vi "MotorControlMina1.vi"() -> ()   [LabVIEW 2012]
uses:
  <vilib>/Utility/error.llb/DialogType.ctl
  <vilib>/DAQmx/create/channels.llb/DAQmx Create Channel (AO-Voltage-Basic).vi
  <vilib>/DAQmx/write.llb/DAQmx Write (Analog DBL 1Chan 1Samp).vi
  <vilib>/DAQmx/create/channels.llb/DAQmx Create Channel (DO-Digital Output).vi
  <vilib>/DAQmx/write.llb/DAQmx Write (Digital Bool 1Line 1Point).vi
  <vilib>/DAQmx/create/channels.llb/DAQmx Create Channel (AI-Voltage-Basic).vi
  <vilib>/DAQmx/configure/timing.llb/DAQmx Timing (Sample Clock).vi
  <vilib>/DAQmx/read.llb/DAQmx Read (Analog 2D DBL NChan NSamp).vi
  <vilib>/Analysis/baseanly.llb/Mean (DBL).vi
  <vilib>/DAQmx/read.llb/DAQmx Read (Digital Bool 1Line 1Point).vi
  <vilib>/Utility/inputDevices.llb/joystickAcquire.vi
  <vilib>/Utility/inputDevices.llb/closeJoystick.vi
  <vilib>/Analysis/NI_AALBase.lvlib
panel:
  in  "Offset (V)":dbl=5.0
  out "Oscillate Mirror? 2":bool
  out "Mirror Voltage":dbl
  in  "Oscillate Mirror?":bool
  in  "Period (s)":i32=1
  in  "Amplitude (V)":dbl=4.0
  in  "Stop":bool
  in  "ForceExtInitConst":dbl[](array[numeric])
  out "InstrumentMode":T1(ring)=enum."Shutdown"
  in  "XMotorRef":refnum<k7>(container)
  in  "YMotorRef":refnum<k7>(container)
  in  "ZMotorRef":refnum<k7>(container)
  out "JoystOffset":T2={"XOffset"=-99999, "YOffset"=-99999, "ZOffset"=-99999}
  out "RelJoyPos":T3
  in  "InterfaceSelector":T4(tab)
  in  "GoToTopDisp":bool
  in  "GoToBottDisp":bool
  in  "GoToExpLoc":bool
  in  "SaveTopDisp":bool
  in  "SaveBottDisp":bool
  in  "SaveExpLoc":bool
  out "Top Dispenser":T5={"X Pos (mm)"=0.5532008, "Y Pos (mm)"=0.030929338, "Z Pos (mm)"=0.77973413} {"Y Pos (mm)" format="%.3f"; "Z Pos (mm)" format="%.3f"; "X Pos (mm)" format="%.3f"}
  out "Bottom Dispenser":T5={"X Pos (mm)"=0.600309, "Y Pos (mm)"=-1.1540928, "Z Pos (mm)"=0.7938141} {"Y Pos (mm)" format="%.3f"; "Z Pos (mm)" format="%.3f"; "X Pos (mm)" format="%.3f"}
  out "Experiment Region":T5={"X Pos (mm)"=1.4278219, "Y Pos (mm)"=-0.74810517, "Z Pos (mm)"=0.7938141} {"Y Pos (mm)" format="%.3f"; "Z Pos (mm)" format="%.3f"; "X Pos (mm)" format="%.3f"}
  in  "PreviewPanel":T6(tab)
  out "Diagnostic Display":cluster{dbl, dbl}(graph)={100.78259213882863, 10.649843481998925}
  out "VertReading":dbl=0.0051513671875 format="%.3f"
  out "HorizReading":dbl=0.00535888671875 format="%.3f"
  out "QPD B \n(Steerable Trap)":T7={"Horizontal Voltage (V)"=-0.009930419921875, "Vertical Voltage (V)"=-0.077978515625, "Sum Voltage (V)"=-0.056793212890625, "Horizontal Signal (NormV)"=0.17485222998387961, "Vertical Signal (NormV)"=1.3730252552391187} {"Vertical Signal (NormV)" format="%.4f"; "Horizontal Signal (NormV)" format="%#.4f"; "Sum Voltage (V)" format="%.4f"; "Vertical Voltage (V)" format="%.4f"; "Horizontal Voltage (V)" format="%.4f"}
  out "QPD A \n(Fixed Trap)":T7={"Horizontal Voltage (V)"=-0.151220703125, "Vertical Voltage (V)"=-0.02420654296875, "Sum Voltage (V)"=-0.1012939453125, "Horizontal Signal (NormV)"=1.4928898529766208, "Vertical Signal (NormV)"=0.23897324656543747} {"Vertical Signal (NormV)" format="%.4f"; "Horizontal Signal (NormV)" format="%.4f"; "Sum Voltage (V)" format="%.4f"; "Vertical Voltage (V)" format="%.4f"; "Horizontal Voltage (V)" format="%.4f"}
  in  "PreviewDataAcquision":T8={"Sampling Freq (Hz)"=2500.0, "#Samples Averaged"=50}
  in  "Trap A (Steerable)  Params":T9={"X Stiff. (pN/nm)"=0.056, "X Alpha (nm/NV)"=976.0, "X Offset (NV)"=-0.02, "Y Stiff. (pN/nm)"=0.056, "Y Alpha (nm/NV)"=976.0, "Y Offset (NV)"=0.008}
  in  "Trap B (Fixed)  Params":T9={"X Stiff. (pN/nm)"=0.063, "X Alpha (nm/NV)"=1056.0, "X Offset (NV)"=-0.022, "Y Stiff. (pN/nm)"=0.063, "Y Alpha (nm/NV)"=1056.0, "Y Offset (NV)"=-0.013}
  in  "Z Motor Settings":T10={"Joyst Min Signal"=10.0, "Joyst Max Signal"=30000.0, "Vmax (mm/s)"=0.005, "Acc (mm/s/s)"=0.2, "+ JoystDirection"=2, "- JoystDirection"=1} {"Acc (mm/s/s)" format="%#.3f"; "Vmax (mm/s)" format="%#.3f"}
  in  "Y Motor Settings":T10={"Joyst Min Signal"=10.0, "Joyst Max Signal"=20000.0, "Vmax (mm/s)"=0.03, "Acc (mm/s/s)"=0.5, "+ JoystDirection"=1, "- JoystDirection"=2} {"Acc (mm/s/s)" format="%#.3f"; "Vmax (mm/s)" format="%#.3f"}
  in  "X Motor Settings":T10={"Joyst Min Signal"=10.0, "Joyst Max Signal"=20000.0, "Vmax (mm/s)"=0.03, "Acc (mm/s/s)"=0.5, "+ JoystDirection"=2, "- JoystDirection"=1} {"Acc (mm/s/s)" format="%#.3f"; "Vmax (mm/s)" format="%#.3f"}
  in  "Motor Cruise Param":T11={"X Acc (mm/s^2)"=0.3, "X Vmax (mm/s)"=0.3, "Y Acc (mm/s^2)"=0.3, "Y Vmax (mm/s)"=0.3, "Z Acc (mm/s^2)"=0.1, "Z Vmax (mm/s)"=0.1}
  in  "Motor Limits":T12={"XMin"=-0.8, "XMax"=3.0, "YMin"=-2.0, "YMax"=2.0, "ZMin"=0.0, "ZMax"=2.0}
  in  "Steerable Mirror Calibration":T13={"Hor. Scaling (nm/V)"=760.0, "Vert. Scaling (nm/V)"=760.0, "Hor. Mirr. Offset (V)"=0.0, "Vert. Mirr. Offset (V)"=0.0}
  in  "SampRate/Ch":dbl=25000.0
  in  "AveragingWindow":i32=10
  in  "Steerable \nTrap\n(F12)":bool
  in  "Fixed\nTrap\n(F11)":bool
  in  "BMHorizSlider(V)":dbl(slide)=0.0059356689453125 scale=0.0..10.0
  in  "BMSliderVert(V)":dbl(slide)=0.005126953125 scale=0.0..10.0 scale format="%#_3f"
  in  "Align Traps Vertically":bool
  in  "MaxHorizontalTrapSeparation":bool
  out "X Motor State":T14={"Direction"=0, "Vel (mm/s)"=0.0, "IsActive?"=FALSE, "Pos (mm)"=-0.2957381} {"Pos (mm)" format="%#.3f"; "Vel (mm/s)" format="%#.4f"}
  out "Y Motor State":T14={"Direction"=0, "Vel (mm/s)"=0.0, "IsActive?"=FALSE, "Pos (mm)"=0.016441232} {"Pos (mm)" format="%#.3f"; "Vel (mm/s)" format="%#.4f"}
  out "Z Motor State":T14={"Direction"=0, "Vel (mm/s)"=0.0, "IsActive?"=FALSE, "Pos (mm)"=-0.26253498} {"Pos (mm)" format="%#.3f"; "Vel (mm/s)" format="%#.4f"}
  out "Move Z":bool
  out "Move XY":bool
  in  "MotorLoopDelay":u32=100
  out "Waveform Chart":T15(graph)={"[0]"=0.0023651123, "[1]"=0.0025787354, "[2]"=0.0019226074, "[3]"=0.0018310547, "[4]"=0.006378174, "[5]"=0.004486084, "[6]"=0.0008239746, "[7]"=0.0034179688}
  in  "StopPassiveMode":bool caption="stop"
  out "LowFreqFilePath":string="C:\\Data\\091813\\091813N02.psv"
  in  "PMVertSlider(V)":dbl(slide)=0.005145263671875 scale=0.0..10.0 scale format="%#_3f"
  in  "PMHorizSlider(V)":dbl(slide)=0.0045623779296875 scale=2.0..10.0
  out "IsPassiveModeActive?":bool caption="stop"
  out "Force TrapA":cluster{dbl, dbl}[](graph)=[{nan, nan}, {nan, nan}, {nan, nan}, {nan, nan}, {nan, nan}, {nan, nan}, {nan, nan}, {nan, nan}, {nan, nan}, {nan, nan}, {nan, nan}, {nan, nan}, {nan, nan}, {nan, nan}, {nan, nan}, {nan, nan}, {nan, nan}, {nan, nan}, {nan, nan}, {nan, nan}, {nan, nan}, {nan, nan}, {nan, nan}, {nan, nan}, {nan, nan}, {nan, nan}, {nan, nan}, {nan, nan}, {nan, nan}, {nan, nan}, {nan, nan}, {nan, nan}, {nan, nan}, {nan, nan}, {nan, nan}, {nan, nan}, {nan, nan}, {nan, nan}, {nan, nan}, {nan, nan}, {nan, nan}, {nan, nan}, {nan, nan}, {nan, nan}, {nan, nan}, {nan, nan}, {nan, nan}, {nan, nan}, {nan, nan}, {nan, nan}, {nan, nan}, {nan, nan}, {nan, nan}, {nan, nan}, {nan, nan}, {nan, nan}, {nan, nan}, {nan, nan}, {nan, nan}, {nan, nan}, {nan, nan}, {nan, nan}, {nan, nan}, {nan, nan}, {nan, nan}, {nan, nan}, {nan, nan}, {nan, nan}, {nan, nan}, {nan, nan}, {nan, nan}, {nan, nan}, {nan, nan}, {nan, nan}, {nan, nan}, {nan, nan}, {nan, nan}, {nan, nan}, {nan, nan}, {nan, nan}, {nan, nan}, {nan, nan}, {nan, nan}, {nan, nan}, {nan, nan}, {nan, nan}, {nan, nan}, {nan, nan}, {nan, nan}, {nan, nan}, {nan, nan}, {nan, nan}, {nan, nan}, {nan, nan}, {nan, nan}, {nan, nan}, {nan, nan}, {nan, nan}, {nan, nan}, {nan, nan}, {nan, nan}, {nan, nan}, {nan, nan}, {nan, nan}, {nan, nan}, {nan, nan}, {nan, nan}, {nan, nan}, {nan, nan}, {nan, nan}, {nan, nan}, {nan, nan}, {nan, nan}, {nan, nan}, {nan, nan}, {nan, nan}, {nan, nan}, {nan, nan}, {nan, nan}, {nan, nan}, {nan, nan}, {nan, nan}, {nan, nan}, {nan, nan}, {nan, nan}, {nan, nan}, {nan, nan}, {nan, nan}, {nan, nan}, {nan, nan}, {nan, nan}, {nan, nan}, {nan, nan}, {nan, nan}, {nan, nan}, {nan, nan}, {nan, nan}, {nan, nan}, {nan, nan}, {nan, nan}, {nan, nan}, {nan, nan}, {nan, nan}, {nan, nan}, {nan, nan}, {nan, nan}, {nan, nan}, {nan, nan}, {nan, nan}, {nan, nan}, {nan, nan}, {nan, nan}, {nan, nan}, {nan, nan}, {nan, nan}, {nan, nan}, {nan, nan}, {nan, nan}, {nan, nan}, {nan, nan}, {nan, nan}, {nan, nan}, {nan, nan}, {nan, nan}, {nan, nan}, {nan, nan}, {nan, nan}, {nan, nan}, {nan, nan}, {nan, nan}, {nan, nan}, {nan, nan}, {nan, nan}, {nan, nan}, {nan, nan}, {nan, nan}, {nan, nan}, {nan, nan}, {nan, nan}, {nan, nan}, {nan, nan}, {nan, nan}, {nan, nan}, {nan, nan}, {nan, nan}, {nan, nan}, {nan, nan}, {nan, nan}, {nan, nan}, {nan, nan}, {nan, nan}, {nan, nan}, {nan, nan}, {nan, nan}, {nan, nan}, {nan, nan}, {nan, nan}, {nan, nan}, {nan, nan}, {nan, nan}, {nan, nan}, {nan, nan}, {nan, nan}, {nan, nan}, {nan, nan}, {nan, nan}, {nan, nan}, {nan, nan}, {nan, nan}, {nan, nan}, {nan, nan}, {nan, nan}, {nan, nan}, {nan, nan}, {nan, nan}, {nan, nan}, {nan, nan}, {nan, nan}, {nan, nan}, {nan, nan}, {nan, nan}, {nan, nan}, {nan, nan}, {nan, nan}, {nan, nan}, {nan, nan}, {nan, nan}, {nan, nan}, {nan, nan}, {nan, nan}, {nan, nan}, {nan, nan}, {nan, nan}, {nan, nan}, {nan, nan}, {nan, nan}, {nan, nan}, {nan, nan}, {nan, nan}, {nan, nan}, {nan, nan}, {nan, nan}, {nan, nan}, {nan, nan}, {nan, nan}, {nan, nan}, {nan, nan}, {nan, nan}, {nan, nan}, {nan, nan}, {nan, nan}, {nan, nan}, {nan, nan}, {nan, nan}, {nan, nan}, {nan, nan}, {nan, nan}, {nan, nan}, {nan, nan}, {nan, nan}, {nan, nan}, {nan, nan}, {nan, nan}, {nan, nan}, {nan, nan}, {nan, nan}, {nan, nan}, {nan, nan}, {nan, nan}, {nan, nan}, {nan, nan}, {nan, nan}, {nan, nan}, {nan, nan}, {nan, nan}, {nan, nan}, {nan, nan}, {nan, nan}, {nan, nan}, {nan, nan}, {nan, nan}, {nan, nan}, {nan, nan}, {nan, nan}, {nan, nan}, {nan, nan}, {nan, nan}, {nan, nan}, {nan, nan}, {nan, nan}, {nan, nan}, {nan, nan}, {nan, nan}, {nan, nan}, {nan, nan}, {nan, nan}, {nan, nan}, {nan, nan}, {nan, nan}, {nan, nan}, {nan, nan}, {nan, nan}, {nan, nan}, {nan, nan}, {nan, nan}, {nan, nan}, {nan, nan}, {nan, nan}, {nan, nan}, {nan, nan}, {nan, nan}, {nan, nan}, {nan, nan}, {nan, nan}, {nan, nan}, {nan, nan}, {nan, nan}, {nan, nan}, {nan, nan}, {nan, nan}, {nan, nan}, {nan, nan}, {nan, nan}, {nan, nan}, {nan, nan}, {nan, nan}, {nan, nan}, {nan, nan}, {nan, nan}, {nan, nan}, {nan, nan}, {nan, nan}, {nan, nan}, {nan, nan}, {nan, nan}, {nan, nan}, {nan, nan}, {nan, nan}, {nan, nan}, {nan, nan}, {nan, nan}, {nan, nan}, {nan, nan}, {nan, nan}, {nan, nan}, {nan, nan}, {nan, nan}, {nan, nan}, {nan, nan}, {nan, nan}, {nan, nan}, {nan, nan}, {nan, nan}, {nan, nan}, {nan, nan}, {nan, nan}, {nan, nan}, {nan, nan}, {nan, nan}, {nan, nan}, {nan, nan}, {nan, nan}, {nan, nan}, {nan, nan}, {nan, nan}, {nan, nan}, {nan, nan}, {nan, nan}, {nan, nan}, {nan, nan}, {nan, nan}, {nan, nan}, {nan, nan}, {nan, nan}, {nan, nan}, {nan, nan}, {nan, nan}, {nan, nan}, {nan, nan}, {nan, nan}, {nan, nan}, {nan, nan}, {nan, nan}, {nan, nan}, {nan, nan}, {nan, nan}, {nan, nan}, {nan, nan}, {nan, nan}, {nan, nan}, {nan, nan}, {nan, nan}, {nan, nan}, {nan, nan}, {nan, nan}, {nan, nan}, {nan, nan}, {nan, nan}, {nan, nan}, {nan, nan}, {nan, nan}, {nan, nan}, {nan, nan}, {nan, nan}, {nan, nan}, {nan, nan}, {nan, nan}, {nan, nan}, {nan, nan}, {nan, nan}, {nan, nan}, {nan, nan}, {nan, nan}, {nan, nan}, {nan, nan}, {nan, nan}, {nan, nan}, {nan, nan}, {nan, nan}, {nan, nan}, {nan, nan}, {nan, nan}, {nan, nan}, {nan, nan}, {nan, nan}, {nan, nan}, {nan, nan}, {nan, nan}, {nan, nan}, {nan, nan}, {nan, nan}, {nan, nan}, {nan, nan}, {nan, nan}, {nan, nan}, {nan, nan}, {nan, nan}, {nan, nan}, {nan, nan}, {nan, nan}, {nan, nan}, {nan, nan}, {nan, nan}, {nan, nan}, {nan, nan}, {nan, nan}, {nan, nan}, {nan, nan}, {nan, nan}, {nan, nan}, {nan, nan}, {nan, nan}, {nan, nan}, {nan, nan}, {nan, nan}, {nan, nan}, {nan, nan}, {nan, nan}, {nan, nan}, {nan, nan}, {nan, nan}, {nan, nan}, {nan, nan}, {nan, nan}, {nan, nan}, {nan, nan}, {nan, nan}, {nan, nan}, {nan, nan}, {nan, nan}, {nan, nan}, {nan, nan}, {nan, nan}, {nan, nan}, {nan, nan}, {nan, nan}, {nan, nan}, {nan, nan}, {nan, nan}, {nan, nan}, {nan, nan}, {nan, nan}, {nan, nan}, {nan, nan}, {nan, nan}, {nan, nan}, {nan, nan}, {nan, nan}, {nan, nan}, {nan, nan}, {nan, nan}, {nan, nan}, {nan, nan}, {nan, nan}, {nan, nan}, {nan, nan}, {nan, nan}, {nan, nan}, {nan, nan}, {nan, nan}, {nan, nan}, {nan, nan}, {nan, nan}, {nan, nan}, {nan, nan}, {nan, nan}, {nan, nan}, {nan, nan}, {nan, nan}, {nan, nan}, {nan, nan}, {nan, nan}, {nan, nan}, {nan, nan}, {nan, nan}, {nan, nan}, {nan, nan}, {nan, nan}, {nan, nan}, {nan, nan}, {nan, nan}, {nan, nan}, {nan, nan}, {nan, nan}, {nan, nan}, {nan, nan}, {nan, nan}, {nan, nan}, {nan, nan}, {nan, nan}, {nan, nan}, {nan, nan}, {nan, nan}, {nan, nan}, {nan, nan}, {nan, nan}, {nan, nan}, {nan, nan}, {nan, nan}, {nan, nan}, {nan, nan}, {nan, nan}, {nan, nan}, {nan, nan}, {nan, nan}, {nan, nan}, {nan, nan}, {nan, nan}, {nan, nan}, {nan, nan}, {nan, nan}, {nan, nan}, {nan, nan}, {nan, nan}, {nan, nan}, {nan, nan}, {nan, nan}, {nan, nan}, {nan, nan}, {nan, nan}, {nan, nan}, {nan, nan}, {nan, nan}, {nan, nan}, {nan, nan}, {nan, nan}, {nan, nan}, {nan, nan}, {nan, nan}, {nan, nan}, {nan, nan}, {nan, nan}, {nan, nan}, {nan, nan}, {nan, nan}, {nan, nan}, {nan, nan}, {nan, nan}, {nan, nan}, {nan, nan}, {nan, nan}, {nan, nan}, {nan, nan}, {nan, nan}, {nan, nan}, {nan, nan}, {nan, nan}, {nan, nan}, {nan, nan}, {nan, nan}, {nan, nan}, {nan, nan}, {nan, nan}, {nan, nan}, {nan, nan}, {nan, nan}, {nan, nan}, {nan, nan}, {nan, nan}, {nan, nan}, {nan, nan}, {nan, nan}, {nan, nan}, {nan, nan}, {nan, nan}, {nan, nan}, {nan, nan}, {nan, nan}, {nan, nan}, {nan, nan}, {nan, nan}, {nan, nan}, {nan, nan}, {nan, nan}, {nan, nan}, {nan, nan}, {nan, nan}, {nan, nan}, {nan, nan}, {nan, nan}, {nan, nan}, {nan, nan}, {nan, nan}, {nan, nan}, {nan, nan}, {nan, nan}, {nan, nan}, {nan, nan}, {nan, nan}, {nan, nan}, {nan, nan}, {nan, nan}, {nan, nan}, {nan, nan}, {nan, nan}, {nan, nan}, {nan, nan}, {nan, nan}, {nan, nan}, {nan, nan}, {nan, nan}, {nan, nan}, {nan, nan}, {nan, nan}, {nan, nan}, {nan, nan}, {nan, nan}, {nan, nan}, {nan, nan}, {nan, nan}, {nan, nan}, {nan, nan}, {nan, nan}, {nan, nan}, {nan, nan}, {nan, nan}, {nan, nan}, {nan, nan}, {nan, nan}, {nan, nan}, {nan, nan}, {nan, nan}, {nan, nan}, {nan, nan}, {nan, nan}, {nan, nan}, {nan, nan}, {nan, nan}, {nan, nan}, {nan, nan}, {nan, nan}, {nan, nan}, {nan, nan}, {nan, nan}, {nan, nan}, {nan, nan}, {nan, nan}, {nan, nan}, {nan, nan}, {nan, nan}, {nan, nan}, {nan, nan}, {nan, nan}, {nan, nan}, {nan, nan}, {nan, nan}, {nan, nan}, {nan, nan}, {nan, nan}, {nan, nan}, {nan, nan}, {nan, nan}, {nan, nan}, {nan, nan}, {nan, nan}, {nan, nan}, {nan, nan}, {nan, nan}, {nan, nan}, {nan, nan}, {nan, nan}, {nan, nan}, {nan, nan}, {nan, nan}, {nan, nan}, {nan, nan}, {nan, nan}, {nan, nan}, {nan, nan}, {nan, nan}, {nan, nan}, {nan, nan}, {nan, nan}, {nan, nan}, {nan, nan}, {nan, nan}, {nan, nan}, {nan, nan}, {nan, nan}, {nan, nan}, {nan, nan}, {nan, nan}, {nan, nan}, {nan, nan}, {nan, nan}, {nan, nan}, {nan, nan}, {nan, nan}, {nan, nan}, {nan, nan}, {nan, nan}, {nan, nan}, {nan, nan}, {nan, nan}, {nan, nan}, {nan, nan}, {nan, nan}, {nan, nan}, {nan, nan}, {nan, nan}, {nan, nan}, {nan, nan}, {nan, nan}, {nan, nan}, {nan, nan}, {nan, nan}, {nan, nan}, {nan, nan}, {nan, nan}, {nan, nan}, {nan, nan}, {nan, nan}, {nan, nan}, {nan, nan}, {nan, nan}, {nan, nan}, {nan, nan}, {nan, nan}, {nan, nan}, {nan, nan}, {nan, nan}, {nan, nan}, {nan, nan}, {nan, nan}, {nan, nan}, {nan, nan}, {nan, nan}, {nan, nan}, {nan, nan}, {nan, nan}, {nan, nan}, {nan, nan}, {nan, nan}, {nan, nan}, {nan, nan}, {nan, nan}, {nan, nan}, {nan, nan}, {nan, nan}, {nan, nan}, {nan, nan}, {nan, nan}, {nan, nan}, {nan, nan}, {nan, nan}, {nan, nan}, {nan, nan}, {nan, nan}, {nan, nan}, {nan, nan}, {nan, nan}, {nan, nan}, {nan, nan}, {nan, nan}, {nan, nan}, {nan, nan}, {nan, nan}, {nan, nan}, {nan, nan}, {nan, nan}, {nan, nan}, {nan, nan}, {nan, nan}, {nan, nan}, {nan, nan}, {nan, nan}, {nan, nan}, {nan, nan}, {nan, nan}, {nan, nan}, {nan, nan}, {nan, nan}, {nan, nan}, {nan, nan}, {nan, nan}, {nan, nan}, {nan, nan}, {nan, nan}, {nan, nan}, {nan, nan}, {nan, nan}, {nan, nan}, {nan, nan}, {nan, nan}, {nan, nan}, {nan, nan}, {nan, nan}, {nan, nan}, {nan, nan}, {nan, nan}, {nan, nan}, {nan, nan}, {nan, nan}, {nan, nan}, {nan, nan}, {nan, nan}, {nan, nan}, {nan, nan}, {nan, nan}, {nan, nan}, {nan, nan}, {nan, nan}, {nan, nan}, {nan, nan}, {nan, nan}, {nan, nan}, {nan, nan}, {nan, nan}, {nan, nan}, {nan, nan}, {nan, nan}, {nan, nan}, {nan, nan}, {nan, nan}, {nan, nan}, {nan, nan}, {nan, nan}, {nan, nan}, {nan, nan}, {nan, nan}, {nan, nan}, {nan, nan}, {nan, nan}, {nan, nan}, {nan, nan}, {nan, nan}, {nan, nan}, {nan, nan}, {nan, nan}, {nan, nan}, {nan, nan}, {nan, nan}, {nan, nan}, {nan, nan}, {nan, nan}, {nan, nan}, {nan, nan}, {nan, nan}, {nan, nan}, {nan, nan}, {nan, nan}, {nan, nan}, {nan, nan}, {nan, nan}, {nan, nan}, {nan, nan}, {nan, nan}, {nan, nan}, {nan, nan}, {nan, nan}, {nan, nan}, {nan, nan}, {nan, nan}, {nan, nan}, {nan, nan}, {nan, nan}, {nan, nan}, {nan, nan}, {nan, nan}, {nan, nan}, {nan, nan}, {nan, nan}, {nan, nan}, {nan, nan}, {nan, nan}, {nan, nan}, {nan, nan}, {nan, nan}, {nan, nan}, {nan, nan}, {nan, nan}, {nan, nan}, {nan, nan}, {nan, nan}, {nan, nan}, {nan, nan}, {nan, nan}, {nan, nan}, {nan, nan}, {nan, nan}, {nan, nan}, {nan, nan}, {nan, nan}, {nan, nan}, {nan, nan}, {nan, nan}, {nan, nan}, {nan, nan}, {nan, nan}, {nan, nan}, {nan, nan}, {nan, nan}, {nan, nan}, {nan, nan}, {nan, nan}, {nan, nan}, {nan, nan}, {nan, nan}, {nan, nan}, {nan, nan}, {nan, nan}, {nan, nan}, {nan, nan}, {nan, nan}, {nan, nan}, {nan, nan}, {nan, nan}, {nan, nan}, {nan, nan}, {nan, nan}, {nan, nan}, {nan, nan}, {nan, nan}, {nan, nan}, {nan, nan}, {nan, nan}, {nan, nan}, {nan, nan}, {nan, nan}, {nan, nan}, {nan, nan}, {nan, nan}, {nan, nan}, {nan, nan}, {nan, nan}, {nan, nan}, {nan, nan}, {nan, nan}, {nan, nan}, {nan, nan}, {nan, nan}, {nan, nan}, {nan, nan}, {nan, nan}, {nan, nan}, {nan, nan}, {nan, nan}, {nan, nan}, {nan, nan}, {nan, nan}, {nan, nan}, {nan, nan}, {nan, nan}, {nan, nan}, {nan, nan}, {nan, nan}, {nan, nan}, {nan, nan}, {nan, nan}, {nan, nan}, {nan, nan}, {nan, nan}, {nan, nan}, {nan, nan}, {nan, nan}, {nan, nan}, {nan, nan}, {nan, nan}, {nan, nan}, {nan, nan}]
  out "Noise-Ext":cluster{dbl, dbl}[](graph)=[{nan, -0.0}, {nan, -0.0}, {nan, -0.0}, {nan, -0.0}, {nan, -0.0}, {nan, -0.0}, {nan, -0.0}, {nan, -0.0}, {nan, -0.0}, {nan, -0.0}, {nan, -0.0}, {nan, -0.0}, {nan, -0.0}, {nan, -0.0}, {nan, -0.0}, {nan, -0.0}, {nan, -0.0}, {nan, -0.0}, {nan, -0.0}, {nan, -0.0}, {nan, -0.0}, {nan, -0.0}, {nan, -0.0}, {nan, -0.0}, {nan, -0.0}, {nan, -0.0}, {nan, -0.0}, {nan, -0.0}, {nan, -0.0}, {nan, -0.0}, {nan, -0.0}, {nan, -0.0}, {nan, -0.0}, {nan, -0.0}, {nan, -0.0}, {nan, -0.0}, {nan, -0.0}, {nan, -0.0}, {nan, -0.0}, {nan, -0.0}, {nan, -0.0}, {nan, -0.0}, {nan, -0.0}, {nan, -0.0}, {nan, -0.0}, {nan, -0.0}, {nan, -0.0}, {nan, -0.0}, {nan, -0.0}, {nan, -0.0}, {nan, -0.0}, {nan, -0.0}, {nan, -0.0}, {nan, -0.0}, {nan, -0.0}, {nan, -0.0}, {nan, -0.0}, {nan, -0.0}, {nan, -0.0}, {nan, -0.0}, {nan, -0.0}, {nan, -0.0}, {nan, -0.0}, {nan, -0.0}, {nan, -0.0}, {nan, -0.0}, {nan, -0.0}, {nan, -0.0}, {nan, -0.0}, {nan, -0.0}, {nan, -0.0}, {nan, -0.0}, {nan, -0.0}, {nan, -0.0}, {nan, -0.0}, {nan, -0.0}, {nan, -0.0}, {nan, -0.0}, {nan, -0.0}, {nan, -0.0}, {nan, -0.0}, {nan, -0.0}, {nan, -0.0}, {nan, -0.0}, {nan, -0.0}, {nan, -0.0}, {nan, -0.0}, {nan, -0.0}, {nan, -0.0}, {nan, -0.0}, {nan, -0.0}, {nan, -0.0}, {nan, -0.0}, {nan, -0.0}, {nan, -0.0}, {nan, -0.0}, {nan, -0.0}, {nan, -0.0}, {nan, -0.0}, {nan, -0.0}, {nan, -0.0}, {nan, -0.0}, {nan, -0.0}, {nan, -0.0}, {nan, -0.0}, {nan, -0.0}, {nan, -0.0}, {nan, -0.0}, {nan, -0.0}, {nan, -0.0}, {nan, -0.0}, {nan, -0.0}, {nan, -0.0}, {nan, -0.0}, {nan, -0.0}, {nan, -0.0}, {nan, -0.0}, {nan, -0.0}, {nan, -0.0}, {nan, -0.0}, {nan, -0.0}, {nan, -0.0}, {nan, -0.0}, {nan, -0.0}, {nan, -0.0}, {nan, -0.0}, {nan, -0.0}, {nan, -0.0}, {nan, -0.0}, {nan, -0.0}, {nan, -0.0}, {nan, -0.0}, {nan, -0.0}, {nan, -0.0}, {nan, -0.0}, {nan, -0.0}, {nan, -0.0}, {nan, -0.0}, {nan, -0.0}, {nan, -0.0}, {nan, -0.0}, {nan, -0.0}, {nan, -0.0}, {nan, -0.0}, {nan, -0.0}, {nan, -0.0}, {nan, -0.0}, {nan, -0.0}, {nan, -0.0}, {nan, -0.0}, {nan, -0.0}, {nan, -0.0}, {nan, -0.0}, {nan, -0.0}, {nan, -0.0}, {nan, -0.0}, {nan, -0.0}, {nan, -0.0}, {nan, -0.0}, {nan, -0.0}, {nan, -0.0}, {nan, -0.0}, {nan, -0.0}, {nan, -0.0}, {nan, -0.0}, {nan, -0.0}, {nan, -0.0}, {nan, -0.0}, {nan, -0.0}, {nan, -0.0}, {nan, -0.0}, {nan, -0.0}, {nan, -0.0}, {nan, -0.0}, {nan, -0.0}, {nan, -0.0}, {nan, -0.0}, {nan, -0.0}, {nan, -0.0}, {nan, -0.0}, {nan, -0.0}, {nan, -0.0}, {nan, -0.0}, {nan, -0.0}, {nan, -0.0}, {nan, -0.0}, {nan, -0.0}, {nan, -0.0}, {nan, -0.0}, {nan, -0.0}, {nan, -0.0}, {nan, -0.0}, {nan, -0.0}, {nan, -0.0}, {nan, -0.0}, {nan, -0.0}, {nan, -0.0}, {nan, -0.0}, {nan, -0.0}, {nan, -0.0}, {nan, -0.0}, {nan, -0.0}, {nan, -0.0}, {nan, -0.0}, {nan, -0.0}, {nan, -0.0}, {nan, -0.0}, {nan, -0.0}, {nan, -0.0}, {nan, -0.0}, {nan, -0.0}, {nan, -0.0}, {nan, -0.0}, {nan, -0.0}, {nan, -0.0}, {nan, -0.0}, {nan, -0.0}, {nan, -0.0}, {nan, -0.0}, {nan, -0.0}, {nan, -0.0}, {nan, -0.0}, {nan, -0.0}, {nan, -0.0}, {nan, -0.0}, {nan, -0.0}, {nan, -0.0}, {nan, -0.0}, {nan, -0.0}, {nan, -0.0}, {nan, -0.0}, {nan, -0.0}, {nan, -0.0}, {nan, -0.0}, {nan, -0.0}, {nan, -0.0}, {nan, -0.0}, {nan, -0.0}, {nan, -0.0}, {nan, -0.0}, {nan, -0.0}, {nan, -0.0}, {nan, -0.0}, {nan, -0.0}, {nan, -0.0}, {nan, -0.0}, {nan, -0.0}, {nan, -0.0}, {nan, -0.0}, {nan, -0.0}, {nan, -0.0}, {nan, -0.0}, {nan, -0.0}, {nan, -0.0}, {nan, -0.0}, {nan, -0.0}, {nan, -0.0}, {nan, -0.0}, {nan, -0.0}, {nan, -0.0}, {nan, -0.0}, {nan, -0.0}, {nan, -0.0}, {nan, -0.0}, {nan, -0.0}, {nan, -0.0}, {nan, -0.0}, {nan, -0.0}, {nan, -0.0}, {nan, -0.0}, {nan, -0.0}, {nan, -0.0}, {nan, -0.0}, {nan, -0.0}, {nan, -0.0}, {nan, -0.0}, {nan, -0.0}, {nan, -0.0}, {nan, -0.0}, {nan, -0.0}, {nan, -0.0}, {nan, -0.0}, {nan, -0.0}, {nan, -0.0}, {nan, -0.0}, {nan, -0.0}, {nan, -0.0}, {nan, -0.0}, {nan, -0.0}, {nan, -0.0}, {nan, -0.0}, {nan, -0.0}, {nan, -0.0}, {nan, -0.0}, {nan, -0.0}, {nan, -0.0}, {nan, -0.0}, {nan, -0.0}, {nan, -0.0}, {nan, -0.0}, {nan, -0.0}, {nan, -0.0}, {nan, -0.0}, {nan, -0.0}, {nan, -0.0}, {nan, -0.0}, {nan, -0.0}, {nan, -0.0}, {nan, -0.0}, {nan, -0.0}, {nan, -0.0}, {nan, -0.0}, {nan, -0.0}, {nan, -0.0}, {nan, -0.0}, {nan, -0.0}, {nan, -0.0}, {nan, -0.0}, {nan, -0.0}, {nan, -0.0}, {nan, -0.0}, {nan, -0.0}, {nan, -0.0}, {nan, -0.0}, {nan, -0.0}, {nan, -0.0}, {nan, -0.0}, {nan, -0.0}, {nan, -0.0}, {nan, -0.0}, {nan, -0.0}, {nan, -0.0}, {nan, -0.0}, {nan, -0.0}, {nan, -0.0}, {nan, -0.0}, {nan, -0.0}, {nan, -0.0}, {nan, -0.0}, {nan, -0.0}, {nan, -0.0}, {nan, -0.0}, {nan, -0.0}, {nan, -0.0}, {nan, -0.0}, {nan, -0.0}, {nan, -0.0}, {nan, -0.0}, {nan, -0.0}, {nan, -0.0}, {nan, -0.0}, {nan, -0.0}, {nan, -0.0}, {nan, -0.0}, {nan, -0.0}, {nan, -0.0}, {nan, -0.0}, {nan, -0.0}, {nan, -0.0}, {nan, -0.0}, {nan, -0.0}, {nan, -0.0}, {nan, -0.0}, {nan, -0.0}, {nan, -0.0}, {nan, -0.0}, {nan, -0.0}, {nan, -0.0}, {nan, -0.0}, {nan, -0.0}, {nan, -0.0}, {nan, -0.0}, {nan, -0.0}, {nan, -0.0}, {nan, -0.0}, {nan, -0.0}, {nan, -0.0}, {nan, -0.0}, {nan, -0.0}, {nan, -0.0}, {nan, -0.0}, {nan, -0.0}, {nan, -0.0}, {nan, -0.0}, {nan, -0.0}, {nan, -0.0}, {nan, -0.0}, {nan, -0.0}, {nan, -0.0}, {nan, -0.0}, {nan, -0.0}, {nan, -0.0}, {nan, -0.0}, {nan, -0.0}, {nan, -0.0}, {nan, -0.0}, {nan, -0.0}, {nan, -0.0}, {nan, -0.0}, {nan, -0.0}, {nan, -0.0}, {nan, -0.0}, {nan, -0.0}, {nan, -0.0}, {nan, -0.0}, {nan, -0.0}, {nan, -0.0}, {nan, -0.0}, {nan, -0.0}, {nan, -0.0}, {nan, -0.0}, {nan, -0.0}, {nan, -0.0}, {nan, -0.0}, {nan, -0.0}, {nan, -0.0}, {nan, -0.0}, {nan, -0.0}, {nan, -0.0}, {nan, -0.0}, {nan, -0.0}, {nan, -0.0}, {nan, -0.0}, {nan, -0.0}, {nan, -0.0}, {nan, -0.0}, {nan, -0.0}, {nan, -0.0}, {nan, -0.0}, {nan, -0.0}, {nan, -0.0}, {nan, -0.0}, {nan, -0.0}, {nan, -0.0}, {nan, -0.0}, {nan, -0.0}, {nan, -0.0}, {nan, -0.0}, {nan, -0.0}, {nan, -0.0}, {nan, -0.0}, {nan, -0.0}, {nan, -0.0}, {nan, -0.0}, {nan, -0.0}, {nan, -0.0}, {nan, -0.0}, {nan, -0.0}, {nan, -0.0}, {nan, -0.0}, {nan, -0.0}, {nan, -0.0}, {nan, -0.0}, {nan, -0.0}, {nan, -0.0}, {nan, -0.0}, {nan, -0.0}, {nan, -0.0}, {nan, -0.0}, {nan, -0.0}, {nan, -0.0}, {nan, -0.0}, {nan, -0.0}, {nan, -0.0}, {nan, -0.0}, {nan, -0.0}, {nan, -0.0}, {nan, -0.0}, {nan, -0.0}, {nan, -0.0}, {nan, -0.0}, {nan, -0.0}, {nan, -0.0}, {nan, -0.0}, {nan, -0.0}, {nan, -0.0}, {nan, -0.0}, {nan, -0.0}, {nan, -0.0}, {nan, -0.0}, {nan, -0.0}, {nan, -0.0}, {nan, -0.0}, {nan, -0.0}, {nan, -0.0}, {nan, -0.0}, {nan, -0.0}, {nan, -0.0}, {nan, -0.0}, {nan, -0.0}, {nan, -0.0}, {nan, -0.0}, {nan, -0.0}, {nan, -0.0}, {nan, -0.0}, {nan, -0.0}, {nan, -0.0}, {nan, -0.0}, {nan, -0.0}, {nan, -0.0}, {nan, -0.0}, {nan, -0.0}, {nan, -0.0}, {nan, -0.0}, {nan, -0.0}, {nan, -0.0}, {nan, -0.0}, {nan, -0.0}, {nan, -0.0}, {nan, -0.0}, {nan, -0.0}, {nan, -0.0}, {nan, -0.0}, {nan, -0.0}, {nan, -0.0}, {nan, -0.0}, {nan, -0.0}, {nan, -0.0}, {nan, -0.0}, {nan, -0.0}, {nan, -0.0}, {nan, -0.0}, {nan, -0.0}, {nan, -0.0}, {nan, -0.0}, {nan, -0.0}, {nan, -0.0}, {nan, -0.0}, {nan, -0.0}, {nan, -0.0}, {nan, -0.0}, {nan, -0.0}, {nan, -0.0}, {nan, -0.0}, {nan, -0.0}, {nan, -0.0}, {nan, -0.0}, {nan, -0.0}, {nan, -0.0}, {nan, -0.0}, {nan, -0.0}, {nan, -0.0}, {nan, -0.0}, {nan, -0.0}, {nan, -0.0}, {nan, -0.0}, {nan, -0.0}, {nan, -0.0}, {nan, -0.0}, {nan, -0.0}, {nan, -0.0}, {nan, -0.0}, {nan, -0.0}, {nan, -0.0}, {nan, -0.0}, {nan, -0.0}, {nan, -0.0}, {nan, -0.0}, {nan, -0.0}, {nan, -0.0}, {nan, -0.0}, {nan, -0.0}, {nan, -0.0}, {nan, -0.0}, {nan, -0.0}, {nan, -0.0}, {nan, -0.0}, {nan, -0.0}, {nan, -0.0}, {nan, -0.0}, {nan, -0.0}, {nan, -0.0}, {nan, -0.0}, {nan, -0.0}, {nan, -0.0}, {nan, -0.0}, {nan, -0.0}, {nan, -0.0}, {nan, -0.0}, {nan, -0.0}, {nan, -0.0}, {nan, -0.0}, {nan, -0.0}, {nan, -0.0}, {nan, -0.0}, {nan, -0.0}, {nan, -0.0}, {nan, -0.0}, {nan, -0.0}, {nan, -0.0}, {nan, -0.0}, {nan, -0.0}, {nan, -0.0}, {nan, -0.0}, {nan, -0.0}, {nan, -0.0}, {nan, -0.0}, {nan, -0.0}, {nan, -0.0}, {nan, -0.0}, {nan, -0.0}, {nan, -0.0}, {nan, -0.0}, {nan, -0.0}, {nan, -0.0}, {nan, -0.0}, {nan, -0.0}, {nan, -0.0}, {nan, -0.0}, {nan, -0.0}, {nan, -0.0}, {nan, -0.0}, {nan, -0.0}, {nan, -0.0}, {nan, -0.0}, {nan, -0.0}, {nan, -0.0}, {nan, -0.0}, {nan, -0.0}, {nan, -0.0}, {nan, -0.0}, {nan, -0.0}, {nan, -0.0}, {nan, -0.0}, {nan, -0.0}, {nan, -0.0}, {nan, -0.0}, {nan, -0.0}, {nan, -0.0}, {nan, -0.0}, {nan, -0.0}, {nan, -0.0}, {nan, -0.0}, {nan, -0.0}, {nan, -0.0}, {nan, -0.0}, {nan, -0.0}, {nan, -0.0}, {nan, -0.0}, {nan, -0.0}, {nan, -0.0}, {nan, -0.0}, {nan, -0.0}, {nan, -0.0}, {nan, -0.0}, {nan, -0.0}, {nan, -0.0}, {nan, -0.0}, {nan, -0.0}, {nan, -0.0}, {nan, -0.0}, {nan, -0.0}, {nan, -0.0}, {nan, -0.0}, {nan, -0.0}, {nan, -0.0}, {nan, -0.0}, {nan, -0.0}, {nan, -0.0}, {nan, -0.0}, {nan, -0.0}, {nan, -0.0}, {nan, -0.0}, {nan, -0.0}, {nan, -0.0}, {nan, -0.0}, {nan, -0.0}, {nan, -0.0}, {nan, -0.0}, {nan, -0.0}, {nan, -0.0}, {nan, -0.0}, {nan, -0.0}, {nan, -0.0}, {nan, -0.0}, {nan, -0.0}, {nan, -0.0}, {nan, -0.0}, {nan, -0.0}, {nan, -0.0}, {nan, -0.0}, {nan, -0.0}, {nan, -0.0}, {nan, -0.0}, {nan, -0.0}, {nan, -0.0}, {nan, -0.0}, {nan, -0.0}, {nan, -0.0}, {nan, -0.0}, {nan, -0.0}, {nan, -0.0}, {nan, -0.0}, {nan, -0.0}, {nan, -0.0}, {nan, -0.0}, {nan, -0.0}, {nan, -0.0}, {nan, -0.0}, {nan, -0.0}, {nan, -0.0}, {nan, -0.0}, {nan, -0.0}, {nan, -0.0}, {nan, -0.0}, {nan, -0.0}, {nan, -0.0}, {nan, -0.0}, {nan, -0.0}, {nan, -0.0}, {nan, -0.0}, {nan, -0.0}, {nan, -0.0}, {nan, -0.0}, {nan, -0.0}, {nan, -0.0}, {nan, -0.0}, {nan, -0.0}, {nan, -0.0}, {nan, -0.0}, {nan, -0.0}, {nan, -0.0}, {nan, -0.0}, {nan, -0.0}, {nan, -0.0}, {nan, -0.0}, {nan, -0.0}, {nan, -0.0}, {nan, -0.0}, {nan, -0.0}, {nan, -0.0}, {nan, -0.0}, {nan, -0.0}, {nan, -0.0}, {nan, -0.0}, {nan, -0.0}, {nan, -0.0}, {nan, -0.0}, {nan, -0.0}, {nan, -0.0}, {nan, -0.0}, {nan, -0.0}, {nan, -0.0}, {nan, -0.0}, {nan, -0.0}, {nan, -0.0}, {nan, -0.0}, {nan, -0.0}, {nan, -0.0}, {nan, -0.0}, {nan, -0.0}, {nan, -0.0}, {nan, -0.0}, {nan, -0.0}, {nan, -0.0}, {nan, -0.0}, {nan, -0.0}, {nan, -0.0}, {nan, -0.0}, {nan, -0.0}, {nan, -0.0}, {nan, -0.0}, {nan, -0.0}, {nan, -0.0}, {nan, -0.0}, {nan, -0.0}, {nan, -0.0}, {nan, -0.0}, {nan, -0.0}, {nan, -0.0}, {nan, -0.0}, {nan, -0.0}, {nan, -0.0}, {nan, -0.0}, {nan, -0.0}, {nan, -0.0}, {nan, -0.0}, {nan, -0.0}, {nan, -0.0}, {nan, -0.0}, {nan, -0.0}, {nan, -0.0}, {nan, -0.0}, {nan, -0.0}, {nan, -0.0}, {nan, -0.0}, {nan, -0.0}, {nan, -0.0}, {nan, -0.0}, {nan, -0.0}, {nan, -0.0}, {nan, -0.0}, {nan, -0.0}, {nan, -0.0}, {nan, -0.0}, {nan, -0.0}, {nan, -0.0}, {nan, -0.0}, {nan, -0.0}, {nan, -0.0}, {nan, -0.0}, {nan, -0.0}, {nan, -0.0}, {nan, -0.0}, {nan, -0.0}, {nan, -0.0}, {nan, -0.0}, {nan, -0.0}, {nan, -0.0}, {nan, -0.0}, {nan, -0.0}, {nan, -0.0}, {nan, -0.0}, {nan, -0.0}, {nan, -0.0}, {nan, -0.0}, {nan, -0.0}, {nan, -0.0}, {nan, -0.0}, {nan, -0.0}, {nan, -0.0}, {nan, -0.0}, {nan, -0.0}, {nan, -0.0}, {nan, -0.0}, {nan, -0.0}, {nan, -0.0}, {nan, -0.0}, {nan, -0.0}, {nan, -0.0}, {nan, -0.0}, {nan, -0.0}, {nan, -0.0}, {nan, -0.0}, {nan, -0.0}, {nan, -0.0}, {nan, -0.0}, {nan, -0.0}, {nan, -0.0}, {nan, -0.0}, {nan, -0.0}, {nan, -0.0}, {nan, -0.0}, {nan, -0.0}, {nan, -0.0}, {nan, -0.0}, {nan, -0.0}, {nan, -0.0}, {nan, -0.0}, {nan, -0.0}, {nan, -0.0}, {nan, -0.0}, {nan, -0.0}, {nan, -0.0}, {nan, -0.0}, {nan, -0.0}, {nan, -0.0}, {nan, -0.0}, {nan, -0.0}, {nan, -0.0}, {nan, -0.0}, {nan, -0.0}, {nan, -0.0}, {nan, -0.0}, {nan, -0.0}, {nan, -0.0}, {nan, -0.0}, {nan, -0.0}, {nan, -0.0}, {nan, -0.0}, {nan, -0.0}, {nan, -0.0}, {nan, -0.0}, {nan, -0.0}, {nan, -0.0}, {nan, -0.0}, {nan, -0.0}, {nan, -0.0}, {nan, -0.0}, {nan, -0.0}, {nan, -0.0}, {nan, -0.0}, {nan, -0.0}, {nan, -0.0}, {nan, -0.0}, {nan, -0.0}, {nan, -0.0}, {nan, -0.0}, {nan, -0.0}, {nan, -0.0}, {nan, -0.0}, {nan, -0.0}, {nan, -0.0}, {nan, -0.0}, {nan, -0.0}, {nan, -0.0}, {nan, -0.0}, {nan, -0.0}, {nan, -0.0}, {nan, -0.0}, {nan, -0.0}, {nan, -0.0}, {nan, -0.0}, {nan, -0.0}, {nan, -0.0}, {nan, -0.0}, {nan, -0.0}, {nan, -0.0}, {nan, -0.0}, {nan, -0.0}, {nan, -0.0}, {nan, -0.0}, {nan, -0.0}, {nan, -0.0}, {nan, -0.0}, {nan, -0.0}, {nan, -0.0}, {nan, -0.0}, {nan, -0.0}, {nan, -0.0}, {nan, -0.0}, {nan, -0.0}, {nan, -0.0}, {nan, -0.0}, {nan, -0.0}, {nan, -0.0}, {nan, -0.0}, {nan, -0.0}, {nan, -0.0}, {nan, -0.0}, {nan, -0.0}, {nan, -0.0}, {nan, -0.0}, {nan, -0.0}, {nan, -0.0}, {nan, -0.0}, {nan, -0.0}, {nan, -0.0}, {nan, -0.0}, {nan, -0.0}, {nan, -0.0}, {nan, -0.0}, {nan, -0.0}, {nan, -0.0}, {nan, -0.0}, {nan, -0.0}, {nan, -0.0}, {nan, -0.0}, {nan, -0.0}, {nan, -0.0}, {nan, -0.0}, {nan, -0.0}, {nan, -0.0}, {nan, -0.0}, {nan, -0.0}, {nan, -0.0}, {nan, -0.0}, {nan, -0.0}, {nan, -0.0}, {nan, -0.0}, {nan, -0.0}, {nan, -0.0}, {nan, -0.0}, {nan, -0.0}, {nan, -0.0}, {nan, -0.0}, {nan, -0.0}, {nan, -0.0}, {nan, -0.0}, {nan, -0.0}, {nan, -0.0}, {nan, -0.0}, {nan, -0.0}, {nan, -0.0}, {nan, -0.0}, {nan, -0.0}, {nan, -0.0}, {nan, -0.0}, {nan, -0.0}, {nan, -0.0}, {nan, -0.0}, {nan, -0.0}, {nan, -0.0}, {nan, -0.0}, {nan, -0.0}, {nan, -0.0}, {nan, -0.0}, {nan, -0.0}, {nan, -0.0}, {nan, -0.0}, {nan, -0.0}, {nan, -0.0}, {nan, -0.0}, {nan, -0.0}, {nan, -0.0}, {nan, -0.0}, {nan, -0.0}, {nan, -0.0}, {nan, -0.0}, {nan, -0.0}]
  out "Force TrapB":cluster{dbl, dbl}[](graph)=[{nan, nan}, {nan, nan}, {nan, nan}, {nan, nan}, {nan, nan}, {nan, nan}, {nan, nan}, {nan, nan}, {nan, nan}, {nan, nan}, {nan, nan}, {nan, nan}, {nan, nan}, {nan, nan}, {nan, nan}, {nan, nan}, {nan, nan}, {nan, nan}, {nan, nan}, {nan, nan}, {nan, nan}, {nan, nan}, {nan, nan}, {nan, nan}, {nan, nan}, {nan, nan}, {nan, nan}, {nan, nan}, {nan, nan}, {nan, nan}, {nan, nan}, {nan, nan}, {nan, nan}, {nan, nan}, {nan, nan}, {nan, nan}, {nan, nan}, {nan, nan}, {nan, nan}, {nan, nan}, {nan, nan}, {nan, nan}, {nan, nan}, {nan, nan}, {nan, nan}, {nan, nan}, {nan, nan}, {nan, nan}, {nan, nan}, {nan, nan}, {nan, nan}, {nan, nan}, {nan, nan}, {nan, nan}, {nan, nan}, {nan, nan}, {nan, nan}, {nan, nan}, {nan, nan}, {nan, nan}, {nan, nan}, {nan, nan}, {nan, nan}, {nan, nan}, {nan, nan}, {nan, nan}, {nan, nan}, {nan, nan}, {nan, nan}, {nan, nan}, {nan, nan}, {nan, nan}, {nan, nan}, {nan, nan}, {nan, nan}, {nan, nan}, {nan, nan}, {nan, nan}, {nan, nan}, {nan, nan}, {nan, nan}, {nan, nan}, {nan, nan}, {nan, nan}, {nan, nan}, {nan, nan}, {nan, nan}, {nan, nan}, {nan, nan}, {nan, nan}, {nan, nan}, {nan, nan}, {nan, nan}, {nan, nan}, {nan, nan}, {nan, nan}, {nan, nan}, {nan, nan}, {nan, nan}, {nan, nan}, {nan, nan}, {nan, nan}, {nan, nan}, {nan, nan}, {nan, nan}, {nan, nan}, {nan, nan}, {nan, nan}, {nan, nan}, {nan, nan}, {nan, nan}, {nan, nan}, {nan, nan}, {nan, nan}, {nan, nan}, {nan, nan}, {nan, nan}, {nan, nan}, {nan, nan}, {nan, nan}, {nan, nan}, {nan, nan}, {nan, nan}, {nan, nan}, {nan, nan}, {nan, nan}, {nan, nan}, {nan, nan}, {nan, nan}, {nan, nan}, {nan, nan}, {nan, nan}, {nan, nan}, {nan, nan}, {nan, nan}, {nan, nan}, {nan, nan}, {nan, nan}, {nan, nan}, {nan, nan}, {nan, nan}, {nan, nan}, {nan, nan}, {nan, nan}, {nan, nan}, {nan, nan}, {nan, nan}, {nan, nan}, {nan, nan}, {nan, nan}, {nan, nan}, {nan, nan}, {nan, nan}, {nan, nan}, {nan, nan}, {nan, nan}, {nan, nan}, {nan, nan}, {nan, nan}, {nan, nan}, {nan, nan}, {nan, nan}, {nan, nan}, {nan, nan}, {nan, nan}, {nan, nan}, {nan, nan}, {nan, nan}, {nan, nan}, {nan, nan}, {nan, nan}, {nan, nan}, {nan, nan}, {nan, nan}, {nan, nan}, {nan, nan}, {nan, nan}, {nan, nan}, {nan, nan}, {nan, nan}, {nan, nan}, {nan, nan}, {nan, nan}, {nan, nan}, {nan, nan}, {nan, nan}, {nan, nan}, {nan, nan}, {nan, nan}, {nan, nan}, {nan, nan}, {nan, nan}, {nan, nan}, {nan, nan}, {nan, nan}, {nan, nan}, {nan, nan}, {nan, nan}, {nan, nan}, {nan, nan}, {nan, nan}, {nan, nan}, {nan, nan}, {nan, nan}, {nan, nan}, {nan, nan}, {nan, nan}, {nan, nan}, {nan, nan}, {nan, nan}, {nan, nan}, {nan, nan}, {nan, nan}, {nan, nan}, {nan, nan}, {nan, nan}, {nan, nan}, {nan, nan}, {nan, nan}, {nan, nan}, {nan, nan}, {nan, nan}, {nan, nan}, {nan, nan}, {nan, nan}, {nan, nan}, {nan, nan}, {nan, nan}, {nan, nan}, {nan, nan}, {nan, nan}, {nan, nan}, {nan, nan}, {nan, nan}, {nan, nan}, {nan, nan}, {nan, nan}, {nan, nan}, {nan, nan}, {nan, nan}, {nan, nan}, {nan, nan}, {nan, nan}, {nan, nan}, {nan, nan}, {nan, nan}, {nan, nan}, {nan, nan}, {nan, nan}, {nan, nan}, {nan, nan}, {nan, nan}, {nan, nan}, {nan, nan}, {nan, nan}, {nan, nan}, {nan, nan}, {nan, nan}, {nan, nan}, {nan, nan}, {nan, nan}, {nan, nan}, {nan, nan}, {nan, nan}, {nan, nan}, {nan, nan}, {nan, nan}, {nan, nan}, {nan, nan}, {nan, nan}, {nan, nan}, {nan, nan}, {nan, nan}, {nan, nan}, {nan, nan}, {nan, nan}, {nan, nan}, {nan, nan}, {nan, nan}, {nan, nan}, {nan, nan}, {nan, nan}, {nan, nan}, {nan, nan}, {nan, nan}, {nan, nan}, {nan, nan}, {nan, nan}, {nan, nan}, {nan, nan}, {nan, nan}, {nan, nan}, {nan, nan}, {nan, nan}, {nan, nan}, {nan, nan}, {nan, nan}, {nan, nan}, {nan, nan}, {nan, nan}, {nan, nan}, {nan, nan}, {nan, nan}, {nan, nan}, {nan, nan}, {nan, nan}, {nan, nan}, {nan, nan}, {nan, nan}, {nan, nan}, {nan, nan}, {nan, nan}, {nan, nan}, {nan, nan}, {nan, nan}, {nan, nan}, {nan, nan}, {nan, nan}, {nan, nan}, {nan, nan}, {nan, nan}, {nan, nan}, {nan, nan}, {nan, nan}, {nan, nan}, {nan, nan}, {nan, nan}, {nan, nan}, {nan, nan}, {nan, nan}, {nan, nan}, {nan, nan}, {nan, nan}, {nan, nan}, {nan, nan}, {nan, nan}, {nan, nan}, {nan, nan}, {nan, nan}, {nan, nan}, {nan, nan}, {nan, nan}, {nan, nan}, {nan, nan}, {nan, nan}, {nan, nan}, {nan, nan}, {nan, nan}, {nan, nan}, {nan, nan}, {nan, nan}, {nan, nan}, {nan, nan}, {nan, nan}, {nan, nan}, {nan, nan}, {nan, nan}, {nan, nan}, {nan, nan}, {nan, nan}, {nan, nan}, {nan, nan}, {nan, nan}, {nan, nan}, {nan, nan}, {nan, nan}, {nan, nan}, {nan, nan}, {nan, nan}, {nan, nan}, {nan, nan}, {nan, nan}, {nan, nan}, {nan, nan}, {nan, nan}, {nan, nan}, {nan, nan}, {nan, nan}, {nan, nan}, {nan, nan}, {nan, nan}, {nan, nan}, {nan, nan}, {nan, nan}, {nan, nan}, {nan, nan}, {nan, nan}, {nan, nan}, {nan, nan}, {nan, nan}, {nan, nan}, {nan, nan}, {nan, nan}, {nan, nan}, {nan, nan}, {nan, nan}, {nan, nan}, {nan, nan}, {nan, nan}, {nan, nan}, {nan, nan}, {nan, nan}, {nan, nan}, {nan, nan}, {nan, nan}, {nan, nan}, {nan, nan}, {nan, nan}, {nan, nan}, {nan, nan}, {nan, nan}, {nan, nan}, {nan, nan}, {nan, nan}, {nan, nan}, {nan, nan}, {nan, nan}, {nan, nan}, {nan, nan}, {nan, nan}, {nan, nan}, {nan, nan}, {nan, nan}, {nan, nan}, {nan, nan}, {nan, nan}, {nan, nan}, {nan, nan}, {nan, nan}, {nan, nan}, {nan, nan}, {nan, nan}, {nan, nan}, {nan, nan}, {nan, nan}, {nan, nan}, {nan, nan}, {nan, nan}, {nan, nan}, {nan, nan}, {nan, nan}, {nan, nan}, {nan, nan}, {nan, nan}, {nan, nan}, {nan, nan}, {nan, nan}, {nan, nan}, {nan, nan}, {nan, nan}, {nan, nan}, {nan, nan}, {nan, nan}, {nan, nan}, {nan, nan}, {nan, nan}, {nan, nan}, {nan, nan}, {nan, nan}, {nan, nan}, {nan, nan}, {nan, nan}, {nan, nan}, {nan, nan}, {nan, nan}, {nan, nan}, {nan, nan}, {nan, nan}, {nan, nan}, {nan, nan}, {nan, nan}, {nan, nan}, {nan, nan}, {nan, nan}, {nan, nan}, {nan, nan}, {nan, nan}, {nan, nan}, {nan, nan}, {nan, nan}, {nan, nan}, {nan, nan}, {nan, nan}, {nan, nan}, {nan, nan}, {nan, nan}, {nan, nan}, {nan, nan}, {nan, nan}, {nan, nan}, {nan, nan}, {nan, nan}, {nan, nan}, {nan, nan}, {nan, nan}, {nan, nan}, {nan, nan}, {nan, nan}, {nan, nan}, {nan, nan}, {nan, nan}, {nan, nan}, {nan, nan}, {nan, nan}, {nan, nan}, {nan, nan}, {nan, nan}, {nan, nan}, {nan, nan}, {nan, nan}, {nan, nan}, {nan, nan}, {nan, nan}, {nan, nan}, {nan, nan}, {nan, nan}, {nan, nan}, {nan, nan}, {nan, nan}, {nan, nan}, {nan, nan}, {nan, nan}, {nan, nan}, {nan, nan}, {nan, nan}, {nan, nan}, {nan, nan}, {nan, nan}, {nan, nan}, {nan, nan}, {nan, nan}, {nan, nan}, {nan, nan}, {nan, nan}, {nan, nan}, {nan, nan}, {nan, nan}, {nan, nan}, {nan, nan}, {nan, nan}, {nan, nan}, {nan, nan}, {nan, nan}, {nan, nan}, {nan, nan}, {nan, nan}, {nan, nan}, {nan, nan}, {nan, nan}, {nan, nan}, {nan, nan}, {nan, nan}, {nan, nan}, {nan, nan}, {nan, nan}, {nan, nan}, {nan, nan}, {nan, nan}, {nan, nan}, {nan, nan}, {nan, nan}, {nan, nan}, {nan, nan}, {nan, nan}, {nan, nan}, {nan, nan}, {nan, nan}, {nan, nan}, {nan, nan}, {nan, nan}, {nan, nan}, {nan, nan}, {nan, nan}, {nan, nan}, {nan, nan}, {nan, nan}, {nan, nan}, {nan, nan}, {nan, nan}, {nan, nan}, {nan, nan}, {nan, nan}, {nan, nan}, {nan, nan}, {nan, nan}, {nan, nan}, {nan, nan}, {nan, nan}, {nan, nan}, {nan, nan}, {nan, nan}, {nan, nan}, {nan, nan}, {nan, nan}, {nan, nan}, {nan, nan}, {nan, nan}, {nan, nan}, {nan, nan}, {nan, nan}, {nan, nan}, {nan, nan}, {nan, nan}, {nan, nan}, {nan, nan}, {nan, nan}, {nan, nan}, {nan, nan}, {nan, nan}, {nan, nan}, {nan, nan}, {nan, nan}, {nan, nan}, {nan, nan}, {nan, nan}, {nan, nan}, {nan, nan}, {nan, nan}, {nan, nan}, {nan, nan}, {nan, nan}, {nan, nan}, {nan, nan}, {nan, nan}, {nan, nan}, {nan, nan}, {nan, nan}, {nan, nan}, {nan, nan}, {nan, nan}, {nan, nan}, {nan, nan}, {nan, nan}, {nan, nan}, {nan, nan}, {nan, nan}, {nan, nan}, {nan, nan}, {nan, nan}, {nan, nan}, {nan, nan}, {nan, nan}, {nan, nan}, {nan, nan}, {nan, nan}, {nan, nan}, {nan, nan}, {nan, nan}, {nan, nan}, {nan, nan}, {nan, nan}, {nan, nan}, {nan, nan}, {nan, nan}, {nan, nan}, {nan, nan}, {nan, nan}, {nan, nan}, {nan, nan}, {nan, nan}, {nan, nan}, {nan, nan}, {nan, nan}, {nan, nan}, {nan, nan}, {nan, nan}, {nan, nan}, {nan, nan}, {nan, nan}, {nan, nan}, {nan, nan}, {nan, nan}, {nan, nan}, {nan, nan}, {nan, nan}, {nan, nan}, {nan, nan}, {nan, nan}, {nan, nan}, {nan, nan}, {nan, nan}, {nan, nan}, {nan, nan}, {nan, nan}, {nan, nan}, {nan, nan}, {nan, nan}, {nan, nan}, {nan, nan}, {nan, nan}, {nan, nan}, {nan, nan}, {nan, nan}, {nan, nan}, {nan, nan}, {nan, nan}, {nan, nan}, {nan, nan}, {nan, nan}, {nan, nan}, {nan, nan}, {nan, nan}, {nan, nan}, {nan, nan}, {nan, nan}, {nan, nan}, {nan, nan}, {nan, nan}, {nan, nan}, {nan, nan}, {nan, nan}, {nan, nan}, {nan, nan}, {nan, nan}, {nan, nan}, {nan, nan}, {nan, nan}, {nan, nan}, {nan, nan}, {nan, nan}, {nan, nan}, {nan, nan}, {nan, nan}, {nan, nan}, {nan, nan}, {nan, nan}, {nan, nan}, {nan, nan}, {nan, nan}, {nan, nan}, {nan, nan}, {nan, nan}, {nan, nan}, {nan, nan}, {nan, nan}, {nan, nan}, {nan, nan}, {nan, nan}, {nan, nan}, {nan, nan}, {nan, nan}, {nan, nan}, {nan, nan}, {nan, nan}, {nan, nan}, {nan, nan}, {nan, nan}, {nan, nan}, {nan, nan}, {nan, nan}, {nan, nan}, {nan, nan}, {nan, nan}, {nan, nan}, {nan, nan}, {nan, nan}, {nan, nan}, {nan, nan}, {nan, nan}, {nan, nan}, {nan, nan}, {nan, nan}, {nan, nan}, {nan, nan}, {nan, nan}, {nan, nan}, {nan, nan}, {nan, nan}, {nan, nan}, {nan, nan}, {nan, nan}, {nan, nan}, {nan, nan}, {nan, nan}, {nan, nan}, {nan, nan}, {nan, nan}, {nan, nan}, {nan, nan}, {nan, nan}, {nan, nan}, {nan, nan}, {nan, nan}, {nan, nan}, {nan, nan}, {nan, nan}, {nan, nan}, {nan, nan}, {nan, nan}, {nan, nan}, {nan, nan}, {nan, nan}, {nan, nan}, {nan, nan}, {nan, nan}, {nan, nan}, {nan, nan}, {nan, nan}, {nan, nan}, {nan, nan}, {nan, nan}, {nan, nan}, {nan, nan}, {nan, nan}, {nan, nan}, {nan, nan}, {nan, nan}, {nan, nan}, {nan, nan}, {nan, nan}, {nan, nan}, {nan, nan}, {nan, nan}, {nan, nan}, {nan, nan}, {nan, nan}, {nan, nan}, {nan, nan}, {nan, nan}, {nan, nan}, {nan, nan}, {nan, nan}, {nan, nan}, {nan, nan}, {nan, nan}, {nan, nan}, {nan, nan}, {nan, nan}, {nan, nan}, {nan, nan}, {nan, nan}, {nan, nan}, {nan, nan}, {nan, nan}, {nan, nan}, {nan, nan}, {nan, nan}, {nan, nan}, {nan, nan}, {nan, nan}, {nan, nan}, {nan, nan}, {nan, nan}, {nan, nan}, {nan, nan}, {nan, nan}, {nan, nan}, {nan, nan}, {nan, nan}, {nan, nan}, {nan, nan}, {nan, nan}, {nan, nan}, {nan, nan}, {nan, nan}, {nan, nan}, {nan, nan}, {nan, nan}, {nan, nan}, {nan, nan}, {nan, nan}, {nan, nan}, {nan, nan}, {nan, nan}, {nan, nan}, {nan, nan}, {nan, nan}, {nan, nan}, {nan, nan}, {nan, nan}, {nan, nan}, {nan, nan}, {nan, nan}, {nan, nan}, {nan, nan}, {nan, nan}, {nan, nan}, {nan, nan}, {nan, nan}, {nan, nan}, {nan, nan}, {nan, nan}, {nan, nan}, {nan, nan}, {nan, nan}, {nan, nan}, {nan, nan}, {nan, nan}, {nan, nan}, {nan, nan}, {nan, nan}, {nan, nan}, {nan, nan}, {nan, nan}, {nan, nan}, {nan, nan}, {nan, nan}, {nan, nan}, {nan, nan}, {nan, nan}, {nan, nan}, {nan, nan}, {nan, nan}, {nan, nan}, {nan, nan}, {nan, nan}, {nan, nan}, {nan, nan}, {nan, nan}, {nan, nan}, {nan, nan}, {nan, nan}, {nan, nan}, {nan, nan}, {nan, nan}, {nan, nan}, {nan, nan}, {nan, nan}, {nan, nan}, {nan, nan}, {nan, nan}, {nan, nan}, {nan, nan}, {nan, nan}, {nan, nan}, {nan, nan}, {nan, nan}, {nan, nan}, {nan, nan}, {nan, nan}, {nan, nan}, {nan, nan}, {nan, nan}, {nan, nan}, {nan, nan}, {nan, nan}, {nan, nan}, {nan, nan}, {nan, nan}, {nan, nan}, {nan, nan}, {nan, nan}, {nan, nan}, {nan, nan}, {nan, nan}, {nan, nan}, {nan, nan}, {nan, nan}, {nan, nan}, {nan, nan}, {nan, nan}, {nan, nan}, {nan, nan}, {nan, nan}, {nan, nan}, {nan, nan}, {nan, nan}, {nan, nan}, {nan, nan}, {nan, nan}, {nan, nan}, {nan, nan}, {nan, nan}, {nan, nan}, {nan, nan}, {nan, nan}, {nan, nan}, {nan, nan}, {nan, nan}, {nan, nan}, {nan, nan}, {nan, nan}, {nan, nan}, {nan, nan}, {nan, nan}, {nan, nan}, {nan, nan}, {nan, nan}, {nan, nan}, {nan, nan}, {nan, nan}, {nan, nan}, {nan, nan}, {nan, nan}, {nan, nan}, {nan, nan}, {nan, nan}, {nan, nan}, {nan, nan}, {nan, nan}, {nan, nan}, {nan, nan}, {nan, nan}, {nan, nan}, {nan, nan}, {nan, nan}, {nan, nan}, {nan, nan}, {nan, nan}, {nan, nan}]
  out "OffsetFilePath":string="C:\\Data\\091813\\091813N08.ofs"
  in  "InitialConst":dbl[](array[numeric])
  in  "Stop Voltage (V)":dbl=4.0
  out "OM Vert MTA Voltage":dbl=0.0042724609375 format="%#.3f"
  out "OM Horiz MTA Voltage":dbl format="%#.3f"
  in  "HorizMirrCalib(nm/V)":dbl=752.0
  in  "HorizMirrOffs(V)":dbl
  in  "ClearChart":bool
  in  "Step (V)":dbl=0.01
  in  "#PtsToWait":i32=100
  in  "VertMirrOffs(V)":dbl
  in  "VertMirrCalib(nm/V)":dbl=752.0
  out "IsOffsetModeActive?":bool caption="stop"
  in  "StopOffset":bool caption="stop"
  out "ProgressBar":i32(slide)=200 min=0 max=512 step=1 scale=0.0..200.0
  in  "WindowSample#":i32=2048
  out "HiFreqDiagnostic":T16(graph)={"[0]"=0.002342537045478821, "[1]"=0.0025282055139541626, "[2]"=0.0019662082195281982, "[3]"=0.0019291043281555176, "[4]"=0.005142837762832642, "[5]"=0.0045330822467803955, "[6]"=0.0008034706115722656, "[7]"=0.0034596025943756104}
  in  "HiFSamplingRate/Ch":dbl=25000.0
  out "File Name and Path":string="C:\\Data\\091813\\091813N01.brw"
  in  "Total#OfWindows":dbl=200.0
  out "IsForceExtActive?":bool=TRUE
  in  "FEX Axis":bool=TRUE
  out "ForceExtensionFilePath":string="C:\\Data\\091813\\091813N00.pul"
  in  "StopForceExtension":bool caption="stop"
  in  "#FEXPtsToWait":i32=500
  in  "Mirror Step (V)":dbl=0.0020000000949949026
  out "FEX Force TrapA":cluster{dbl, dbl}[](graph)=[{nan, nan}, {nan, nan}, {nan, nan}, {nan, nan}, {nan, nan}, {nan, nan}, {nan, nan}, {nan, nan}, {nan, nan}, {nan, nan}, {nan, nan}, {nan, nan}, {nan, nan}, {nan, nan}, {nan, nan}, {nan, nan}, {nan, nan}, {nan, nan}, {nan, nan}, {nan, nan}, {nan, nan}, {nan, nan}, {nan, nan}, {nan, nan}, {nan, nan}, {nan, nan}, {nan, nan}, {nan, nan}, {nan, nan}, {nan, nan}, {nan, nan}, {nan, nan}, {nan, nan}, {nan, nan}, {nan, nan}, {nan, nan}, {nan, nan}, {nan, nan}, {nan, nan}, {nan, nan}, {nan, nan}, {nan, nan}, {nan, nan}, {nan, nan}, {nan, nan}, {nan, nan}, {nan, nan}, {nan, nan}, {nan, nan}, {nan, nan}, {nan, nan}, {nan, nan}, {nan, nan}, {nan, nan}, {nan, nan}, {nan, nan}, {nan, nan}, {nan, nan}, {nan, nan}, {nan, nan}, {nan, nan}, {nan, nan}, {nan, nan}, {nan, nan}, {nan, nan}, {nan, nan}, {nan, nan}, {nan, nan}, {nan, nan}, {nan, nan}, {nan, nan}, {nan, nan}, {nan, nan}, {nan, nan}, {nan, nan}, {nan, nan}, {nan, nan}, {nan, nan}, {nan, nan}, {nan, nan}, {nan, nan}, {nan, nan}, {nan, nan}, {nan, nan}, {nan, nan}, {nan, nan}, {nan, nan}, {nan, nan}, {nan, nan}, {nan, nan}, {nan, nan}, {nan, nan}, {nan, nan}, {nan, nan}, {nan, nan}, {nan, nan}, {nan, nan}, {nan, nan}, {nan, nan}, {nan, nan}, {nan, nan}, {nan, nan}, {nan, nan}, {nan, nan}, {nan, nan}, {nan, nan}, {nan, nan}, {nan, nan}, {nan, nan}, {nan, nan}, {nan, nan}, {nan, nan}, {nan, nan}, {nan, nan}, {nan, nan}, {nan, nan}, {nan, nan}, {nan, nan}, {nan, nan}, {nan, nan}, {nan, nan}, {nan, nan}, {nan, nan}, {nan, nan}, {nan, nan}, {nan, nan}, {nan, nan}, {nan, nan}, {nan, nan}, {nan, nan}, {nan, nan}, {nan, nan}, {nan, nan}, {nan, nan}, {nan, nan}, {nan, nan}, {nan, nan}, {nan, nan}, {nan, nan}, {nan, nan}, {nan, nan}, {nan, nan}, {nan, nan}, {nan, nan}, {nan, nan}, {nan, nan}, {nan, nan}, {nan, nan}, {nan, nan}, {nan, nan}, {nan, nan}, {nan, nan}, {nan, nan}, {nan, nan}, {nan, nan}, {nan, nan}, {nan, nan}, {nan, nan}, {nan, nan}, {nan, nan}, {nan, nan}, {nan, nan}, {nan, nan}, {nan, nan}, {nan, nan}, {nan, nan}, {nan, nan}, {nan, nan}, {nan, nan}, {nan, nan}, {nan, nan}, {nan, nan}, {nan, nan}, {nan, nan}, {nan, nan}, {nan, nan}, {nan, nan}, {nan, nan}, {nan, nan}, {nan, nan}, {nan, nan}, {nan, nan}, {nan, nan}, {nan, nan}, {nan, nan}, {nan, nan}, {nan, nan}, {nan, nan}, {nan, nan}, {nan, nan}, {nan, nan}, {nan, nan}, {nan, nan}, {nan, nan}, {nan, nan}, {nan, nan}, {nan, nan}, {nan, nan}, {nan, nan}, {nan, nan}, {nan, nan}, {nan, nan}, {nan, nan}, {nan, nan}, {nan, nan}, {nan, nan}, {nan, nan}, {nan, nan}, {nan, nan}, {nan, nan}, {nan, nan}, {nan, nan}, {nan, nan}, {nan, nan}, {nan, nan}, {nan, nan}, {nan, nan}, {nan, nan}, {nan, nan}, {nan, nan}, {nan, nan}, {nan, nan}, {nan, nan}, {nan, nan}, {nan, nan}, {nan, nan}, {nan, nan}, {nan, nan}, {nan, nan}, {nan, nan}, {nan, nan}, {nan, nan}, {nan, nan}, {nan, nan}, {nan, nan}, {nan, nan}, {nan, nan}, {nan, nan}, {nan, nan}, {nan, nan}, {nan, nan}, {nan, nan}, {nan, nan}, {nan, nan}, {nan, nan}, {nan, nan}, {nan, nan}, {nan, nan}, {nan, nan}, {nan, nan}, {nan, nan}, {nan, nan}, {nan, nan}, {nan, nan}, {nan, nan}, {nan, nan}, {nan, nan}, {nan, nan}, {nan, nan}, {nan, nan}, {nan, nan}, {nan, nan}, {nan, nan}, {nan, nan}, {nan, nan}, {nan, nan}, {nan, nan}, {nan, nan}, {nan, nan}, {nan, nan}, {nan, nan}, {nan, nan}, {nan, nan}, {nan, nan}, {nan, nan}, {nan, nan}, {nan, nan}, {nan, nan}, {nan, nan}, {nan, nan}, {nan, nan}, {nan, nan}, {nan, nan}, {nan, nan}, {nan, nan}, {nan, nan}, {nan, nan}, {nan, nan}, {nan, nan}, {nan, nan}, {nan, nan}, {nan, nan}, {nan, nan}, {nan, nan}, {nan, nan}, {nan, nan}, {nan, nan}, {nan, nan}, {nan, nan}, {nan, nan}, {nan, nan}, {nan, nan}, {nan, nan}, {nan, nan}, {nan, nan}, {nan, nan}, {nan, nan}, {nan, nan}, {nan, nan}, {nan, nan}, {nan, nan}, {nan, nan}, {nan, nan}, {nan, nan}, {nan, nan}, {nan, nan}, {nan, nan}, {nan, nan}, {nan, nan}, {nan, nan}, {nan, nan}, {nan, nan}, {nan, nan}, {nan, nan}, {nan, nan}, {nan, nan}, {nan, nan}, {nan, nan}, {nan, nan}, {nan, nan}, {nan, nan}, {nan, nan}, {nan, nan}, {nan, nan}, {nan, nan}, {nan, nan}, {nan, nan}, {nan, nan}, {nan, nan}, {nan, nan}, {nan, nan}, {nan, nan}, {nan, nan}, {nan, nan}, {nan, nan}, {nan, nan}, {nan, nan}, {nan, nan}, {nan, nan}, {nan, nan}, {nan, nan}, {nan, nan}, {nan, nan}, {nan, nan}, {nan, nan}, {nan, nan}, {nan, nan}, {nan, nan}, {nan, nan}, {nan, nan}, {nan, nan}, {nan, nan}, {nan, nan}, {nan, nan}, {nan, nan}, {nan, nan}, {nan, nan}, {nan, nan}, {nan, nan}, {nan, nan}, {nan, nan}, {nan, nan}, {nan, nan}, {nan, nan}, {nan, nan}, {nan, nan}, {nan, nan}, {nan, nan}, {nan, nan}, {nan, nan}, {nan, nan}, {nan, nan}, {nan, nan}, {nan, nan}, {nan, nan}, {nan, nan}, {nan, nan}, {nan, nan}, {nan, nan}, {nan, nan}, {nan, nan}, {nan, nan}, {nan, nan}, {nan, nan}, {nan, nan}, {nan, nan}, {nan, nan}, {nan, nan}, {nan, nan}, {nan, nan}, {nan, nan}, {nan, nan}, {nan, nan}, {nan, nan}, {nan, nan}, {nan, nan}, {nan, nan}, {nan, nan}, {nan, nan}, {nan, nan}, {nan, nan}, {nan, nan}, {nan, nan}, {nan, nan}, {nan, nan}, {nan, nan}, {nan, nan}, {nan, nan}, {nan, nan}, {nan, nan}, {nan, nan}, {nan, nan}, {nan, nan}, {nan, nan}, {nan, nan}, {nan, nan}, {nan, nan}, {nan, nan}, {nan, nan}, {nan, nan}, {nan, nan}, {nan, nan}, {nan, nan}, {nan, nan}, {nan, nan}, {nan, nan}, {nan, nan}, {nan, nan}, {nan, nan}, {nan, nan}, {nan, nan}, {nan, nan}, {nan, nan}, {nan, nan}, {nan, nan}, {nan, nan}, {nan, nan}, {nan, nan}, {nan, nan}, {nan, nan}, {nan, nan}, {nan, nan}, {nan, nan}, {nan, nan}, {nan, nan}, {nan, nan}, {nan, nan}, {nan, nan}, {nan, nan}, {nan, nan}, {nan, nan}, {nan, nan}, {nan, nan}, {nan, nan}, {nan, nan}, {nan, nan}, {nan, nan}, {nan, nan}, {nan, nan}, {nan, nan}, {nan, nan}, {nan, nan}, {nan, nan}, {nan, nan}, {nan, nan}, {nan, nan}, {nan, nan}, {nan, nan}, {nan, nan}, {nan, nan}, {nan, nan}, {nan, nan}, {nan, nan}, {nan, nan}, {nan, nan}, {nan, nan}, {nan, nan}, {nan, nan}, {nan, nan}, {nan, nan}, {nan, nan}, {nan, nan}, {nan, nan}, {nan, nan}, {nan, nan}, {nan, nan}, {nan, nan}, {nan, nan}, {nan, nan}, {nan, nan}, {nan, nan}, {nan, nan}, {nan, nan}, {nan, nan}, {nan, nan}, {nan, nan}, {nan, nan}, {nan, nan}, {nan, nan}, {nan, nan}, {nan, nan}, {nan, nan}, {nan, nan}, {nan, nan}, {nan, nan}, {nan, nan}, {nan, nan}, {nan, nan}, {nan, nan}, {nan, nan}, {nan, nan}, {nan, nan}, {nan, nan}, {nan, nan}, {nan, nan}, {nan, nan}, {nan, nan}, {nan, nan}, {nan, nan}, {nan, nan}, {nan, nan}, {nan, nan}, {nan, nan}, {nan, nan}, {nan, nan}, {nan, nan}, {nan, nan}, {nan, nan}, {nan, nan}, {nan, nan}, {nan, nan}, {nan, nan}, {nan, nan}, {nan, nan}, {nan, nan}, {nan, nan}, {nan, nan}, {nan, nan}, {nan, nan}, {nan, nan}, {nan, nan}, {nan, nan}, {nan, nan}, {nan, nan}, {nan, nan}, {nan, nan}, {nan, nan}, {nan, nan}, {nan, nan}, {nan, nan}, {nan, nan}, {nan, nan}, {nan, nan}, {nan, nan}, {nan, nan}, {nan, nan}, {nan, nan}, {nan, nan}, {nan, nan}, {nan, nan}, {nan, nan}, {nan, nan}, {nan, nan}, {nan, nan}, {nan, nan}, {nan, nan}, {nan, nan}, {nan, nan}, {nan, nan}, {nan, nan}, {nan, nan}, {nan, nan}, {nan, nan}, {nan, nan}, {nan, nan}, {nan, nan}, {nan, nan}, {nan, nan}, {nan, nan}, {nan, nan}, {nan, nan}, {nan, nan}, {nan, nan}, {nan, nan}, {nan, nan}, {nan, nan}, {nan, nan}, {nan, nan}, {nan, nan}, {nan, nan}, {nan, nan}, {nan, nan}, {nan, nan}, {nan, nan}, {nan, nan}, {nan, nan}, {nan, nan}, {nan, nan}, {nan, nan}, {nan, nan}, {nan, nan}, {nan, nan}, {nan, nan}, {nan, nan}, {nan, nan}, {nan, nan}, {nan, nan}, {nan, nan}, {nan, nan}, {nan, nan}, {nan, nan}, {nan, nan}, {nan, nan}, {nan, nan}, {nan, nan}, {nan, nan}, {nan, nan}, {nan, nan}, {nan, nan}, {nan, nan}, {nan, nan}, {nan, nan}, {nan, nan}, {nan, nan}, {nan, nan}, {nan, nan}, {nan, nan}, {nan, nan}, {nan, nan}, {nan, nan}, {nan, nan}, {nan, nan}, {nan, nan}, {nan, nan}, {nan, nan}, {nan, nan}, {nan, nan}, {nan, nan}, {nan, nan}, {nan, nan}, {nan, nan}, {nan, nan}, {nan, nan}, {nan, nan}, {nan, nan}, {nan, nan}, {nan, nan}, {nan, nan}, {nan, nan}, {nan, nan}, {nan, nan}, {nan, nan}, {nan, nan}, {nan, nan}, {nan, nan}, {nan, nan}, {nan, nan}, {nan, nan}, {nan, nan}, {nan, nan}, {nan, nan}, {nan, nan}, {nan, nan}, {nan, nan}, {nan, nan}, {nan, nan}, {nan, nan}, {nan, nan}, {nan, nan}, {nan, nan}, {nan, nan}, {nan, nan}, {nan, nan}, {nan, nan}, {nan, nan}, {nan, nan}, {nan, nan}, {nan, nan}, {nan, nan}, {nan, nan}, {nan, nan}, {nan, nan}, {nan, nan}, {nan, nan}, {nan, nan}, {nan, nan}, {nan, nan}, {nan, nan}, {nan, nan}, {nan, nan}, {nan, nan}, {nan, nan}, {nan, nan}, {nan, nan}, {nan, nan}, {nan, nan}, {nan, nan}, {nan, nan}, {nan, nan}, {nan, nan}, {nan, nan}, {nan, nan}, {nan, nan}, {nan, nan}, {nan, nan}, {nan, nan}, {nan, nan}, {nan, nan}, {nan, nan}, {nan, nan}, {nan, nan}, {nan, nan}, {nan, nan}, {nan, nan}, {nan, nan}, {nan, nan}, {nan, nan}, {nan, nan}, {nan, nan}, {nan, nan}, {nan, nan}, {nan, nan}, {nan, nan}, {nan, nan}, {nan, nan}, {nan, nan}, {nan, nan}, {nan, nan}, {nan, nan}, {nan, nan}, {nan, nan}, {nan, nan}, {nan, nan}, {nan, nan}, {nan, nan}, {nan, nan}, {nan, nan}, {nan, nan}, {nan, nan}, {nan, nan}, {nan, nan}, {nan, nan}, {nan, nan}, {nan, nan}, {nan, nan}, {nan, nan}, {nan, nan}, {nan, nan}, {nan, nan}, {nan, nan}, {nan, nan}, {nan, nan}, {nan, nan}, {nan, nan}, {nan, nan}, {nan, nan}, {nan, nan}, {nan, nan}, {nan, nan}, {nan, nan}, {nan, nan}, {nan, nan}, {nan, nan}, {nan, nan}, {nan, nan}, {nan, nan}, {nan, nan}, {nan, nan}, {nan, nan}, {nan, nan}, {nan, nan}, {nan, nan}, {nan, nan}, {nan, nan}, {nan, nan}, {nan, nan}, {nan, nan}, {nan, nan}, {nan, nan}, {nan, nan}, {nan, nan}, {nan, nan}, {nan, nan}, {nan, nan}, {nan, nan}, {nan, nan}, {nan, nan}, {nan, nan}, {nan, nan}, {nan, nan}, {nan, nan}, {nan, nan}, {nan, nan}, {nan, nan}, {nan, nan}, {nan, nan}, {nan, nan}, {nan, nan}, {nan, nan}, {nan, nan}, {nan, nan}, {nan, nan}, {nan, nan}, {nan, nan}, {nan, nan}, {nan, nan}, {nan, nan}, {nan, nan}, {nan, nan}, {nan, nan}, {nan, nan}, {nan, nan}, {nan, nan}, {nan, nan}, {nan, nan}, {nan, nan}, {nan, nan}, {nan, nan}, {nan, nan}, {nan, nan}, {nan, nan}, {nan, nan}, {nan, nan}, {nan, nan}, {nan, nan}, {nan, nan}, {nan, nan}, {nan, nan}, {nan, nan}, {nan, nan}, {nan, nan}, {nan, nan}, {nan, nan}, {nan, nan}, {nan, nan}, {nan, nan}, {nan, nan}, {nan, nan}, {nan, nan}, {nan, nan}, {nan, nan}, {nan, nan}, {nan, nan}, {nan, nan}, {nan, nan}, {nan, nan}, {nan, nan}, {nan, nan}, {nan, nan}, {nan, nan}, {nan, nan}, {nan, nan}, {nan, nan}, {nan, nan}, {nan, nan}, {nan, nan}, {nan, nan}, {nan, nan}, {nan, nan}, {nan, nan}, {nan, nan}, {nan, nan}, {nan, nan}, {nan, nan}, {nan, nan}, {nan, nan}, {nan, nan}, {nan, nan}, {nan, nan}, {nan, nan}, {nan, nan}, {nan, nan}, {nan, nan}, {nan, nan}, {nan, nan}, {nan, nan}, {nan, nan}, {nan, nan}, {nan, nan}, {nan, nan}, {nan, nan}, {nan, nan}, {nan, nan}, {nan, nan}, {nan, nan}, {nan, nan}, {nan, nan}, {nan, nan}, {nan, nan}, {nan, nan}, {nan, nan}, {nan, nan}, {nan, nan}, {nan, nan}, {nan, nan}, {nan, nan}, {nan, nan}, {nan, nan}, {nan, nan}, {nan, nan}, {nan, nan}, {nan, nan}, {nan, nan}, {nan, nan}, {nan, nan}, {nan, nan}, {nan, nan}, {nan, nan}, {nan, nan}, {nan, nan}, {nan, nan}, {nan, nan}, {nan, nan}, {nan, nan}, {nan, nan}, {nan, nan}, {nan, nan}, {nan, nan}, {nan, nan}, {nan, nan}, {nan, nan}, {nan, nan}, {nan, nan}, {nan, nan}, {nan, nan}, {nan, nan}, {nan, nan}, {nan, nan}, {nan, nan}, {nan, nan}, {nan, nan}, {nan, nan}, {nan, nan}, {nan, nan}, {nan, nan}, {nan, nan}, {nan, nan}, {nan, nan}, {nan, nan}, {nan, nan}, {nan, nan}, {nan, nan}, {nan, nan}, {nan, nan}, {nan, nan}, {nan, nan}, {nan, nan}, {nan, nan}, {nan, nan}, {7.638962495303106, 2.456849346640493}, {7.84670121492986, 2.456180715056149}, {7.942545246743487, 2.427469325692295}, {7.900969908567134, 2.4098354947322864}, {7.865465305611222, 2.4495638510702538}, {7.966782197206914, 2.4496951071687545}, {7.87006434744489, 2.4490746455516}, {7.8437578281563125, 2.45506709388253}, {7.911915628131262, 2.4425679963649523}, {7.901751745678857, 2.4404390355076924}, {7.878296632327154, 2.4306340867881993}, {7.863901631387775, 2.4648225046672785}, {7.918262305861724, 2.4575404686155946}, {7.864867430172846, 2.463818476380022}, {7.959331749436373, 2.4372888251352878}, {7.861234187124248, 2.4390292519711547}, {7.891403901553106, 2.4337530028631815}, {7.908466346756012, 2.451178545183674}, {7.8473910712049095, 2.430505249229798}, {7.884597319639279, 2.417524377874045}, {7.856543164453908, 2.4550126445337797}, {7.876594986848698, 2.4463404091548315}, {7.878250641908818, 2.4296030107026403}, {7.936796444451403, 2.4391183372916156}, {7.883263597507515, 2.4300972184127314}, {7.9049710749624245, 2.454844207830699}, {7.840538498872745, 2.4269627273809995}, {7.8741574946768536, 2.455451506050127}, {7.862935832602705, 2.442907047277978}, {7.929116044589178, 2.4194841577810426}, {7.815749663389279, 2.3985679248140253}, {7.880228229897295, 2.447961704588897}, {7.8477589945516035, 2.4208019123274913}, {7.914491091558117, 2.4398445687182324}, {7.89535907753006, 2.4237016421698336}, {7.933945038514529, 2.451442492194818}, {7.8621080050726455, 2.464890983956254}, {7.848310879571644, 2.4305929769253565}, {7.891541872808117, 2.4451493905929733}, {7.843803818574649, 2.440983690848668}, {7.833777907377255, 2.432451028667969}]
  out "FEX Noise-Ext":cluster{dbl, dbl}[](graph)=[{nan, -0.0}, {nan, -0.0}, {nan, -0.0}, {nan, -0.0}, {nan, -0.0}, {nan, -0.0}, {nan, -0.0}, {nan, -0.0}, {nan, -0.0}, {nan, -0.0}, {nan, -0.0}, {nan, -0.0}, {nan, -0.0}, {nan, -0.0}, {nan, -0.0}, {nan, -0.0}, {nan, -0.0}, {nan, -0.0}, {nan, -0.0}, {nan, -0.0}, {nan, -0.0}, {nan, -0.0}, {nan, -0.0}, {nan, -0.0}, {nan, -0.0}, {nan, -0.0}, {nan, -0.0}, {nan, -0.0}, {nan, -0.0}, {nan, -0.0}, {nan, -0.0}, {nan, -0.0}, {nan, -0.0}, {nan, -0.0}, {nan, -0.0}, {nan, -0.0}, {nan, -0.0}, {nan, -0.0}, {nan, -0.0}, {nan, -0.0}, {nan, -0.0}, {nan, -0.0}, {nan, -0.0}, {nan, -0.0}, {nan, -0.0}, {nan, -0.0}, {nan, -0.0}, {nan, -0.0}, {nan, -0.0}, {nan, -0.0}, {nan, -0.0}, {nan, -0.0}, {nan, -0.0}, {nan, -0.0}, {nan, -0.0}, {nan, -0.0}, {nan, -0.0}, {nan, -0.0}, {nan, -0.0}, {nan, -0.0}, {nan, -0.0}, {nan, -0.0}, {nan, -0.0}, {nan, -0.0}, {nan, -0.0}, {nan, -0.0}, {nan, -0.0}, {nan, -0.0}, {nan, -0.0}, {nan, -0.0}, {nan, -0.0}, {nan, -0.0}, {nan, -0.0}, {nan, -0.0}, {nan, -0.0}, {nan, -0.0}, {nan, -0.0}, {nan, -0.0}, {nan, -0.0}, {nan, -0.0}, {nan, -0.0}, {nan, -0.0}, {nan, -0.0}, {nan, -0.0}, {nan, -0.0}, {nan, -0.0}, {nan, -0.0}, {nan, -0.0}, {nan, -0.0}, {nan, -0.0}, {nan, -0.0}, {nan, -0.0}, {nan, -0.0}, {nan, -0.0}, {nan, -0.0}, {nan, -0.0}, {nan, -0.0}, {nan, -0.0}, {nan, -0.0}, {nan, -0.0}, {nan, -0.0}, {nan, -0.0}, {nan, -0.0}, {nan, -0.0}, {nan, -0.0}, {nan, -0.0}, {nan, -0.0}, {nan, -0.0}, {nan, -0.0}, {nan, -0.0}, {nan, -0.0}, {nan, -0.0}, {nan, -0.0}, {nan, -0.0}, {nan, -0.0}, {nan, -0.0}, {nan, -0.0}, {nan, -0.0}, {nan, -0.0}, {nan, -0.0}, {nan, -0.0}, {nan, -0.0}, {nan, -0.0}, {nan, -0.0}, {nan, -0.0}, {nan, -0.0}, {nan, -0.0}, {nan, -0.0}, {nan, -0.0}, {nan, -0.0}, {nan, -0.0}, {nan, -0.0}, {nan, -0.0}, {nan, -0.0}, {nan, -0.0}, {nan, -0.0}, {nan, -0.0}, {nan, -0.0}, {nan, -0.0}, {nan, -0.0}, {nan, -0.0}, {nan, -0.0}, {nan, -0.0}, {nan, -0.0}, {nan, -0.0}, {nan, -0.0}, {nan, -0.0}, {nan, -0.0}, {nan, -0.0}, {nan, -0.0}, {nan, -0.0}, {nan, -0.0}, {nan, -0.0}, {nan, -0.0}, {nan, -0.0}, {nan, -0.0}, {nan, -0.0}, {nan, -0.0}, {nan, -0.0}, {nan, -0.0}, {nan, -0.0}, {nan, -0.0}, {nan, -0.0}, {nan, -0.0}, {nan, -0.0}, {nan, -0.0}, {nan, -0.0}, {nan, -0.0}, {nan, -0.0}, {nan, -0.0}, {nan, -0.0}, {nan, -0.0}, {nan, -0.0}, {nan, -0.0}, {nan, -0.0}, {nan, -0.0}, {nan, -0.0}, {nan, -0.0}, {nan, -0.0}, {nan, -0.0}, {nan, -0.0}, {nan, -0.0}, {nan, -0.0}, {nan, -0.0}, {nan, -0.0}, {nan, -0.0}, {nan, -0.0}, {nan, -0.0}, {nan, -0.0}, {nan, -0.0}, {nan, -0.0}, {nan, -0.0}, {nan, -0.0}, {nan, -0.0}, {nan, -0.0}, {nan, -0.0}, {nan, -0.0}, {nan, -0.0}, {nan, -0.0}, {nan, -0.0}, {nan, -0.0}, {nan, -0.0}, {nan, -0.0}, {nan, -0.0}, {nan, -0.0}, {nan, -0.0}, {nan, -0.0}, {nan, -0.0}, {nan, -0.0}, {nan, -0.0}, {nan, -0.0}, {nan, -0.0}, {nan, -0.0}, {nan, -0.0}, {nan, -0.0}, {nan, -0.0}, {nan, -0.0}, {nan, -0.0}, {nan, -0.0}, {nan, -0.0}, {nan, -0.0}, {nan, -0.0}, {nan, -0.0}, {nan, -0.0}, {nan, -0.0}, {nan, -0.0}, {nan, -0.0}, {nan, -0.0}, {nan, -0.0}, {nan, -0.0}, {nan, -0.0}, {nan, -0.0}, {nan, -0.0}, {nan, -0.0}, {nan, -0.0}, {nan, -0.0}, {nan, -0.0}, {nan, -0.0}, {nan, -0.0}, {nan, -0.0}, {nan, -0.0}, {nan, -0.0}, {nan, -0.0}, {nan, -0.0}, {nan, -0.0}, {nan, -0.0}, {nan, -0.0}, {nan, -0.0}, {nan, -0.0}, {nan, -0.0}, {nan, -0.0}, {nan, -0.0}, {nan, -0.0}, {nan, -0.0}, {nan, -0.0}, {nan, -0.0}, {nan, -0.0}, {nan, -0.0}, {nan, -0.0}, {nan, -0.0}, {nan, -0.0}, {nan, -0.0}, {nan, -0.0}, {nan, -0.0}, {nan, -0.0}, {nan, -0.0}, {nan, -0.0}, {nan, -0.0}, {nan, -0.0}, {nan, -0.0}, {nan, -0.0}, {nan, -0.0}, {nan, -0.0}, {nan, -0.0}, {nan, -0.0}, {nan, -0.0}, {nan, -0.0}, {nan, -0.0}, {nan, -0.0}, {nan, -0.0}, {nan, -0.0}, {nan, -0.0}, {nan, -0.0}, {nan, -0.0}, {nan, -0.0}, {nan, -0.0}, {nan, -0.0}, {nan, -0.0}, {nan, -0.0}, {nan, -0.0}, {nan, -0.0}, {nan, -0.0}, {nan, -0.0}, {nan, -0.0}, {nan, -0.0}, {nan, -0.0}, {nan, -0.0}, {nan, -0.0}, {nan, -0.0}, {nan, -0.0}, {nan, -0.0}, {nan, -0.0}, {nan, -0.0}, {nan, -0.0}, {nan, -0.0}, {nan, -0.0}, {nan, -0.0}, {nan, -0.0}, {nan, -0.0}, {nan, -0.0}, {nan, -0.0}, {nan, -0.0}, {nan, -0.0}, {nan, -0.0}, {nan, -0.0}, {nan, -0.0}, {nan, -0.0}, {nan, -0.0}, {nan, -0.0}, {nan, -0.0}, {nan, -0.0}, {nan, -0.0}, {nan, -0.0}, {nan, -0.0}, {nan, -0.0}, {nan, -0.0}, {nan, -0.0}, {nan, -0.0}, {nan, -0.0}, {nan, -0.0}, {nan, -0.0}, {nan, -0.0}, {nan, -0.0}, {nan, -0.0}, {nan, -0.0}, {nan, -0.0}, {nan, -0.0}, {nan, -0.0}, {nan, -0.0}, {nan, -0.0}, {nan, -0.0}, {nan, -0.0}, {nan, -0.0}, {nan, -0.0}, {nan, -0.0}, {nan, -0.0}, {nan, -0.0}, {nan, -0.0}, {nan, -0.0}, {nan, -0.0}, {nan, -0.0}, {nan, -0.0}, {nan, -0.0}, {nan, -0.0}, {nan, -0.0}, {nan, -0.0}, {nan, -0.0}, {nan, -0.0}, {nan, -0.0}, {nan, -0.0}, {nan, -0.0}, {nan, -0.0}, {nan, -0.0}, {nan, -0.0}, {nan, -0.0}, {nan, -0.0}, {nan, -0.0}, {nan, -0.0}, {nan, -0.0}, {nan, -0.0}, {nan, -0.0}, {nan, -0.0}, {nan, -0.0}, {nan, -0.0}, {nan, -0.0}, {nan, -0.0}, {nan, -0.0}, {nan, -0.0}, {nan, -0.0}, {nan, -0.0}, {nan, -0.0}, {nan, -0.0}, {nan, -0.0}, {nan, -0.0}, {nan, -0.0}, {nan, -0.0}, {nan, -0.0}, {nan, -0.0}, {nan, -0.0}, {nan, -0.0}, {nan, -0.0}, {nan, -0.0}, {nan, -0.0}, {nan, -0.0}, {nan, -0.0}, {nan, -0.0}, {nan, -0.0}, {nan, -0.0}, {nan, -0.0}, {nan, -0.0}, {nan, -0.0}, {nan, -0.0}, {nan, -0.0}, {nan, -0.0}, {nan, -0.0}, {nan, -0.0}, {nan, -0.0}, {nan, -0.0}, {nan, -0.0}, {nan, -0.0}, {nan, -0.0}, {nan, -0.0}, {nan, -0.0}, {nan, -0.0}, {nan, -0.0}, {nan, -0.0}, {nan, -0.0}, {nan, -0.0}, {nan, -0.0}, {nan, -0.0}, {nan, -0.0}, {nan, -0.0}, {nan, -0.0}, {nan, -0.0}, {nan, -0.0}, {nan, -0.0}, {nan, -0.0}, {nan, -0.0}, {nan, -0.0}, {nan, -0.0}, {nan, -0.0}, {nan, -0.0}, {nan, -0.0}, {nan, -0.0}, {nan, -0.0}, {nan, -0.0}, {nan, -0.0}, {nan, -0.0}, {nan, -0.0}, {nan, -0.0}, {nan, -0.0}, {nan, -0.0}, {nan, -0.0}, {nan, -0.0}, {nan, -0.0}, {nan, -0.0}, {nan, -0.0}, {nan, -0.0}, {nan, -0.0}, {nan, -0.0}, {nan, -0.0}, {nan, -0.0}, {nan, -0.0}, {nan, -0.0}, {nan, -0.0}, {nan, -0.0}, {nan, -0.0}, {nan, -0.0}, {nan, -0.0}, {nan, -0.0}, {nan, -0.0}, {nan, -0.0}, {nan, -0.0}, {nan, -0.0}, {nan, -0.0}, {nan, -0.0}, {nan, -0.0}, {nan, -0.0}, {nan, -0.0}, {nan, -0.0}, {nan, -0.0}, {nan, -0.0}, {nan, -0.0}, {nan, -0.0}, {nan, -0.0}, {nan, -0.0}, {nan, -0.0}, {nan, -0.0}, {nan, -0.0}, {nan, -0.0}, {nan, -0.0}, {nan, -0.0}, {nan, -0.0}, {nan, -0.0}, {nan, -0.0}, {nan, -0.0}, {nan, -0.0}, {nan, -0.0}, {nan, -0.0}, {nan, -0.0}, {nan, -0.0}, {nan, -0.0}, {nan, -0.0}, {nan, -0.0}, {nan, -0.0}, {nan, -0.0}, {nan, -0.0}, {nan, -0.0}, {nan, -0.0}, {nan, -0.0}, {nan, -0.0}, {nan, -0.0}, {nan, -0.0}, {nan, -0.0}, {nan, -0.0}, {nan, -0.0}, {nan, -0.0}, {nan, -0.0}, {nan, -0.0}, {nan, -0.0}, {nan, -0.0}, {nan, -0.0}, {nan, -0.0}, {nan, -0.0}, {nan, -0.0}, {nan, -0.0}, {nan, -0.0}, {nan, -0.0}, {nan, -0.0}, {nan, -0.0}, {nan, -0.0}, {nan, -0.0}, {nan, -0.0}, {nan, -0.0}, {nan, -0.0}, {nan, -0.0}, {nan, -0.0}, {nan, -0.0}, {nan, -0.0}, {nan, -0.0}, {nan, -0.0}, {nan, -0.0}, {nan, -0.0}, {nan, -0.0}, {nan, -0.0}, {nan, -0.0}, {nan, -0.0}, {nan, -0.0}, {nan, -0.0}, {nan, -0.0}, {nan, -0.0}, {nan, -0.0}, {nan, -0.0}, {nan, -0.0}, {nan, -0.0}, {nan, -0.0}, {nan, -0.0}, {nan, -0.0}, {nan, -0.0}, {nan, -0.0}, {nan, -0.0}, {nan, -0.0}, {nan, -0.0}, {nan, -0.0}, {nan, -0.0}, {nan, -0.0}, {nan, -0.0}, {nan, -0.0}, {nan, -0.0}, {nan, -0.0}, {nan, -0.0}, {nan, -0.0}, {nan, -0.0}, {nan, -0.0}, {nan, -0.0}, {nan, -0.0}, {nan, -0.0}, {nan, -0.0}, {nan, -0.0}, {nan, -0.0}, {nan, -0.0}, {nan, -0.0}, {nan, -0.0}, {nan, -0.0}, {nan, -0.0}, {nan, -0.0}, {nan, -0.0}, {nan, -0.0}, {nan, -0.0}, {nan, -0.0}, {nan, -0.0}, {nan, -0.0}, {nan, -0.0}, {nan, -0.0}, {nan, -0.0}, {nan, -0.0}, {nan, -0.0}, {nan, -0.0}, {nan, -0.0}, {nan, -0.0}, {nan, -0.0}, {nan, -0.0}, {nan, -0.0}, {nan, -0.0}, {nan, -0.0}, {nan, -0.0}, {nan, -0.0}, {nan, -0.0}, {nan, -0.0}, {nan, -0.0}, {nan, -0.0}, {nan, -0.0}, {nan, -0.0}, {nan, -0.0}, {nan, -0.0}, {nan, -0.0}, {nan, -0.0}, {nan, -0.0}, {nan, -0.0}, {nan, -0.0}, {nan, -0.0}, {nan, -0.0}, {nan, -0.0}, {nan, -0.0}, {nan, -0.0}, {nan, -0.0}, {nan, -0.0}, {nan, -0.0}, {nan, -0.0}, {nan, -0.0}, {nan, -0.0}, {nan, -0.0}, {nan, -0.0}, {nan, -0.0}, {nan, -0.0}, {nan, -0.0}, {nan, -0.0}, {nan, -0.0}, {nan, -0.0}, {nan, -0.0}, {nan, -0.0}, {nan, -0.0}, {nan, -0.0}, {nan, -0.0}, {nan, -0.0}, {nan, -0.0}, {nan, -0.0}, {nan, -0.0}, {nan, -0.0}, {nan, -0.0}, {nan, -0.0}, {nan, -0.0}, {nan, -0.0}, {nan, -0.0}, {nan, -0.0}, {nan, -0.0}, {nan, -0.0}, {nan, -0.0}, {nan, -0.0}, {nan, -0.0}, {nan, -0.0}, {nan, -0.0}, {nan, -0.0}, {nan, -0.0}, {nan, -0.0}, {nan, -0.0}, {nan, -0.0}, {nan, -0.0}, {nan, -0.0}, {nan, -0.0}, {nan, -0.0}, {nan, -0.0}, {nan, -0.0}, {nan, -0.0}, {nan, -0.0}, {nan, -0.0}, {nan, -0.0}, {nan, -0.0}, {nan, -0.0}, {nan, -0.0}, {nan, -0.0}, {nan, -0.0}, {nan, -0.0}, {nan, -0.0}, {nan, -0.0}, {nan, -0.0}, {nan, -0.0}, {nan, -0.0}, {nan, -0.0}, {nan, -0.0}, {nan, -0.0}, {nan, -0.0}, {nan, -0.0}, {nan, -0.0}, {nan, -0.0}, {nan, -0.0}, {nan, -0.0}, {nan, -0.0}, {nan, -0.0}, {nan, -0.0}, {nan, -0.0}, {nan, -0.0}, {nan, -0.0}, {nan, -0.0}, {nan, -0.0}, {nan, -0.0}, {nan, -0.0}, {nan, -0.0}, {nan, -0.0}, {nan, -0.0}, {nan, -0.0}, {nan, -0.0}, {nan, -0.0}, {nan, -0.0}, {nan, -0.0}, {nan, -0.0}, {nan, -0.0}, {nan, -0.0}, {nan, -0.0}, {nan, -0.0}, {nan, -0.0}, {nan, -0.0}, {nan, -0.0}, {nan, -0.0}, {nan, -0.0}, {nan, -0.0}, {nan, -0.0}, {nan, -0.0}, {nan, -0.0}, {nan, -0.0}, {nan, -0.0}, {nan, -0.0}, {nan, -0.0}, {nan, -0.0}, {nan, -0.0}, {nan, -0.0}, {nan, -0.0}, {nan, -0.0}, {nan, -0.0}, {nan, -0.0}, {nan, -0.0}, {nan, -0.0}, {nan, -0.0}, {nan, -0.0}, {nan, -0.0}, {nan, -0.0}, {nan, -0.0}, {nan, -0.0}, {nan, -0.0}, {nan, -0.0}, {nan, -0.0}, {nan, -0.0}, {nan, -0.0}, {nan, -0.0}, {nan, -0.0}, {nan, -0.0}, {nan, -0.0}, {nan, -0.0}, {nan, -0.0}, {nan, -0.0}, {nan, -0.0}, {nan, -0.0}, {nan, -0.0}, {nan, -0.0}, {nan, -0.0}, {nan, -0.0}, {nan, -0.0}, {nan, -0.0}, {nan, -0.0}, {nan, -0.0}, {nan, -0.0}, {nan, -0.0}, {nan, -0.0}, {nan, -0.0}, {nan, -0.0}, {nan, -0.0}, {nan, -0.0}, {nan, -0.0}, {nan, -0.0}, {nan, -0.0}, {nan, -0.0}, {nan, -0.0}, {nan, -0.0}, {nan, -0.0}, {nan, -0.0}, {nan, -0.0}, {nan, -0.0}, {nan, -0.0}, {nan, -0.0}, {nan, -0.0}, {nan, -0.0}, {nan, -0.0}, {nan, -0.0}, {nan, -0.0}, {nan, -0.0}, {nan, -0.0}, {nan, -0.0}, {nan, -0.0}, {nan, -0.0}, {nan, -0.0}, {nan, -0.0}, {nan, -0.0}, {nan, -0.0}, {nan, -0.0}, {nan, -0.0}, {nan, -0.0}, {nan, -0.0}, {nan, -0.0}, {nan, -0.0}, {nan, -0.0}, {nan, -0.0}, {nan, -0.0}, {nan, -0.0}, {nan, -0.0}, {nan, -0.0}, {nan, -0.0}, {nan, -0.0}, {nan, -0.0}, {nan, -0.0}, {nan, -0.0}, {nan, -0.0}, {nan, -0.0}, {nan, -0.0}, {nan, -0.0}, {nan, -0.0}, {nan, -0.0}, {nan, -0.0}, {nan, -0.0}, {nan, -0.0}, {nan, -0.0}, {nan, -0.0}, {nan, -0.0}, {nan, -0.0}, {nan, -0.0}, {nan, -0.0}, {nan, -0.0}, {nan, -0.0}, {nan, -0.0}, {nan, -0.0}, {nan, -0.0}, {nan, -0.0}, {nan, -0.0}, {nan, -0.0}, {nan, -0.0}, {nan, -0.0}, {nan, -0.0}, {nan, -0.0}, {nan, -0.0}, {nan, -0.0}, {nan, -0.0}, {nan, -0.0}, {nan, -0.0}, {nan, -0.0}, {nan, -0.0}, {nan, -0.0}, {nan, -0.0}, {nan, -0.0}, {nan, -0.0}, {nan, -0.0}, {nan, -0.0}, {nan, -0.0}, {nan, -0.0}, {nan, -0.0}, {nan, -0.0}, {nan, -0.0}, {nan, -0.0}, {nan, -0.0}, {nan, -0.0}, {nan, -0.0}, {nan, -0.0}, {nan, -0.0}, {nan, -0.0}, {nan, -0.0}, {nan, -0.0}, {nan, -0.0}, {nan, -0.0}, {nan, -0.0}, {nan, -0.0}, {nan, -0.0}, {nan, -0.0}, {nan, -0.0}, {nan, -0.0}, {nan, -0.0}, {nan, -0.0}, {nan, -0.0}, {nan, -0.0}, {nan, -0.0}, {nan, -0.0}, {nan, -0.0}, {nan, -0.0}, {nan, -0.0}, {nan, -0.0}, {nan, -0.0}, {nan, -0.0}, {nan, -0.0}, {nan, -0.0}, {nan, -0.0}, {nan, -0.0}, {nan, -0.0}, {nan, -0.0}, {nan, -0.0}, {nan, -0.0}, {nan, -0.0}, {nan, -0.0}, {nan, -0.0}, {nan, -0.0}, {nan, -0.0}, {nan, -0.0}, {nan, -0.0}, {nan, -0.0}, {nan, -0.0}, {nan, -0.0}, {nan, -0.0}, {nan, -0.0}, {nan, -0.0}, {nan, -0.0}, {nan, -0.0}, {nan, -0.0}, {nan, -0.0}, {nan, -0.0}, {nan, -0.0}, {nan, -0.0}, {nan, -0.0}, {nan, -0.0}, {nan, -0.0}, {nan, -0.0}, {nan, -0.0}, {nan, -0.0}, {nan, -0.0}, {nan, -0.0}, {nan, -0.0}, {nan, -0.0}, {nan, -0.0}, {nan, -0.0}, {nan, -0.0}, {nan, -0.0}, {nan, -0.0}, {nan, -0.0}, {nan, -0.0}, {nan, -0.0}, {nan, -0.0}, {nan, -0.0}, {nan, -0.0}, {nan, -0.0}, {nan, -0.0}, {nan, -0.0}, {nan, -0.0}, {nan, -0.0}, {nan, -0.0}, {nan, -0.0}, {nan, -0.0}, {nan, -0.0}, {nan, -0.0}, {nan, -0.0}, {nan, -0.0}, {nan, -0.0}, {nan, -0.0}, {nan, -0.0}, {nan, -0.0}, {nan, -0.0}, {nan, -0.0}, {nan, -0.0}, {nan, -0.0}, {nan, -0.0}, {nan, -0.0}, {nan, -0.0}, {nan, -0.0}, {nan, -0.0}, {nan, -0.0}, {7.638962495303106, 0.9424895025303812}, {7.84670121492986, 0.5282070367470151}, {7.942545246743487, 0.5159960674800174}, {7.900969908567134, 0.4907154316691091}, {7.865465305611222, 0.5191385043313906}, {7.966782197206914, 0.41829504179999155}, {7.87006434744489, 0.6516490364346552}, {7.8437578281563125, 0.4932356122250669}, {7.911915628131262, 0.4821745456477965}, {7.901751745678857, 0.5423211503831956}, {7.878296632327154, 0.47943346326329545}, {7.863901631387775, 0.5166610797022774}, {7.918262305861724, 0.5282630505733534}, {7.864867430172846, 0.40363490227811527}, {7.959331749436373, 0.49292139427239506}, {7.861234187124248, 0.5240573257959174}, {7.891403901553106, 0.48927152745934555}, {7.908466346756012, 0.5340555987810467}, {7.8473910712049095, 0.643118990608639}, {7.884597319639279, 0.5885190763353795}, {7.856543164453908, 0.5073054712202651}, {7.876594986848698, 0.49943787866942396}, {7.878250641908818, 0.499898938801153}, {7.936796444451403, 0.5498592962935136}, {7.883263597507515, 0.4997781722532626}, {7.9049710749624245, 0.5051966386097685}, {7.840538498872745, 0.4450089009781842}, {7.8741574946768536, 0.5609350386555202}, {7.862935832602705, 0.6307906368989648}, {7.929116044589178, 0.5923612817797143}, {7.815749663389279, 0.565545387522218}, {7.880228229897295, 0.5270993781198449}, {7.8477589945516035, 0.5306976897528386}, {7.914491091558117, 0.6210086014010772}, {7.89535907753006, 0.4445374232285632}, {7.933945038514529, 0.5519236459453175}, {7.8621080050726455, 0.549317095654789}, {7.848310879571644, 0.52564045522024}, {7.891541872808117, 0.5519690324295364}, {7.843803818574649, 0.4284688173038872}, {7.833777907377255, 0.5131353218761074}]
  in  "Direction":bool=TRUE
  in  "IsPullActive?":bool
  in  "Clear FEX Chart":bool
  in  "FEX HorizMirrOffs(V)":dbl
  in  "FEX HorizMirrCalib(nm/V)":dbl=752.0
  out "FEX Mirror Y Volt":dbl=0.00537109375 format="%#.3f"
  out "FEX Mirror X Volt":dbl=0.004638671875 format="%#.3f"
  # "ClpXP Optical Tweezers"
  # "Chamber Locations"
  # "Need a Button Here that would read the \nNormalized Offset and save it"
  # "Off"
  # "On"
  # "Off"
  # "On"
  # "Thorlabs Motor Status"
  # "Passive Mode"
  # "when I switch tabs from the passive mode to basic mode, the recording doesn't stop"
  # "The sliders don't do anything in passive mode, fix it"
  # "Whenever I click on Ackquire Offset, it goes back to the basic operation, then I have to ckick again"
  # "Trap Motion Control"
  # "Steerable Mirror Info"
  # "Zero-Force Offset Mode"
  # "High Frequency Data Acquisition"
  # "Adjust the length of acquisition time"
  # "Force-Extension Mode"
  # "Y"
  # "+"
  # "X"
  # "-"
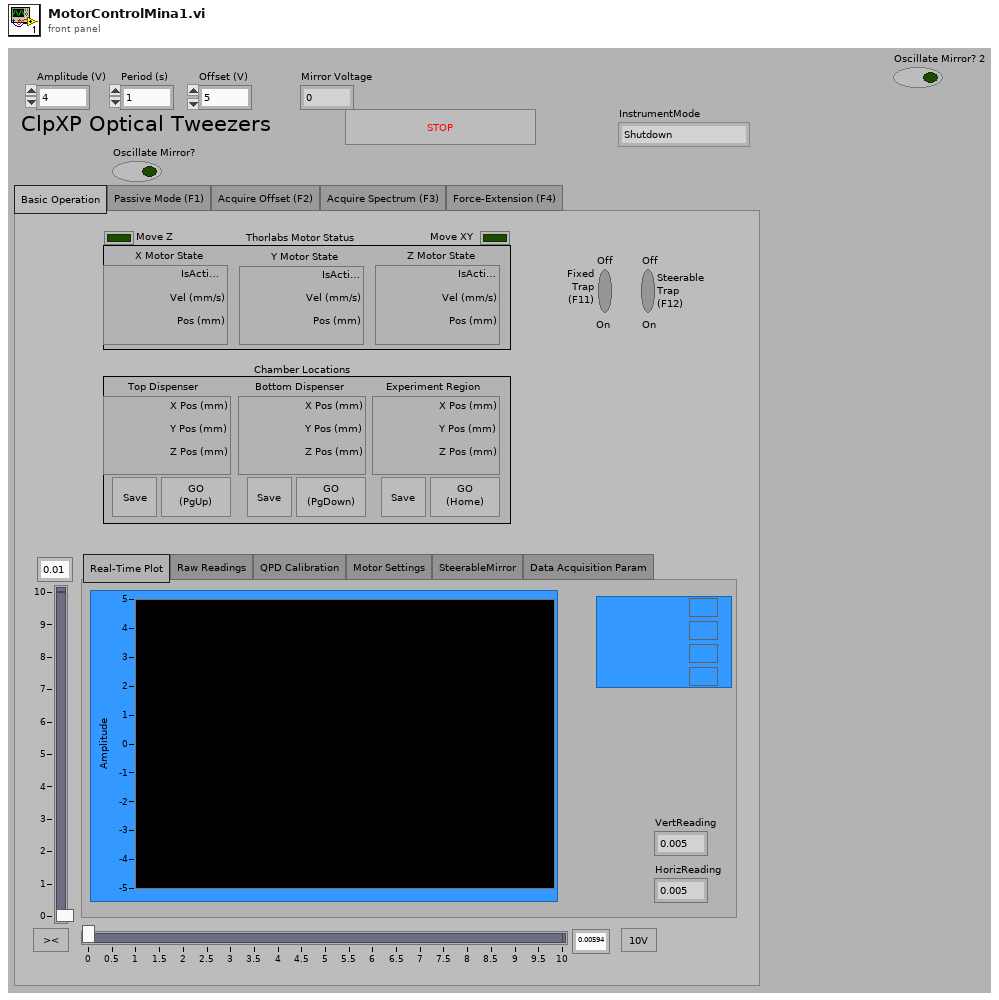
[diagram p1: front panel]
types:
  T1 = enum16{"InitializeJoystick", "InitializeMotors", "BasicMode", "PassiveMode", "AcquireOffsetMode", "AcquireSpectrumMode", "Force-ExtensionMode", "Shutdown"}
  T2 = cluster{"XOffset":i32, "YOffset":i32, "ZOffset":i32}
  T3 = cluster{"XRelPos":i32, "YRelPos":i32, "ZRelPos":i32}
  T4 = enum32{"Basic Operation", "Passive Mode (F1)", "Acquire Offset (F2)", "Acquire Spectrum (F3)", "Force-Extension (F4)"}
  T5 = cluster{"X Pos (mm)":sgl, "Y Pos (mm)":sgl, "Z Pos (mm)":sgl}
  T6 = enum32{"Real-Time Plot", "Raw Readings", "QPD Calibration", "Motor Settings", "SteerableMirror", "Data Acquisition Param"}
  T7 = cluster{"Horizontal Voltage (V)":dbl, "Vertical Voltage (V)":dbl, "Sum Voltage (V)":dbl, "Horizontal Signal (NormV)":dbl, "Vertical Signal (NormV)":dbl}
  T8 = cluster{"Sampling Freq (Hz)":dbl, "#Samples Averaged":i32}
  T9 = cluster{"X Stiff. (pN/nm)":dbl, "X Alpha (nm/NV)":dbl, "X Offset (NV)":dbl, "Y Stiff. (pN/nm)":dbl, "Y Alpha (nm/NV)":dbl, "Y Offset (NV)":dbl}
  T10 = cluster{"Joyst Min Signal":dbl, "Joyst Max Signal":dbl, "Vmax (mm/s)":sgl, "Acc (mm/s/s)":sgl, "+ JoystDirection":i32, "- JoystDirection":i32}
  T11 = cluster{"X Acc (mm/s^2)":sgl, "X Vmax (mm/s)":sgl, "Y Acc (mm/s^2)":sgl, "Y Vmax (mm/s)":sgl, "Z Acc (mm/s^2)":sgl, "Z Vmax (mm/s)":sgl}
  T12 = cluster{"XMin":sgl, "XMax":sgl, "YMin":sgl, "YMax":sgl, "ZMin":sgl, "ZMax":sgl}
  T13 = cluster{"Hor. Scaling (nm/V)":dbl, "Vert. Scaling (nm/V)":dbl, "Hor. Mirr. Offset (V)":dbl, "Vert. Mirr. Offset (V)":dbl}
  T14 = cluster{"Direction":i32, "Vel (mm/s)":sgl, "IsActive?":bool, "Pos (mm)":sgl}
  T15 = cluster{"[0]":sgl, "[1]":sgl, "[2]":sgl, "[3]":sgl, "[4]":sgl, "[5]":sgl, "[6]":sgl, "[7]":sgl}
  T16 = cluster{"[0]":dbl, "[1]":dbl, "[2]":dbl, "[3]":dbl, "[4]":dbl, "[5]":dbl, "[6]":dbl, "[7]":dbl}
  T17 = typedef "DialogType.ctl" = u16
  T18 = cluster{"XMotorRef":refnum<k7>, "YMotorRef":refnum<k7>, "ZMotorRef":refnum<k7>}
  T19 = enum16{"open", "open or create", "create or replace", "create", "open (read only)"}
  T20 = cluster{"[0]":dbl, "[1]":dbl, "[2]":dbl, "[3]":dbl, "[4]":dbl, "[5]":dbl, "[6]":dbl, "[7]":dbl}[]
  T21 = cluster{"AI0: Vy Steer Trap":dbl, "AI1: Vy Fixed Trap":dbl, "AI2: Vx Steer Trap":dbl, "AI3: Vx Fixed Trap":dbl, "AI4: MTA Yaxis":dbl, "AI5: MTA Xaxis":dbl, "AI6: Vsum Steer Trap":dbl, "AI7: Vsum Fixed Trap":dbl}
  T22 = cluster{"Fx Fixed Trap":dbl, "Fy Fixed Trap":dbl, "Fx Steerable Trap":dbl, "Fy Steerable Trap":dbl}
  T23 = cluster{"Fx Fixed Trap":dbl, "Fx Steerable Trap":dbl}
  T24 = cluster{"Steerable \nTrap\n(F12)":refnum<vi>, "Fixed\nTrap\n(F11)":refnum<vi>}
  T25 = cluster{"Motor Reference":refnum<k7>, "Motor Reference":refnum<k7>, "Motor Reference":refnum<k7>}
  T26 = cluster{"X axis":i32, "Y axis":i32, "Z axis":i32, "X axis rotation":i32, "Y axis rotation":i32, "Z axis rotation":i32, "U axis":i32, "V axis":i32}
  T27 = cluster{"button 1":bool, "button 2":bool, "button 3":bool, "button 4":bool, "button 5":bool, "button 6":bool, "button 7":bool, "button 8":bool, "button 9":bool, "button 10":bool, "button 11":bool, "button 12":bool, "button 13":bool, "button 14":bool, "button 15":bool, "button 16":bool, "button 17":bool, "button 18":bool, "button 19":bool, "button 20":bool, "button 21":bool, "button 22":bool, "button 23":bool, "button 24":bool, "button 25":bool, "button 26":bool, "button 27":bool, "button 28":bool, "button 29":bool, "button 30":bool, "button 31":bool, "button 32":bool}
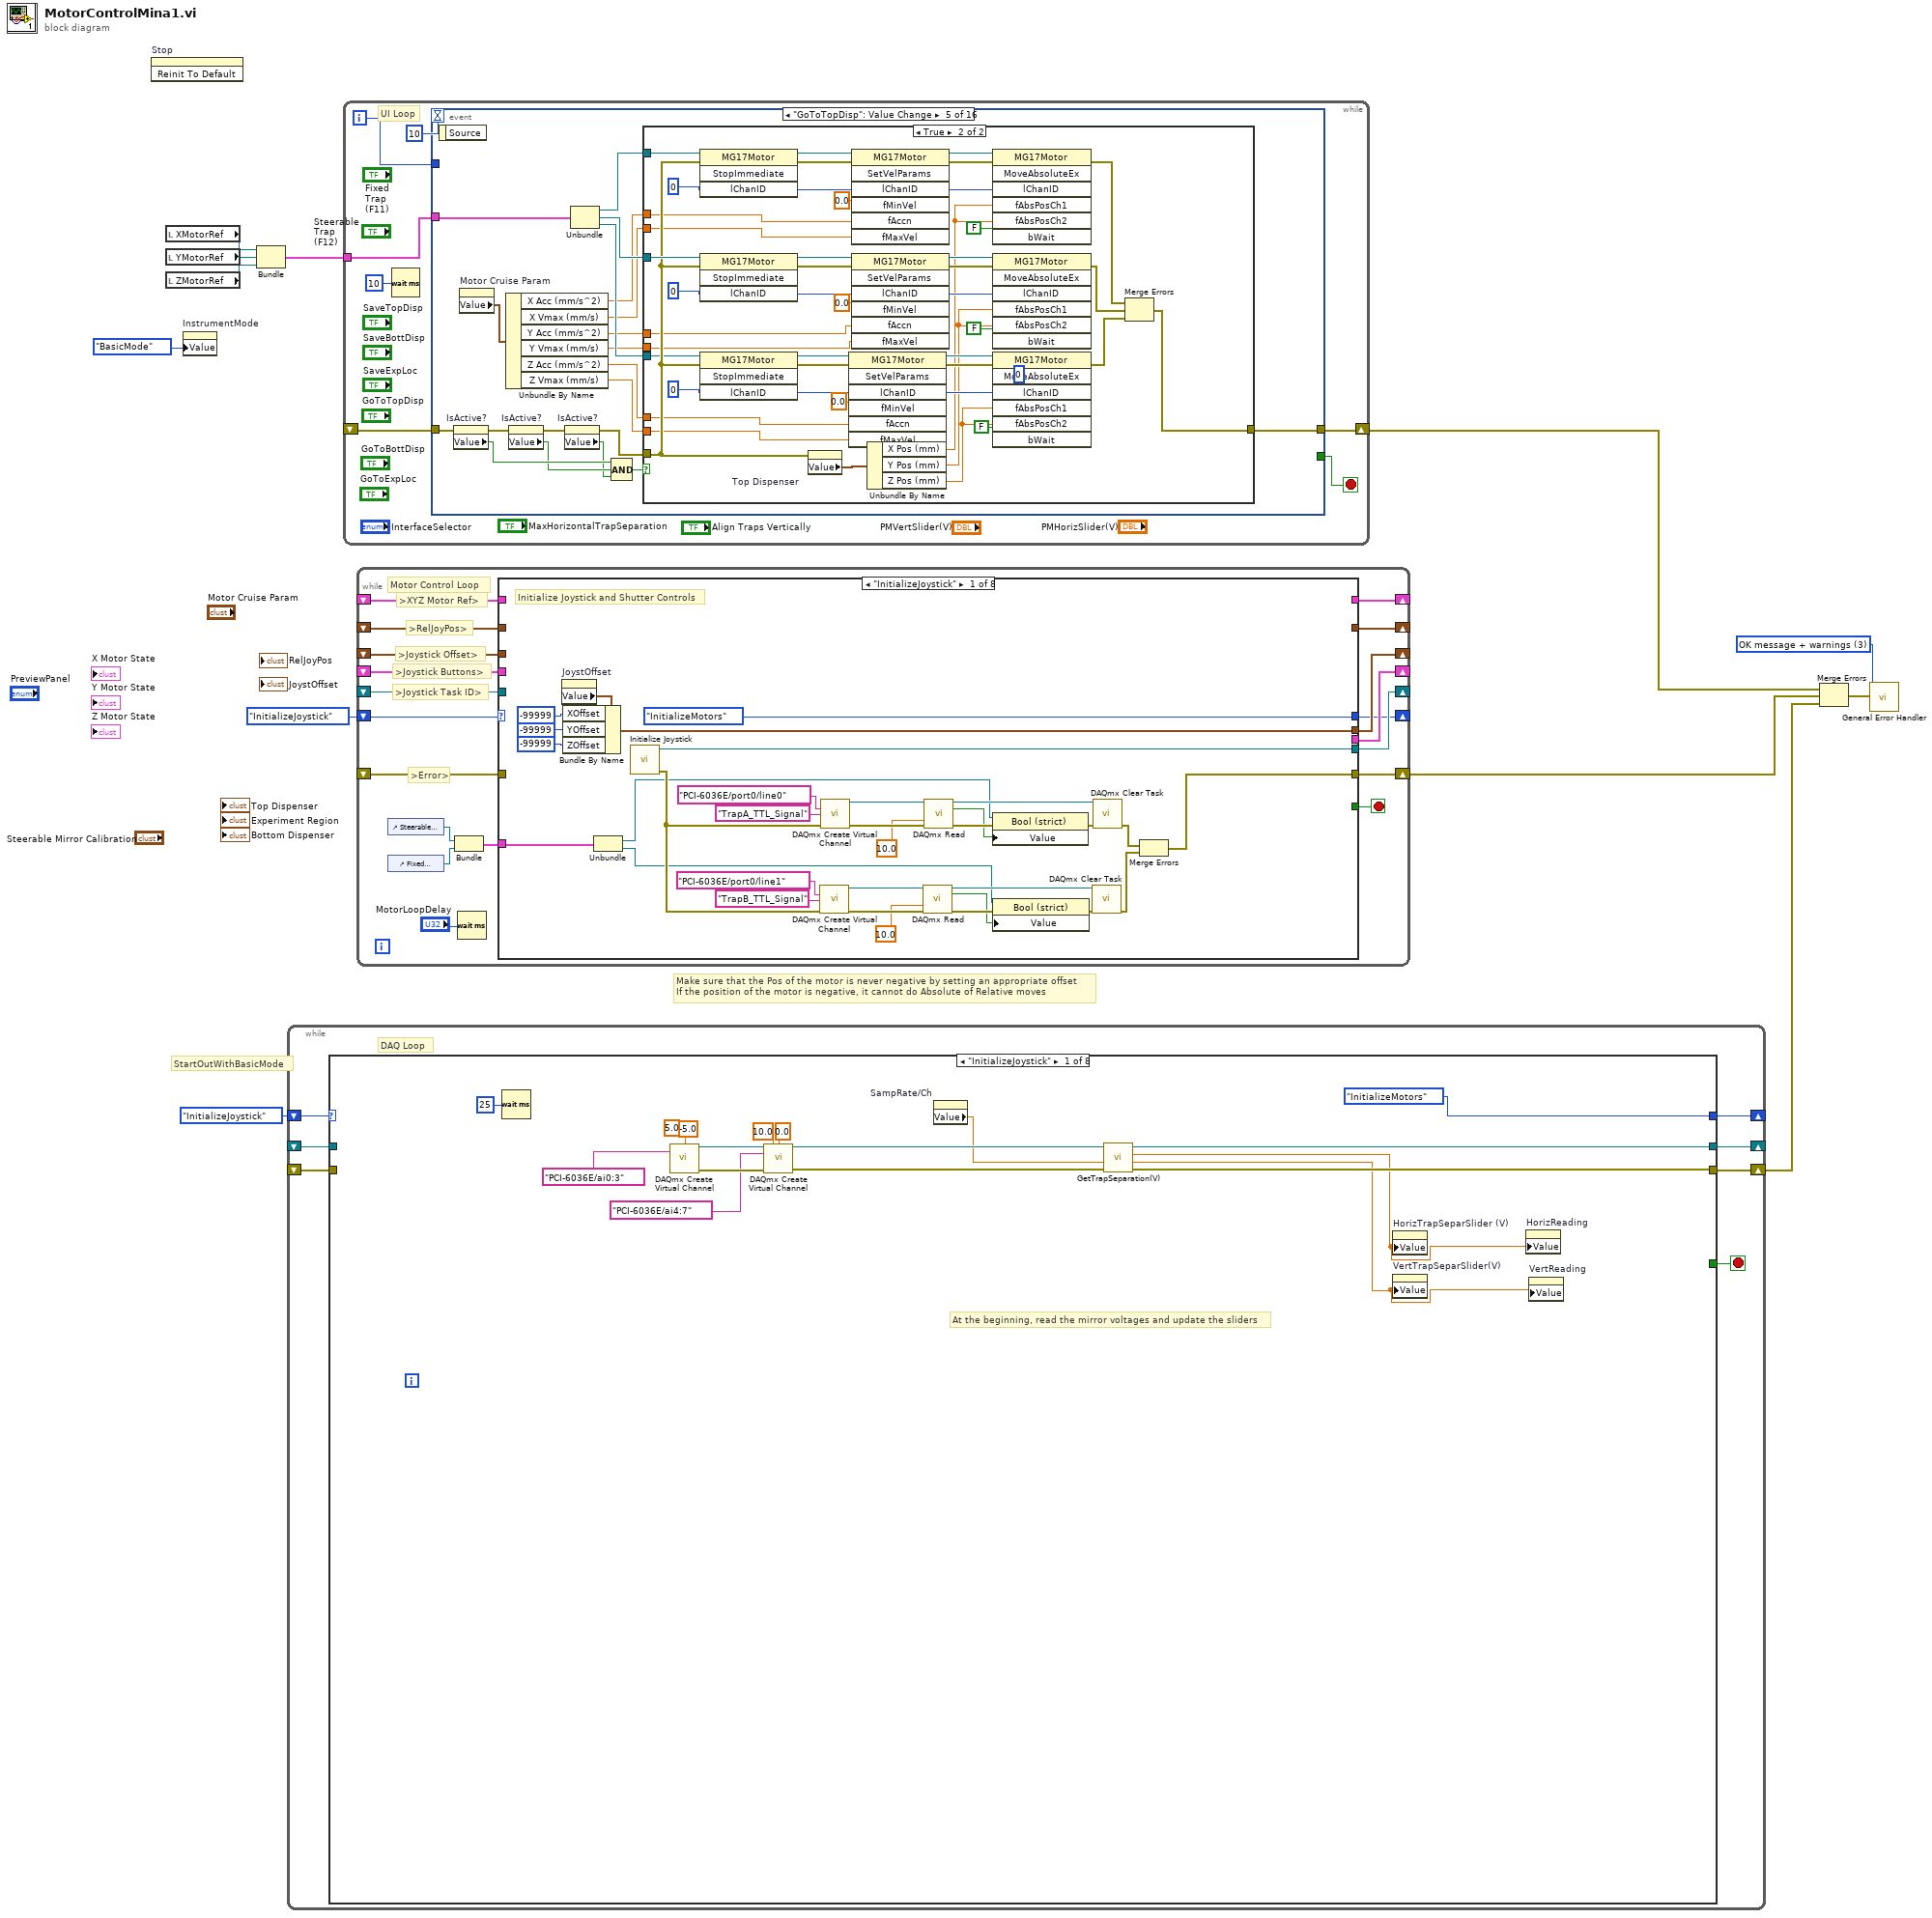
[diagram p0: block diagram]
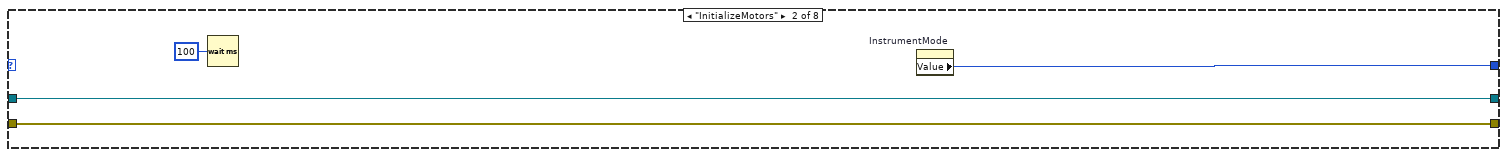
[diagram p2: hidden frame]
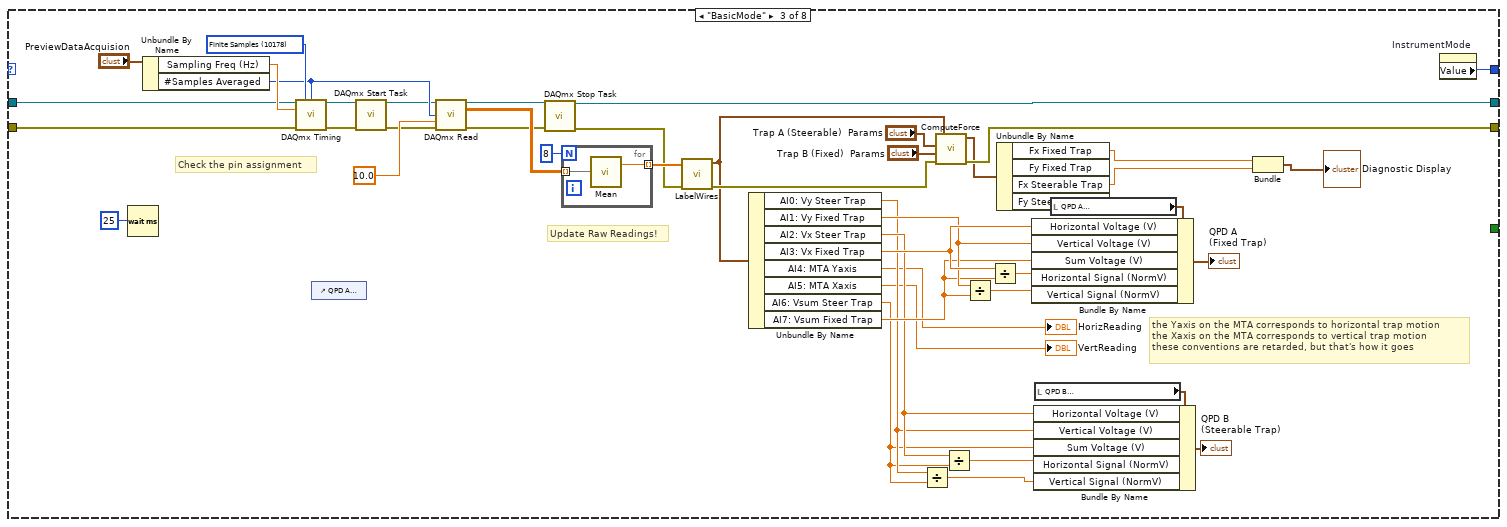
[diagram p3: hidden frame]
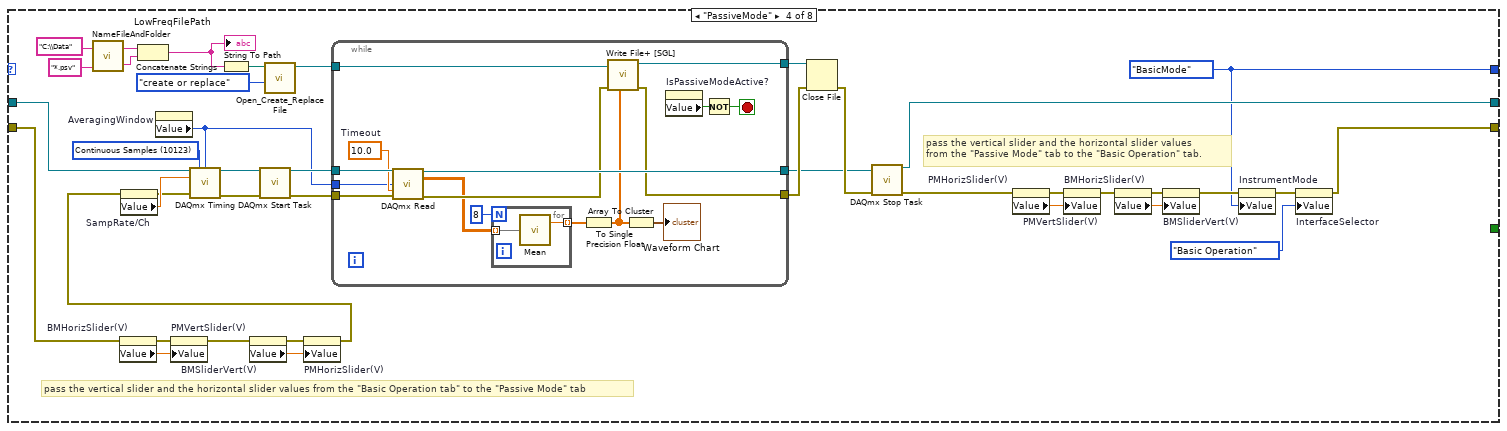
[diagram p4: hidden frame]
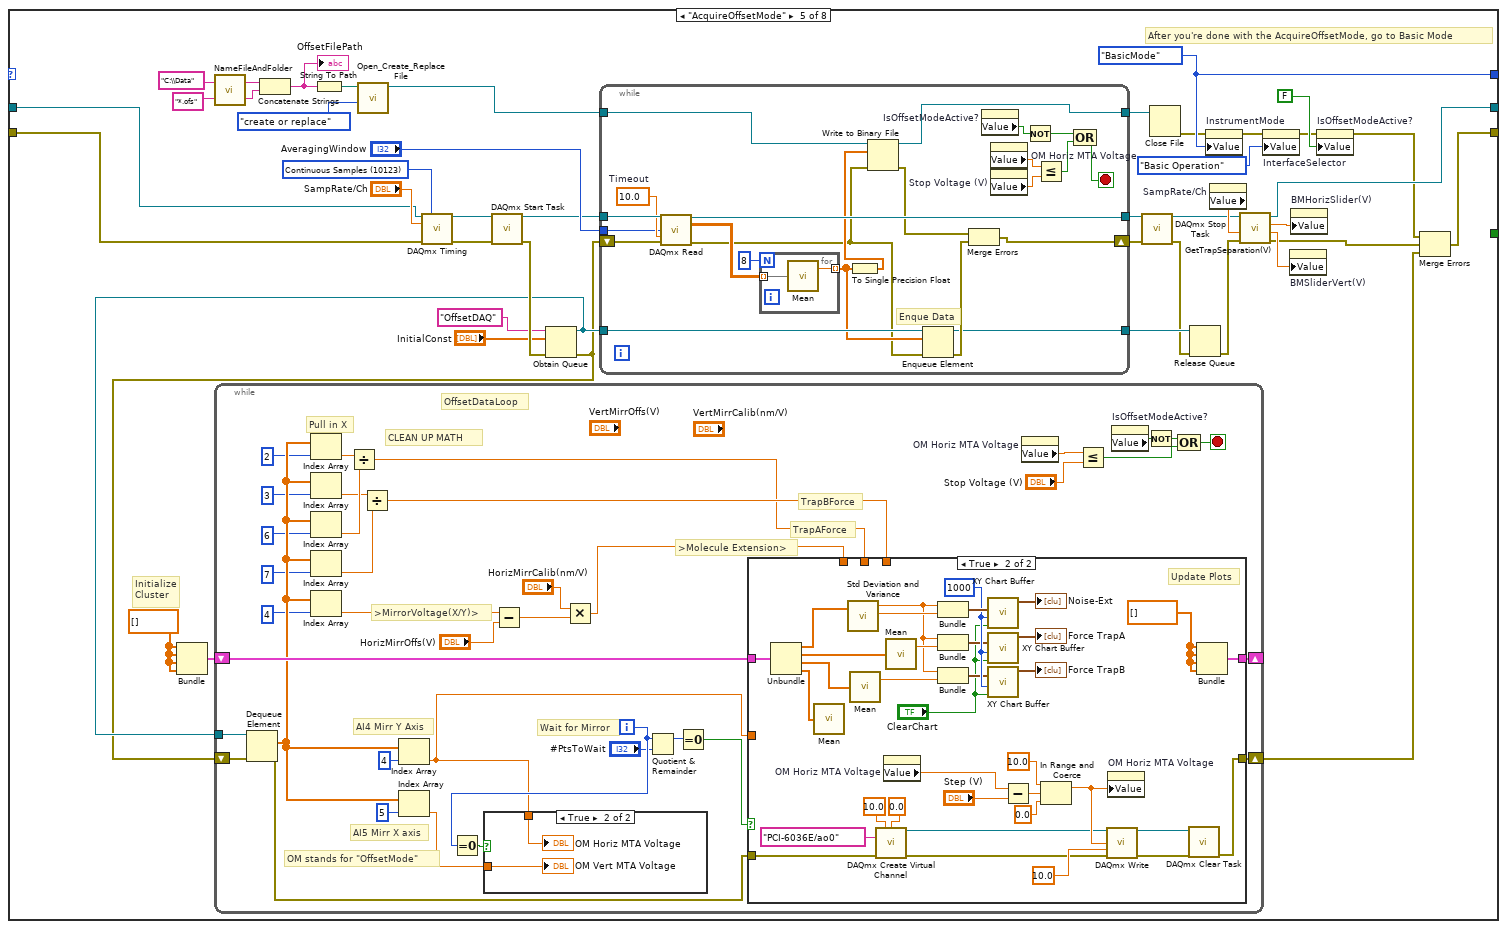
[diagram p5: hidden frame]
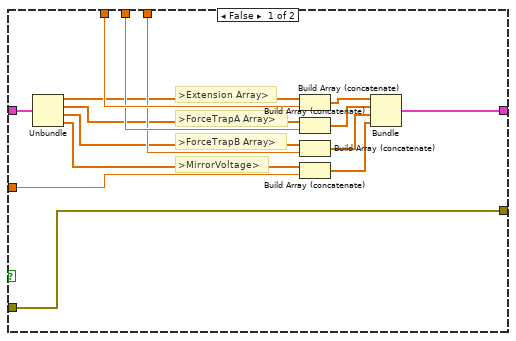
[diagram p7: hidden frame]
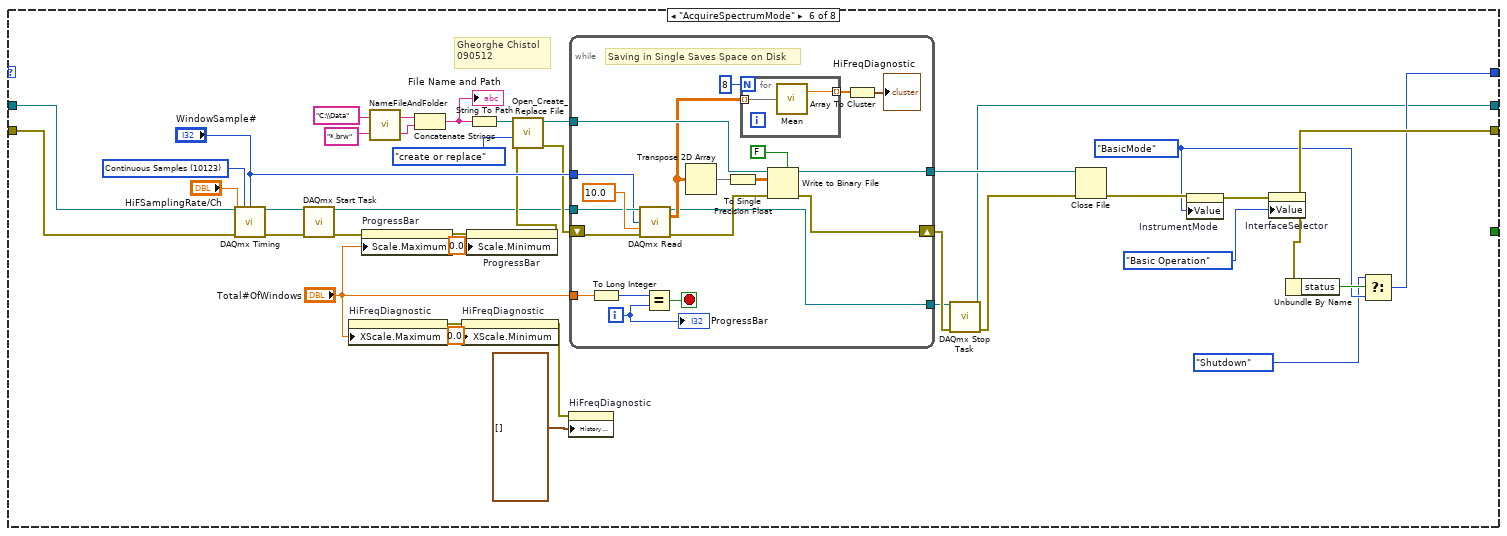
[diagram p8: hidden frame]
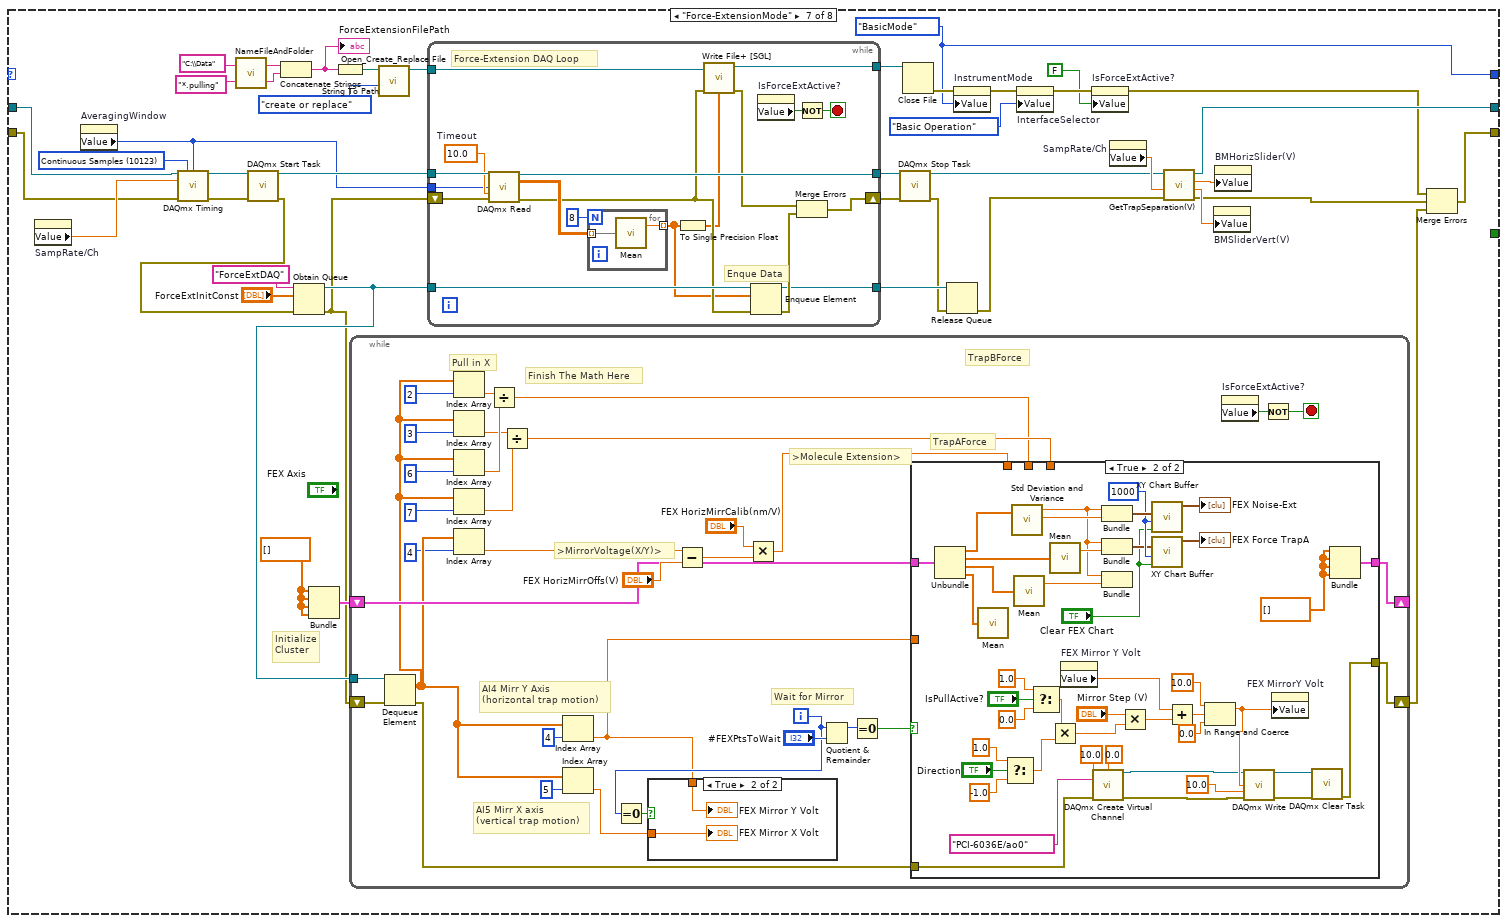
[diagram p9: hidden frame]
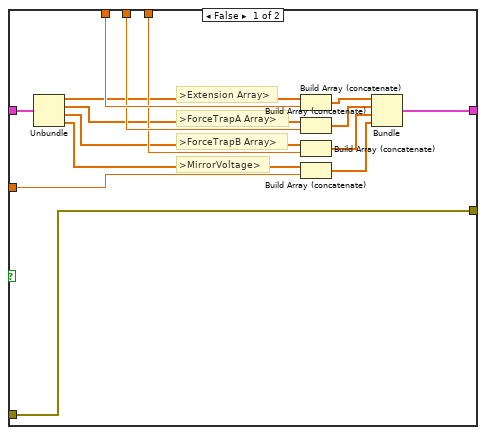
[diagram p11: hidden frame]
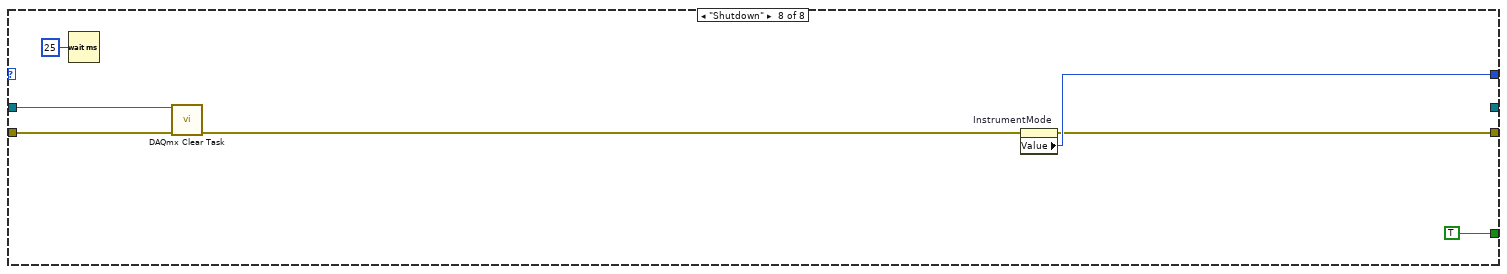
[diagram p12: hidden frame]
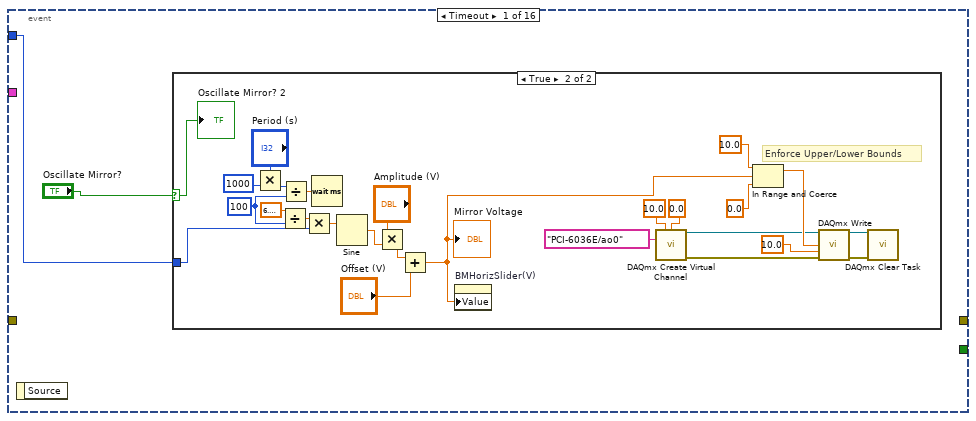
[diagram p13: hidden frame]
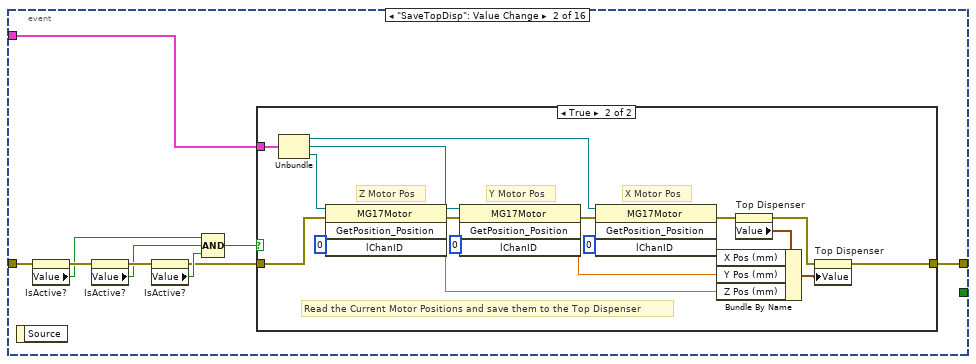
[diagram p15: hidden frame]
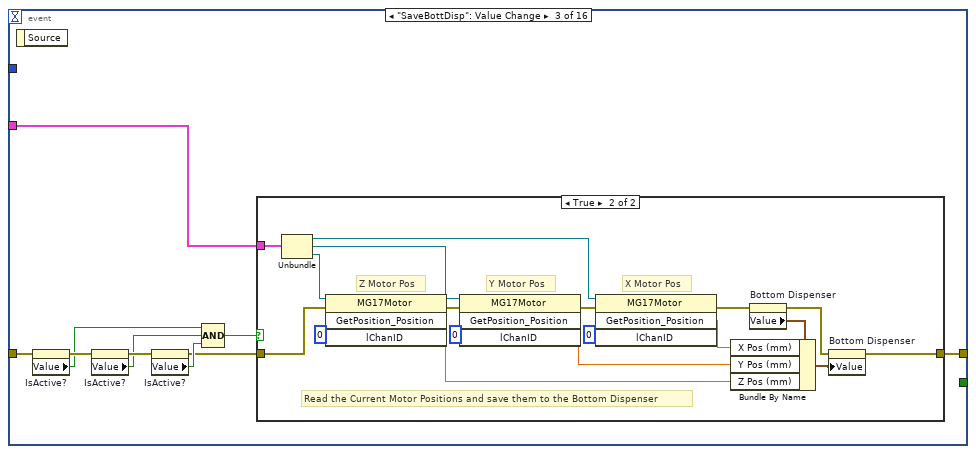
[diagram p17: hidden frame]
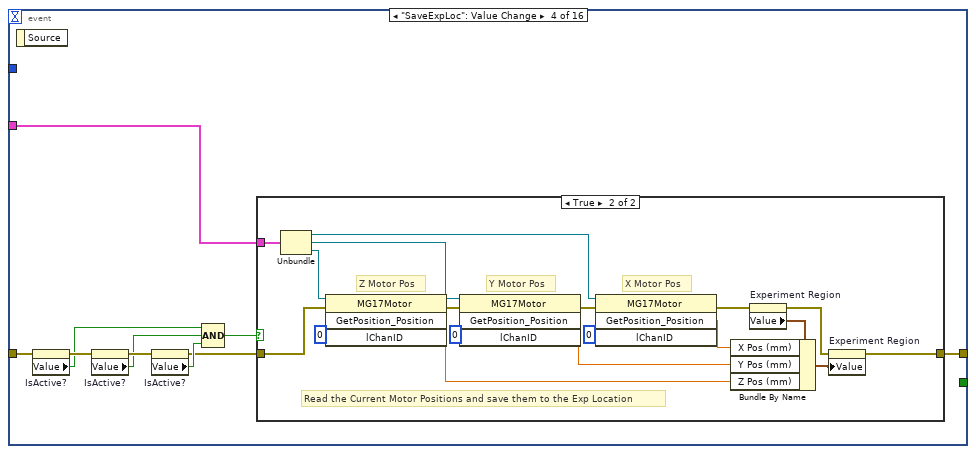
[diagram p19: hidden frame]
diagram:
  w2 = T17 3 items=["no dialog", "OK message", "continue or stop message", "OK message + warnings", "continue/stop + warnings"] ("type of dialog (OK msg:1)")
  # "StartOutWithBasicMode"
  # "Make sure that the Pos of the motor is never negative by setting an appropriate offset\nIf the position of the motor is negative, it cannot do Absolute of Relative moves"
  n1 = invoke on="Stop" class="Bool" method="Reinit To Default"() -> ()  [unwired: 3 in, 3 out]
  n2 = local read "XMotorRef"() -> (w12:refnum<k7>)
  n3 = local read "YMotorRef"() -> (w11:refnum<k7>)
  n4 = local read "ZMotorRef"() -> (w10:refnum<k7>)
  n5 = property on="InstrumentMode" class="Enum (strict)"("Value"=T1."BasicMode") -> ()  [unwired: 2 in, 2 out]
  n6 = Bundle("XMotorRef"=w12, "YMotorRef"=w11, "ZMotorRef"=w10) -> (w9:T18)  [unwired: 1 in]
  n7 = while {
    shift-right: [w14] -> _
    shift-left: T1."InitializeJoystick" ("Value") -> [w15]
    shift-right: [w17] -> w7
    shift-left: _ -> [w18]
    shift-right: [w13] -> _
    shift-left: _ -> [w19]
    stop <- w16 stop-if-true
    # "DAQ Loop"
    n8 = case shown="\"InitializeJoystick\"" w15 {
      tunnel: w19 -> [_ w37 w67 w109 w157 w305 w379 w524]
      tunnel: w18 -> [_ w36 w79 w100 w170 w324 w387 w527]
      tunnel: [w23 w36 w49 w87 w145 w319 w366 w525] -> w17
      tunnel: [_ _ _ _ _ _ _ TRUE] -> w16
      tunnel: [T1."InitializeMotors" ("Value") w38 w77 w88 w162 w315 w376 w529] -> w14
      tunnel: [w24 w37 w66 w106 w150 w304 w370 _] -> w13
      frame "InitializeJoystick" {
        (unwired) 5.0 ("Maximum Value")
        # "At the beginning, read the mirror voltages and update the sliders"
        n9 = Wait (ms)(milliseconds to wait=u32 25) -> ()  [unwired: 1 out]
        n10 = call-poly <vilib>:"DAQmx Create Virtual Channel.vi"("minimum value"=-5.0 ("Minimum Value"), "physical channels"=tag "PCI-6036E/ai0:3" ("Physical Channel")) -> ("task out"=w32:refnum<k21>, "error out"=w31:errorcluster)  [unwired: 12 in]
        n11 = call-poly <vilib>:"DAQmx Create Virtual Channel.vi"("task in"=w32, "maximum value"=10.0, "minimum value"=0.0, "physical channels"=tag "PCI-6036E/ai4:7", "error in"=w31) -> ("task out"=w27:refnum<k21>, "error out"=w26:errorcluster)  [unwired: 9 in]
        n12 = property on="SampRate/Ch" class="DigNum (strict)"() -> ("Value"=w25:dbl)  [unwired: 2 in, 2 out]
        n13 = call "GetTrapSeparation(V).vi"("ErrorIn"=w26, "AcquisitionRatePerChannel"=w25, "DAQ Task"=w27) -> ("ErrorOut"=w23:errorcluster, "VertTrapSeparation(V)"=w21:dbl, "HorTrapSeparation(V)"=w22:dbl, "DAQ Task"=w24:refnum<k21>)  [unwired: 1 in]
        n14 = property on="HorizTrapSeparSlider (V)" class="Slide (strict)"("Value"=w22) -> ()  [unwired: 2 in, 2 out]
        n15 = property on="VertTrapSeparSlider(V)" class="Slide (strict)"("Value"=w21) -> ()  [unwired: 2 in, 2 out]
        n16 = property on="HorizReading" class="DigNum (strict)"("Value"=w22) -> ()  [unwired: 2 in, 2 out]
        n17 = property on="VertReading" class="DigNum (strict)"("Value"=w21) -> ()  [unwired: 2 in, 2 out]
      }
      frame "InitializeMotors" {
        n18 = Wait (ms)(milliseconds to wait=u32 100) -> ()  [unwired: 1 out]
        n19 = property on="InstrumentMode" class="Enum (strict)"() -> ("Value"=w38:T1)  [unwired: 2 in, 2 out]
      }
      frame "BasicMode" {
        w78 = 10178 items=["Finite Samples"=10178, "Continuous Samples"=10123, "Hardware Timed Single Point"=12522] ("sample mode")
        # "the Yaxis on the MTA corresponds to horizontal trap motion\nthe Xaxis on the MTA corresponds to vertical trap motion\nthese conventions are retarded, but that's how it goes"
        # "Update Raw Readings!"
        # "Check the pin assignment"
        n20 = Wait (ms)(milliseconds to wait=u32 25) -> ()  [unwired: 1 out]
        n21 = Unbundle By Name("PreviewDataAcquision") -> ("Sampling Freq (Hz)"=w82:dbl, "#Samples Averaged"=w76:i32)
        n22 = call-poly <vilib>:"DAQmx Timing.vi"("task/channels in"=w67, "sample mode"=w78, "samples per channel"=w76, "rate"=w82, "error in"=w79) -> ("task out"=w74:refnum<k21>, "error out"=w73:errorcluster)  [unwired: 9 in]
        n23 = control-ref of="QPD A \n(Fixed Trap)"() -> ()  [unwired: 1 out]
        n24 = call <vilib>:"DAQmx Start Task.vi"("task/channels in"=w74, "error in"=w73) -> ("task out"=w72:refnum<k21>, "error out"=w71:errorcluster)  [unwired: 12 in]
        n25 = call-poly <vilib>:"DAQmx Read.vi"("task/channels in"=w72, "number of samples per channel"=w76, "timeout"=10.0, "error in"=w71) -> ("task out"=w70:refnum<k21>, "data"=w84:dbl[][], "error out"=w69:errorcluster)  [unwired: 9 in]
        n26 = call <vilib>:"DAQmx Stop Task.vi"("task/channels in"=w70, "error in"=w69) -> ("task out"=w66:refnum<k21>, "error out"=w65:errorcluster)  [unwired: 12 in]
        n27 = for {
          N: 8 -> [_]
          tunnel: w84 -> [w86] mode=indexing
          tunnel: [w85] -> w68 mode=indexing
          n28 = call-poly <vilib>:"Mean.vi"("X"=w86) -> ("mean"=w85:dbl)  [unwired: 1 out]
        }
        n29 = call "LabelWires.vi"("Error In"=w65, "DAQ Raw Measurement Array"=w68) -> ("Error Out"=w50:errorcluster, "Named DAQ Cluster"=w40:T21)  [unwired: 4 in]
        n30 = Unbundle By Name(w40) -> ("AI0: Vy Steer Trap"=w55:dbl, "AI1: Vy Fixed Trap"=w59:dbl, "AI2: Vx Steer Trap"=w56:dbl, "AI3: Vx Fixed Trap"=w60:dbl, "AI4: MTA Yaxis"=→"HorizReading":dbl, "AI5: MTA Xaxis"=→"VertReading":dbl, "AI6: Vsum Steer Trap"=w54:dbl, "AI7: Vsum Fixed Trap"=w58:dbl)
        n31 = Divide(x=w55, y=w54) -> (x/y=w53:dbl)
        n32 = call "ComputeForce.vi"("Error In"=w50, "Fixed Trap Params"="Trap B (Fixed)  Params", "Steerable Trap Params"="Trap A (Steerable)  Params", "Named DAQ Cluster"=w40) -> ("Error Out"=w49:errorcluster, "Computed Forces"=w44:T22)  [unwired: 2 out]
        n33 = Divide(x=w56, y=w54) -> (x/y=w45:dbl)
        n34 = Divide(x=w59, y=w58) -> (x/y=w57:dbl)
        n35 = Divide(x=w60, y=w58) -> (x/y=w46:dbl)
        n36 = Unbundle By Name(w44) -> ("Fx Fixed Trap"=w43:dbl, "Fx Steerable Trap"=w42:dbl)  [unwired: 2 out]
        n37 = local read "QPD B \n(Steerable Trap)"() -> (w62:T7)
        n38 = Bundle By Name(cluster=w62, "Horizontal Voltage (V)"=w56, "Vertical Voltage (V)"=w55, "Sum Voltage (V)"=w54, "Horizontal Signal (NormV)"=w45, "Vertical Signal (NormV)"=w53) -> (→"QPD B \n(Steerable Trap)":T7)
        n39 = local read "QPD A \n(Fixed Trap)"() -> (w64:T7)
        n40 = Bundle By Name(cluster=w64, "Horizontal Voltage (V)"=w60, "Vertical Voltage (V)"=w59, "Sum Voltage (V)"=w58, "Horizontal Signal (NormV)"=w46, "Vertical Signal (NormV)"=w57) -> (→"QPD A \n(Fixed Trap)":T7)
        n41 = Bundle("Fx Fixed Trap"=w43, "Fx Steerable Trap"=w42) -> (→"Diagnostic Display":T23)  [unwired: 1 in]
        n42 = property on="InstrumentMode" class="Enum (strict)"() -> ("Value"=w77:T1)  [unwired: 2 in, 2 out]
      }
      frame "PassiveMode" {
        w88 = T1."BasicMode" ("Value")
        w113 = 10123 items=["Finite Samples"=10178, "Continuous Samples"=10123] ("sample mode")
        # "pass the vertical slider and the horizontal slider values \nfrom the \"Passive Mode\" tab to the \"Basic Operation\" tab."
        # "pass the vertical slider and the horizontal slider values from the \"Basic Operation tab\" to the \"Passive Mode\" tab"
        n43 = call "NameFileAndFolder.vi"("ext"="*.psv", "Head Directory"="C:\\Data" ("path")) -> ("New Filename"=w123:string, "Sub Directory"=w124:string)
        n44 = property on="BMHorizSlider(V)" class="Slide (strict)"(error in=w100) -> (error out=w103:errorcluster, "Value"=w105:dbl)  [unwired: 1 in, 1 out]
        n45 = Concatenate Strings(w124, w123) -> (w120:string)
        "LowFreqFilePath" <- w120
        n46 = property on="AveragingWindow" class="DigNum (strict)"() -> ("Value"=w108:i32)  [unwired: 2 in, 2 out]
        n47 = property on="PMVertSlider(V)" class="Slide (strict)"(error in=w103, "Value"=w105) -> (error out=w102:errorcluster)  [unwired: 1 in, 1 out]
        n48 = String To Path(string=w120) -> (path=w125:path)
        n49 = property on="BMSliderVert(V)" class="Slide (strict)"(error in=w102) -> (error out=w101:errorcluster, "Value"=w104:dbl)  [unwired: 1 in, 1 out]
        n50 = call <vilib>:"Open_Create_Replace File.vi"("function (open:0)"=T19."create or replace", "file path"=w125) -> ("refnum"=w117:refnum<file>)  [unwired: 6 in, 3 out]
        n51 = property on="PMHorizSlider(V)" class="Slide (strict)"(error in=w101, "Value"=w104) -> (error out=w99:errorcluster)  [unwired: 1 in, 1 out]
        n52 = property on="SampRate/Ch" class="DigNum (strict)"(error in=w99) -> (error out=w98:errorcluster, "Value"=w107:dbl)  [unwired: 1 in, 1 out]
        n53 = call-poly <vilib>:"DAQmx Timing.vi"("task/channels in"=w109, "sample mode"=w113, "samples per channel"=w108, "rate"=w107, "error in"=w98) -> ("task out"=w118:refnum<k21>, "error out"=w119:errorcluster)  [unwired: 9 in]
        n54 = call <vilib>:"DAQmx Start Task.vi"("task/channels in"=w118, "error in"=w119) -> ("task out"=w111:refnum<k21>, "error out"=w110:errorcluster)  [unwired: 12 in]
        n55 = while {
          tunnel: w110 -> [w142]
          tunnel: w111 -> [w141]
          tunnel: [w140] -> w112
          tunnel: w117 -> [w138]
          tunnel: [w137] -> w114
          tunnel: [w135] -> w116
          tunnel: w108 -> [w129]
          stop <- w127 stop-if-true
          w139 = 10.0  # Timeout
          n56 = call-poly <vilib>:"DAQmx Read.vi"("task/channels in"=w141, "number of samples per channel"=w129, "timeout"=w139, "error in"=w142) -> ("task out"=w140:refnum<k21>, "data"=w132:dbl[][], "error out"=w136:errorcluster)  [unwired: 9 in]
          n57 = for {
            N: 8 -> [_]
            tunnel: [w144] -> w133 mode=indexing
            tunnel: w132 -> [w143] mode=indexing
            n58 = call-poly <vilib>:"Mean.vi"("X"=w143) -> ("mean"=w144:dbl)  [unwired: 1 out]
          }
          n59 = To Single Precision Float(number=w133) -> (single precision float=w130:sgl[])
          n60 = call <vilib>:"Write File+ [SGL].vi"("1D array"=w130, "error in (no error)"=w136, "refnum"=w138) -> ("error out"=w135:errorcluster, "dup refnum"=w137:refnum<file>)  [unwired: 6 in, 1 out]
          n61 = Array To Cluster(array=w130) -> (cluster=→"Waveform Chart":T15)
          n62 = property on="IsPassiveModeActive?" class="Bool (strict)"() -> ("Value"=w128:bool)  [unwired: 2 in, 2 out]
          n63 = Not(x=w128) -> (.not. x?=w127:bool)
        }
        n64 = Close File(refnum=w114, error in=w116) -> (error out=w115:errorcluster)  [unwired: 1 out]
        n65 = call <vilib>:"DAQmx Stop Task.vi"("task/channels in"=w112, "error in"=w115) -> ("task out"=w106:refnum<k21>, "error out"=w92:errorcluster)  [unwired: 12 in]
        n66 = property on="PMHorizSlider(V)" class="Slide (strict)"(error in=w92) -> (error out=w95:errorcluster, "Value"=w97:dbl)  [unwired: 1 in, 1 out]
        n67 = property on="BMHorizSlider(V)" class="Slide (strict)"(error in=w95, "Value"=w97) -> (error out=w94:errorcluster)  [unwired: 1 in, 1 out]
        n68 = property on="PMVertSlider(V)" class="Slide (strict)"(error in=w94) -> (error out=w93:errorcluster, "Value"=w96:dbl)  [unwired: 1 in, 1 out]
        n69 = property on="BMSliderVert(V)" class="Slide (strict)"(error in=w93, "Value"=w96) -> (error out=w89:errorcluster)  [unwired: 1 in, 1 out]
        n70 = property on="InstrumentMode" class="Enum (strict)"(error in=w89, "Value"=w88) -> (error out=w90:errorcluster)  [unwired: 1 in, 1 out]
        n71 = property on="InterfaceSelector" class="TabCtl (strict)"(error in=w90, "Value"=T4."Basic Operation" ("InterfaceSelector")) -> (error out=w87:errorcluster)  [unwired: 1 in, 1 out]
      }
      frame "AcquireOffsetMode" {
        w162 = T1."BasicMode" ("Value")
        w165 = dbl[] []
        w172 = 10123 items=["Finite Samples"=10178, "Continuous Samples"=10123] ("sample mode")
        # "Initialize\nCluster"
        # "After you're done with the AcquireOffsetMode, go to Basic Mode"
        n72 = Bundle(w165, w165, w165, w165) -> (w166:cluster{dbl[], dbl[], dbl[], dbl[]})  [unwired: 1 in]
        n73 = call "NameFileAndFolder.vi"("ext"="*.ofs", "Head Directory"="C:\\Data" ("path")) -> ("New Filename"=w179:string, "Sub Directory"=w180:string)
        n74 = Concatenate Strings(w180, w179) -> (w176:string)
        "OffsetFilePath" <- w176
        n75 = String To Path(string=w176) -> (path=w181:path)
        n76 = call <vilib>:"Open_Create_Replace File.vi"("function (open:0)"=T19."create or replace", "file path"=w181) -> ("refnum"=w173:refnum<file>)  [unwired: 6 in, 3 out]
        n77 = call-poly <vilib>:"DAQmx Timing.vi"("task/channels in"=w157, "sample mode"=w172, "rate"="SampRate/Ch", "error in"=w170) -> ("task out"=w174:refnum<k21>, "error out"=w175:errorcluster)  [unwired: 10 in]
        n78 = call <vilib>:"DAQmx Start Task.vi"("task/channels in"=w174, "error in"=w175) -> ("task out"=w171:refnum<k21>, "error out"=w188:errorcluster)  [unwired: 12 in]
        n79 = Obtain Queue(name (unnamed)="OffsetDAQ", element data type="InitialConst", error in (no error)=w188) -> (queue out=w164:refnum<queue>, error out=w163:errorcluster)  [unwired: 2 in, 1 out]
        n80 = while {
          shift-right: [w224] -> w146
          shift-left: w163 -> [w191]
          shift-right: [w226] -> _
          shift-left: w166 -> [w225]
          tunnel: w164 -> [w192]
          i -> [w223]
          stop <- w222 stop-if-true
          # "OM stands for \"OffsetMode\""
          # "Pull in X"
          # "AI5 Mirr X axis"
          # "AI4 Mirr Y Axis"
          # "CLEAN UP MATH"
          # ">Molecule Extension>"
          # "TrapBForce"
          # "TrapAForce"
          # ">MirrorVoltage(X/Y)>"
          # "Wait for Mirror"
          # "OffsetDataLoop"
          n81 = Dequeue Element(queue=w192, error in (no error)=w191) -> (element=w206:dbl[], error out=w213:errorcluster)  [unwired: 1 in, 2 out]
          n82 = Index Array(array=w206, index=2) -> (element=w199:dbl)
          n83 = Index Array(array=w206, index=3) -> (element=w197:dbl)
          n84 = Index Array(array=w206, index=6) -> (element=w198:dbl)
          n85 = Index Array(array=w206, index=7) -> (element=w196:dbl)
          n86 = Index Array(array=w206, index=4) -> (element=w219:dbl)
          n87 = Divide(x=w199, y=w198) -> (x/y=w212:dbl)
          n88 = Divide(x=w197, y=w196) -> (x/y=w215:dbl)
          n89 = Index Array(array=w206, index=4) -> (element=w209:dbl)
          n90 = Index Array(array=w206, index=5) -> (element=w205:dbl)
          n91 = Equal To 0?(x=w223) -> (x = 0?=w210:bool)
          n92 = case shown="True" w210 {
            tunnel: w209 -> [_ w228]
            tunnel: w205 -> [_ w227]
            frame False {
            }
            frame True {
              "OM Horiz MTA Voltage" <- w228
              "OM Vert MTA Voltage" <- w227
            }
          }
          n93 = Subtract(x=w219, y="HorizMirrOffs(V)") -> (x-y=w217:dbl)
          n94 = Multiply(x="HorizMirrCalib(nm/V)", y=w217) -> (x*y=w214:dbl)
          n95 = Quotient & Remainder(x=w223, y="#PtsToWait") -> (x-y*floor(x/y)=w220:i32)  [unwired: 1 out]
          n96 = Equal To 0?(x=w220) -> (x = 0?=w211:bool)
          n97 = case shown="True" w211 {
            tunnel: w214 -> [w243 _]
            tunnel: w212 -> [w242 _]
            tunnel: w215 -> [w241 _]
            tunnel: w209 -> [w240 _]
            tunnel: [w239 w258] -> w224
            tunnel: w213 -> [w239 w259]
            tunnel: [w233 w265] -> w226
            tunnel: w225 -> [w232 w271]
            frame False {
              # ">MirrorVoltage>"
              # ">ForceTrapB Array>"
              # ">ForceTrapA Array>"
              # ">Extension Array>"
              n98 = Unbundle(w232) -> (w234:dbl[], w231:dbl[], w230:dbl[], w229:dbl[])
              n99 = Build Array (concatenate)(w234, w243) -> (w238:dbl[])
              n100 = Build Array (concatenate)(w231, w242) -> (w237:dbl[])
              n101 = Build Array (concatenate)(w230, w241) -> (w236:dbl[])
              n102 = Build Array (concatenate)(w229, w240) -> (w235:dbl[])
              n103 = Bundle(w238, w237, w236, w235) -> (w233:cluster{dbl[], dbl[], dbl[], dbl[]})  [unwired: 1 in]
            }
            frame True {
              w266 = dbl[] []
              w254 = 1000 ("chart length (points)")
              # "Update Plots"
              n104 = Unbundle(w271) -> (w270:dbl[], w269:dbl[], w268:dbl[], w267:dbl[])
              n105 = call-poly <vilib>:"Mean.vi"("X"=w267) -> ()  [unwired: 2 out]
              n106 = call <vilib>:"Std Deviation and Variance.vi"("X"=w270) -> ("mean"=w272:dbl, "standard deviation"=w273:dbl)  [unwired: 1 in, 1 out]
              n107 = call-poly <vilib>:"Mean.vi"("X"=w268) -> ("mean"=w278:dbl)  [unwired: 1 out]
              n108 = call-poly <vilib>:"DAQmx Create Virtual Channel.vi"("maximum value"=10.0 ("Maximum Value"), "minimum value"=0.0 ("Minimum Value"), "physical channels"=tag "PCI-6036E/ao0", "error in"=w259) -> ("task out"=w245:refnum<k21>, "error out"=w244:errorcluster)  [unwired: 10 in]
              n109 = property on="OM Horiz MTA Voltage" class="DigNum (strict)"() -> ("Value"=w249:dbl)  [unwired: 2 in, 2 out]
              n110 = call-poly <vilib>:"Mean.vi"("X"=w269) -> ("mean"=w277:dbl)  [unwired: 1 out]
              n111 = Bundle("mean"=w272, "standard deviation"=w273) -> (w255:cluster{"mean":dbl, "standard deviation":dbl})  [unwired: 1 in]
              n112 = Bundle("mean"=w272, "mean"=w277) -> (w252:cluster{"mean":dbl, "mean":dbl})  [unwired: 1 in]
              n113 = Bundle("mean"=w272, "mean"=w278) -> (w253:cluster{"mean":dbl, "mean":dbl})  [unwired: 1 in]
              n114 = call "XY Chart Buffer.vi"("clear first (no:F)"="ClearChart", "chart length (points)"=w254, "new point"=w255) -> ("XY chart data"=→"Noise-Ext":cluster{"x":dbl, "y":dbl}[])  [unwired: 8 in]
              n115 = call "XY Chart Buffer.vi"("clear first (no:F)"="ClearChart", "chart length (points)"=w254, "new point"=w252) -> ("XY chart data"=→"Force TrapA":cluster{"x":dbl, "y":dbl}[])  [unwired: 8 in]
              n116 = call "XY Chart Buffer.vi"("clear first (no:F)"="ClearChart", "chart length (points)"=w254, "new point"=w253) -> ("XY chart data"=→"Force TrapB":cluster{"x":dbl, "y":dbl}[])  [unwired: 8 in]
              n117 = Subtract(x=w249, y="Step (V)") -> (x-y=w276:dbl)
              n118 = In Range and Coerce(upper limit=10.0, x=w276, lower limit=0.0 ("upper limit")) -> (coerced(x)=w257:dbl)  [unwired: 1 out]
              n119 = call-poly <vilib>:"DAQmx Write.vi"("task/channels in"=w245, "data"=w257, "timeout"=10.0, "error in"=w244) -> ("task out"=w263:refnum<k21>, "error out"=w264:errorcluster)  [unwired: 9 in, 1 out]
              n120 = property on="OM Horiz MTA Voltage" class="DigNum (strict)"("Value"=w257) -> ()  [unwired: 2 in, 2 out]
              n121 = call <vilib>:"DAQmx Clear Task.vi"("task in"=w263, "error in"=w264) -> ("error out"=w258:errorcluster)  [unwired: 13 in]
              n122 = Bundle(w266, w266, w266, w266) -> (w265:cluster{dbl[], dbl[], dbl[], dbl[]})  [unwired: 1 in]
            }
          }
          n123 = property on="OM Horiz MTA Voltage" class="DigNum (strict)"() -> ("Value"=w193:dbl)  [unwired: 2 in, 2 out]
          n124 = Less Or Equal?(x=w193, y="Stop Voltage (V)") -> (x <= y?=w195:bool)
          n125 = property on="IsOffsetModeActive?" class="Bool (strict)"() -> ("Value"=w190:bool)  [unwired: 2 in, 2 out]
          n126 = Not(x=w190) -> (.not. x?=w189:bool)
          n127 = Compound Arithmetic op=OR(w189, w195) -> (w222:bool)
        }
        n128 = while {
          tunnel: w171 -> [w300]
          tunnel: [w299] -> w169
          tunnel: w173 -> [w290]
          tunnel: "AveragingWindow" -> [w295]
          tunnel: w164 -> [w294]
          shift-right: [w286] -> w168
          shift-left: w163 -> [w301]
          tunnel: [w292] -> w187
          tunnel: [w285] -> w167
          stop <- w281 stop-if-true
          w298 = 10.0  # Timeout
          # "Enque Data"
          n129 = call-poly <vilib>:"DAQmx Read.vi"("task/channels in"=w300, "number of samples per channel"=w295, "timeout"=w298, "error in"=w301) -> ("task out"=w299:refnum<k21>, "data"=w296:dbl[][], "error out"=w288:errorcluster)  [unwired: 9 in]
          n130 = for {
            N: 8 -> [_]
            tunnel: [w303] -> w291 mode=indexing
            tunnel: w296 -> [w302] mode=indexing
            n131 = call-poly <vilib>:"Mean.vi"("X"=w302) -> ("mean"=w303:dbl)  [unwired: 1 out]
          }
          n132 = To Single Precision Float(number=w291) -> (single precision float=w289:sgl[])
          n133 = Write to Binary File(file (use dialog)=w290, data=w289, error in=w288) -> (refnum out=w285:refnum<file>, error out=w287:errorcluster)  [unwired: 3 in, 1 out]
          n134 = Enqueue Element(queue=w294, element=w291, error in (no error)=w288) -> (queue out=w292:refnum<queue>, error out=w293:errorcluster)  [unwired: 1 in, 1 out]
          n135 = Merge Errors(w287, w293) -> (w286:errorcluster)
          n136 = property on="IsOffsetModeActive?" class="Bool (strict)"() -> ("Value"=w280:bool)  [unwired: 2 in, 2 out]
          n137 = property on="OM Horiz MTA Voltage" class="DigNum (strict)"() -> ("Value"=w283:dbl)  [unwired: 2 in, 2 out]
          n138 = property on="Stop Voltage (V)" class="DigNum (strict)"() -> ("Value"=w284:dbl)  [unwired: 2 in, 2 out]
          n139 = Not(x=w280) -> (.not. x?=w279:bool)
          n140 = Less Or Equal?(x=w283, y=w284) -> (x <= y?=w282:bool)
          n141 = Compound Arithmetic op=OR(w279, w282) -> (w281:bool)
        }
        n142 = call <vilib>:"DAQmx Stop Task.vi"("task/channels in"=w169, "error in"=w168) -> ("task out"=w152:refnum<k21>, "error out"=w151:errorcluster)  [unwired: 12 in]
        n143 = Close File(refnum=w167) -> (error out=w156:errorcluster)  [unwired: 1 in, 1 out]
        n144 = Release Queue(queue=w187, error in (no error)=w151) -> (error out=w148:errorcluster)  [unwired: 1 in, 2 out]
        n145 = property on="InstrumentMode" class="Enum (strict)"(error in=w156, "Value"=w162) -> (error out=w160:errorcluster)  [unwired: 1 in, 1 out]
        n146 = property on="SampRate/Ch" class="DigNum (strict)"() -> ("Value"=w153:dbl)  [unwired: 2 in, 2 out]
        n147 = call "GetTrapSeparation(V).vi"("ErrorIn"=w148, "AcquisitionRatePerChannel"=w153, "DAQ Task"=w152) -> ("ErrorOut"=w149:errorcluster, "VertTrapSeparation(V)"=w155:dbl, "HorTrapSeparation(V)"=w154:dbl, "DAQ Task"=w150:refnum<k21>)  [unwired: 1 in]
        n148 = property on="InterfaceSelector" class="TabCtl (strict)"(error in=w160, "Value"=T4."Basic Operation" ("InterfaceSelector")) -> (error out=w158:errorcluster)  [unwired: 1 in, 1 out]
        n149 = property on="BMSliderVert(V)" class="Slide (strict)"("Value"=w155) -> ()  [unwired: 2 in, 2 out]
        n150 = property on="BMHorizSlider(V)" class="Slide (strict)"("Value"=w154) -> ()  [unwired: 2 in, 2 out]
        n151 = property on="IsOffsetModeActive?" class="Bool (strict)"(error in=w158, "Value"=FALSE ("IsOffsetModeActive?")) -> (error out=w147:errorcluster)  [unwired: 1 in, 1 out]
        n152 = Merge Errors(w147, w149, w146) -> (w145:errorcluster)
      }
      frame "AcquireSpectrumMode" {
        w317 = T1."BasicMode"
        w326 = 10123 items=["Finite Samples"=10178, "Continuous Samples"=10123] ("sample mode")
        # "Gheorghe Chistol\n090512"
        n153 = call-poly <vilib>:"DAQmx Timing.vi"("task/channels in"=w305, "sample mode"=w326, "samples per channel"="WindowSample#", "rate"="HiFSamplingRate/Ch", "error in"=w324) -> ("task out"=w309:refnum<k21>, "error out"=w308:errorcluster)  [unwired: 9 in]
        n154 = call <vilib>:"DAQmx Start Task.vi"("task/channels in"=w309, "error in"=w308) -> ("task out"=w307:refnum<k21>, "error out"=w310:errorcluster)  [unwired: 12 in]
        n155 = property on="HiFreqDiagnostic" class="WFChart (strict)"("XScale.Maximum"="Total#OfWindows") -> (error out=w339:errorcluster)  [unwired: 2 in, 1 out]
        n156 = property on="ProgressBar" class="Slide (strict)"(error in=w310, "Scale.Maximum"="Total#OfWindows") -> (error out=w336:errorcluster)  [unwired: 1 in, 1 out]
        n157 = call "NameFileAndFolder.vi"("ext"="*.brw", "Head Directory"="C:\\Data" ("path")) -> ("New Filename"=w330:string, "Sub Directory"=w331:string)
        n158 = Concatenate Strings(w331, w330) -> (w327:string)
        "File Name and Path" <- w327
        n159 = property on="HiFreqDiagnostic" class="WFChart (strict)"(error in=w339, "XScale.Minimum"=0.0 ("X Scale.Range:Minimum")) -> (error out=w342:errorcluster)  [unwired: 1 in, 1 out]
        n160 = property on="ProgressBar" class="Slide (strict)"(error in=w336, "Scale.Minimum"=0.0 ("Scale.Range:Minimum")) -> (error out=w314:errorcluster)  [unwired: 1 in, 1 out]
        n161 = String To Path(string=w327) -> (path=w332:path)
        n162 = call <vilib>:"Open_Create_Replace File.vi"("error in (no error)"=w314, "function (open:0)"=T19."create or replace", "file path"=w332) -> ("error out"=w313:errorcluster, "refnum"=w335:refnum<file>)  [unwired: 5 in, 2 out]
        n163 = property on="HiFreqDiagnostic" class="WFChart (strict)"(error in=w342, "History Data"=T20 []) -> ()  [unwired: 1 in, 2 out]
        n164 = while {
          tunnel: [w361] -> w325
          tunnel: w307 -> [w358]
          tunnel: w335 -> [w355]
          tunnel: "Total#OfWindows" -> [w354]
          shift-right: [w356] -> w312
          shift-left: w313 -> [w357]
          tunnel: "WindowSample#" -> [w344]
          tunnel: [w343] -> w311
          i -> [w351]
          stop <- w345 stop-if-true
          # "Saving in Single Saves Space on Disk"
          n165 = To Long Integer(number=w354) -> (32bit integer=w352:i32)
          n166 = call-poly <vilib>:"DAQmx Read.vi"("task/channels in"=w358, "number of samples per channel"=w344, "timeout"=10.0, "error in"=w357) -> ("task out"=w343:refnum<k21>, "data"=w348:dbl[][], "error out"=w360:errorcluster)  [unwired: 9 in]
          n167 = Equal?(x=w352, y=w351) -> (x = y?=w345:bool)
          n168 = Transpose 2D Array(2D array=w348) -> (transposed array=w347:dbl[][])
          n169 = To Single Precision Float(number=w347) -> (single precision float=w346:sgl[][])
          n170 = for {
            N: 8 -> [_]
            tunnel: [w364] -> w350 mode=indexing
            tunnel: w348 -> [w363] mode=indexing
            n171 = call-poly <vilib>:"Mean.vi"("X"=w363) -> ("mean"=w364:dbl)  [unwired: 1 out]
          }
          n172 = Write to Binary File(file (use dialog)=w355, data=w346, error in=w360, 5:FALSE ("prepend array or string size? (T)")) -> (refnum out=w361:refnum<file>, error out=w356:errorcluster)  [unwired: 2 in, 1 out]
          n173 = Array To Cluster(array=w350) -> (cluster=→"HiFreqDiagnostic":T16)
          "ProgressBar" <- w351
        }
        n174 = call <vilib>:"DAQmx Stop Task.vi"("task/channels in"=w311, "error in"=w312) -> ("task out"=w304:refnum<k21>, "error out"=w306:errorcluster)  [unwired: 12 in]
        n175 = Close File(refnum=w325, error in=w306) -> (error out=w323:errorcluster)  [unwired: 1 out]
        n176 = property on="InstrumentMode" class="Enum (strict)"(error in=w323, "Value"=w317) -> (error out=w321:errorcluster)  [unwired: 1 in, 1 out]
        n177 = property on="InterfaceSelector" class="TabCtl (strict)"(error in=w321, "Value"=T4."Basic Operation" ("InterfaceSelector")) -> (error out=w319:errorcluster)  [unwired: 1 in, 1 out]
        n178 = Unbundle By Name(w319) -> ("status"=w318:bool)
        n179 = Select(t=T1."Shutdown", s=w318, f=w317) -> (s? t:f=w315:T1)
      }
      frame "Force-ExtensionMode" {
        w376 = T1."BasicMode" ("InstrumentMode")
        w407 = dbl[] []
        w390 = 10123 items=["Finite Samples"=10178, "Continuous Samples"=10123] ("sample mode")
        # "Initialize\nCluster"
        n180 = property on="SampRate/Ch" class="DigNum (strict)"() -> ("Value"=w388:dbl)  [unwired: 2 in, 2 out]
        n181 = property on="AveragingWindow" class="DigNum (strict)"() -> ("Value"=w365:i32)  [unwired: 2 in, 2 out]
        n182 = call-poly <vilib>:"DAQmx Timing.vi"("task/channels in"=w379, "sample mode"=w390, "samples per channel"=w365, "rate"=w388, "error in"=w387) -> ("task out"=w393:refnum<k21>, "error out"=w394:errorcluster)  [unwired: 9 in]
        n183 = call "NameFileAndFolder.vi"("ext"="*.pulling", "Head Directory"="C:\\Data" ("path")) -> ("New Filename"=w398:string, "Sub Directory"=w399:string)
        n184 = call <vilib>:"DAQmx Start Task.vi"("task/channels in"=w393, "error in"=w394) -> ("task out"=w389:refnum<k21>, "error out"=w404:errorcluster)  [unwired: 12 in]
        n185 = Concatenate Strings(w399, w398) -> (w395:string)
        "ForceExtensionFilePath" <- w395
        n186 = Obtain Queue(name (unnamed)="ForceExtDAQ", element data type="ForceExtInitConst", error in (no error)=w404) -> (queue out=w406:refnum<queue>, error out=w386:errorcluster)  [unwired: 2 in, 1 out]
        n187 = Bundle(w407, w407, w407, w407) -> (w408:cluster{dbl[], dbl[], dbl[], dbl[]})  [unwired: 1 in]
        n188 = String To Path(string=w395) -> (path=w400:path)
        n189 = while {
          shift-right: [w450] -> w367
          shift-left: w386 -> [w432]
          tunnel: w406 -> [w457]
          shift-right: [w453] -> _
          shift-left: w408 -> [w452]
          i -> [w448]
          stop <- w430 stop-if-true
          # "Pull in X"
          # "AI5 Mirr X axis\n(vertical trap motion)"
          # "AI4 Mirr Y Axis\n(horizontal trap motion)"
          # "Finish The Math Here"
          # ">Molecule Extension>"
          # "TrapBForce"
          # "TrapAForce"
          # ">MirrorVoltage(X/Y)>"
          # "Wait for Mirror"
          n190 = Dequeue Element(queue=w457, error in (no error)=w432) -> (element=w443:dbl[], error out=w454:errorcluster)  [unwired: 1 in, 2 out]
          n191 = Index Array(array=w443, index=2) -> (element=w436:dbl)
          n192 = Index Array(array=w443, index=3) -> (element=w434:dbl)
          n193 = Index Array(array=w443, index=6) -> (element=w435:dbl)
          n194 = Index Array(array=w443, index=7) -> (element=w433:dbl)
          n195 = Index Array(array=w443, index=4) -> (element=w461:dbl)
          n196 = Divide(x=w436, y=w435) -> (x/y=w451:dbl)
          n197 = Divide(x=w434, y=w433) -> (x/y=w456:dbl)
          n198 = Index Array(array=w443, index=4) -> (element=w446:dbl)
          n199 = Index Array(array=w443, index=5) -> (element=w442:dbl)
          n200 = Equal To 0?(x=w448) -> (x = 0?=w447:bool)
          n201 = case shown="True" w447 {
            tunnel: w446 -> [_ w465]
            tunnel: w442 -> [_ w464]
            frame False {
            }
            frame True {
              "FEX Mirror Y Volt" <- w465
              "FEX Mirror X Volt" <- w464
            }
          }
          n202 = Subtract(x=w461, y="FEX HorizMirrOffs(V)") -> (x-y=w459:dbl)
          n203 = Multiply(x="FEX HorizMirrCalib(nm/V)", y=w459) -> (x*y=w455:dbl)
          n204 = Quotient & Remainder(x=w448, y="#FEXPtsToWait") -> (x-y*floor(x/y)=w462:i32)  [unwired: 1 out]
          n205 = Equal To 0?(x=w462) -> (x = 0?=w449:bool)
          n206 = case shown="True" w449 {
            tunnel: w455 -> [w480 _]
            tunnel: w451 -> [w479 _]
            tunnel: w456 -> [w478 _]
            tunnel: w446 -> [w477 _]
            tunnel: [w476 w492] -> w450
            tunnel: w454 -> [w476 w493]
            tunnel: [w470 w499] -> w453
            tunnel: w452 -> [w469 w505]
            frame False {
              # ">MirrorVoltage>"
              # ">ForceTrapB Array>"
              # ">ForceTrapA Array>"
              # ">Extension Array>"
              n207 = Unbundle(w469) -> (w471:dbl[], w468:dbl[], w467:dbl[], w466:dbl[])
              n208 = Build Array (concatenate)(w471, w480) -> (w475:dbl[])
              n209 = Build Array (concatenate)(w468, w479) -> (w474:dbl[])
              n210 = Build Array (concatenate)(w467, w478) -> (w473:dbl[])
              n211 = Build Array (concatenate)(w466, w477) -> (w472:dbl[])
              n212 = Bundle(w475, w474, w473, w472) -> (w470:cluster{dbl[], dbl[], dbl[], dbl[]})  [unwired: 1 in]
            }
            frame True {
              w500 = dbl[] []
              w488 = 1000 ("chart length (points)")
              n213 = Unbundle(w505) -> (w504:dbl[], w503:dbl[], w502:dbl[], w501:dbl[])
              n214 = call-poly <vilib>:"Mean.vi"("X"=w501) -> ()  [unwired: 2 out]
              n215 = Select(t=1.0, s="Direction", f=-1.0) -> (s? t:f=w506:dbl)
              n216 = call <vilib>:"Std Deviation and Variance.vi"("X"=w504) -> ("mean"=w514:dbl, "standard deviation"=w518:dbl)  [unwired: 1 in, 1 out]
              n217 = call-poly <vilib>:"Mean.vi"("X"=w502) -> ("mean"=w523:dbl)  [unwired: 1 out]
              n218 = Select(t=1.0, s="IsPullActive?", f=0.0) -> (s? t:f=w507:dbl)
              n219 = call-poly <vilib>:"Mean.vi"("X"=w503) -> ("mean"=w522:dbl)  [unwired: 1 out]
              n220 = Multiply(x=w507, y=w506) -> (x*y=w516:dbl)
              n221 = property on="FEX Mirror Y Volt" class="DigNum (strict)"() -> ("Value"=w484:dbl)  [unwired: 2 in, 2 out]
              n222 = call-poly <vilib>:"DAQmx Create Virtual Channel.vi"("maximum value"=10.0 ("Maximum Value"), "minimum value"=0.0 ("Minimum Value"), "physical channels"=tag "PCI-6036E/ao0", "error in"=w493) -> ("task out"=w482:refnum<k21>, "error out"=w481:errorcluster)  [unwired: 10 in]
              n223 = Bundle("mean"=w514, "standard deviation"=w518) -> (w489:cluster{"mean":dbl, "standard deviation":dbl})  [unwired: 1 in]
              n224 = Bundle("mean"=w514, "mean"=w522) -> (w487:cluster{"mean":dbl, "mean":dbl})  [unwired: 1 in]
              n225 = Bundle("mean"=w514, "mean"=w523) -> ()  [unwired: 1 in, 1 out]
              n226 = Multiply(x="Mirror Step (V)", y=w516) -> (x*y=w515:dbl)
              n227 = call "XY Chart Buffer.vi"("clear first (no:F)"="Clear FEX Chart", "chart length (points)"=w488, "new point"=w489) -> ("XY chart data"=→"FEX Noise-Ext":cluster{"x":dbl, "y":dbl}[])  [unwired: 8 in]
              n228 = call "XY Chart Buffer.vi"("clear first (no:F)"="Clear FEX Chart", "chart length (points)"=w488, "new point"=w487) -> ("XY chart data"=→"FEX Force TrapA":cluster{"x":dbl, "y":dbl}[])  [unwired: 8 in]
              n229 = Add(x=w484, y=w515) -> (x+y=w521:dbl)
              n230 = In Range and Coerce(upper limit=10.0, x=w521, lower limit=0.0 ("upper limit")) -> (coerced(x)=w491:dbl)  [unwired: 1 out]
              n231 = call-poly <vilib>:"DAQmx Write.vi"("task/channels in"=w482, "data"=w491, "timeout"=10.0, "error in"=w481) -> ("task out"=w497:refnum<k21>, "error out"=w498:errorcluster)  [unwired: 9 in, 1 out]
              n232 = property on="FEX MirrorY Volt" class="DigNum (strict)"("Value"=w491) -> ()  [unwired: 2 in, 2 out]
              n233 = call <vilib>:"DAQmx Clear Task.vi"("task in"=w497, "error in"=w498) -> ("error out"=w492:errorcluster)  [unwired: 13 in]
              n234 = Bundle(w500, w500, w500, w500) -> (w499:cluster{dbl[], dbl[], dbl[], dbl[]})  [unwired: 1 in]
            }
          }
          n235 = property on="IsForceExtActive?" class="Bool (strict)"() -> ("Value"=w431:bool)  [unwired: 2 in, 2 out]
          n236 = Not(x=w431) -> (.not. x?=w430:bool)
        }
        n237 = call <vilib>:"Open_Create_Replace File.vi"("function (open:0)"=T19."create or replace", "file path"=w400) -> ("refnum"=w392:refnum<file>)  [unwired: 6 in, 3 out]
        n238 = while {
          tunnel: w389 -> [w426]
          tunnel: [w425] -> w381
          tunnel: w392 -> [w423]
          tunnel: [w422] -> w391
          tunnel: w365 -> [w419]
          tunnel: w406 -> [w418]
          shift-right: [w414] -> w378
          shift-left: w386 -> [w427]
          tunnel: [w413] -> w405
          stop <- w409 stop-if-true
          w424 = 10.0  # Timeout
          # "Enque Data"
          # "Force-Extension DAQ Loop"
          n239 = call-poly <vilib>:"DAQmx Read.vi"("task/channels in"=w426, "number of samples per channel"=w419, "timeout"=w424, "error in"=w427) -> ("task out"=w425:refnum<k21>, "data"=w420:dbl[][], "error out"=w417:errorcluster)  [unwired: 9 in]
          n240 = for {
            N: 8 -> [_]
            tunnel: [w429] -> w411 mode=indexing
            tunnel: w420 -> [w428] mode=indexing
            n241 = call-poly <vilib>:"Mean.vi"("X"=w428) -> ("mean"=w429:dbl)  [unwired: 1 out]
          }
          n242 = To Single Precision Float(number=w411) -> (single precision float=w412:sgl[])
          n243 = call <vilib>:"Write File+ [SGL].vi"("1D array"=w412, "error in (no error)"=w417, "refnum"=w423) -> ("error out"=w416:errorcluster, "dup refnum"=w422:refnum<file>)  [unwired: 6 in, 1 out]
          n244 = Enqueue Element(queue=w418, element=w411, error in (no error)=w417) -> (queue out=w413:refnum<queue>, error out=w415:errorcluster)  [unwired: 1 in, 1 out]
          n245 = property on="IsForceExtActive?" class="Bool (strict)"() -> ("Value"=w410:bool)  [unwired: 2 in, 2 out]
          n246 = Not(x=w410) -> (.not. x?=w409:bool)
          n247 = Merge Errors(w416, w415) -> (w414:errorcluster)
        }
        n248 = call <vilib>:"DAQmx Stop Task.vi"("task/channels in"=w381, "error in"=w378) -> ("task out"=w372:refnum<k21>, "error out"=w380:errorcluster)  [unwired: 12 in]
        n249 = Close File(refnum=w391) -> (error out=w377:errorcluster)  [unwired: 1 in, 1 out]
        n250 = Release Queue(queue=w405, error in (no error)=w380) -> (error out=w371:errorcluster)  [unwired: 1 in, 2 out]
        n251 = property on="InstrumentMode" class="Enum (strict)"(error in=w377, "Value"=w376) -> (error out=w385:errorcluster)  [unwired: 1 in, 1 out]
        n252 = property on="InterfaceSelector" class="TabCtl (strict)"(error in=w385, "Value"=T4."Basic Operation" ("InterfaceSelector")) -> (error out=w384:errorcluster)  [unwired: 1 in, 1 out]
        n253 = property on="IsForceExtActive?" class="Bool (strict)"(error in=w384, "Value"=FALSE ("IsOffsetModeActive?")) -> (error out=w368:errorcluster)  [unwired: 1 in, 1 out]
        n254 = property on="SampRate/Ch" class="DigNum (strict)"() -> ("Value"=w375:dbl)  [unwired: 2 in, 2 out]
        n255 = call "GetTrapSeparation(V).vi"("ErrorIn"=w371, "AcquisitionRatePerChannel"=w375, "DAQ Task"=w372) -> ("ErrorOut"=w369:errorcluster, "VertTrapSeparation(V)"=w373:dbl, "HorTrapSeparation(V)"=w374:dbl, "DAQ Task"=w370:refnum<k21>)  [unwired: 1 in]
        n256 = property on="BMSliderVert(V)" class="Slide (strict)"("Value"=w373) -> ()  [unwired: 2 in, 2 out]
        n257 = property on="BMHorizSlider(V)" class="Slide (strict)"("Value"=w374) -> ()  [unwired: 2 in, 2 out]
        n258 = Merge Errors(w368, w369, w367) -> (w366:errorcluster)
      }
      frame "Shutdown" {
        n259 = Wait (ms)(milliseconds to wait=u32 25) -> ()  [unwired: 1 out]
        n260 = call <vilib>:"DAQmx Clear Task.vi"("task in"=w524, "error in"=w527) -> ("error out"=w526:errorcluster)  [unwired: 13 in]
        n261 = property on="InstrumentMode" class="Enum (strict)"(error in=w526) -> (error out=w525:errorcluster, "Value"=w529:T1)  [unwired: 1 in, 1 out]
      }
    }
  }
  n262 = while {
    shift-right: [w536] -> w1
    shift-left: _ -> [w535]
    tunnel: w9 -> [w534]
    i -> [w532]
    stop <- w533 stop-if-true
    # "UI Loop"
    n263 = Wait (ms)(milliseconds to wait=u32 10) -> ()  [unwired: 1 out]
    n264 = event shown="[4] \"GoToTopDisp\": Value Change" {
      selector: _ -> [_ _ _ _ _ _ _ _ _ _ _ _ _ _ _ _]
      dyn-events: _ -> [_ _ _ _ _ _ _ _ _ _ _ _ _ _ _ _]
      timeout: 10 -> [_ _ _ _ _ _ _ _ _ _ _ _ _ _ _ _]
      tunnel: [_ w568 w597 w626 w665 w731 w797 w851 w861 w871 _ _ _ _ _ w923] -> w536
      tunnel: w535 -> [_ w567 w596 w625 w664 w730 w796 w854 w864 w871 _ _ _ _ _ w923]
      tunnel: [_ _ _ _ _ _ _ _ _ _ _ _ _ _ _ "Stop"] -> w533
      tunnel: w534 -> [_ w566 w595 w624 w663 w729 w795 _ _ _ _ _ _ _ _ _]
      tunnel: w532 -> [w539 _ _ _ _ _ _ _ _ _ _ _ _ _ _ _]
      event Timeout {
        n265 = event-data() -> ()  [unwired: 1 in, 1 out]
        n266 = case shown="True" "Oscillate Mirror?" {
          selector: "Oscillate Mirror?" -> [_ w554]
          tunnel: w539 -> [_ w555]
          frame False {
          }
          frame True {
            w564 = 100
            # "Enforce Upper/Lower Bounds"
            n267 = Multiply(x="Period (s)", y=1000) -> (x*y=w562:i32)
            n268 = Divide(x=6.283185307179586, y=w564) -> (x/y=w558:dbl)
            n269 = Divide(x=w562, y=w564) -> (x/y=w563:dbl)
            n270 = Multiply(x=w558, y=w555) -> (x*y=w559:dbl)
            n271 = Wait (ms)(milliseconds to wait=w563) -> ()  [unwired: 1 out]
            n272 = Sine(x=w559) -> (sin(x)=w560:dbl)
            n273 = Multiply(x="Amplitude (V)", y=w560) -> (x*y=w552:dbl)
            n274 = Add(x=w552, y="Offset (V)") -> (x+y=w540:dbl)
            "Mirror Voltage" <- w540
            n275 = property on="BMHorizSlider(V)" class="Slide (strict)"("Value"=w540) -> ()  [unwired: 2 in, 2 out]
            n276 = call-poly <vilib>:"DAQmx Create Virtual Channel.vi"("maximum value"=10.0 ("Maximum Value"), "minimum value"=0.0 ("Minimum Value"), "physical channels"=tag "PCI-6036E/ao0") -> ("task out"=w542:refnum<k21>, "error out"=w541:errorcluster)  [unwired: 11 in]
            n277 = In Range and Coerce(upper limit=10.0, x=w540, lower limit=0.0 ("upper limit")) -> (coerced(x)=w546:dbl)  [unwired: 1 out]
            n278 = call-poly <vilib>:"DAQmx Write.vi"("task/channels in"=w542, "data"=w546, "timeout"=10.0, "error in"=w541) -> ("task out"=w544:refnum<k21>, "error out"=w543:errorcluster)  [unwired: 9 in, 1 out]
            n279 = call <vilib>:"DAQmx Clear Task.vi"("task in"=w544, "error in"=w543) -> ()  [unwired: 13 in, 1 out]
            "Oscillate Mirror? 2" <- w554
          }
        }
      }
      event "SaveTopDisp": Value Change {
        n280 = event-data() -> ()  [unwired: 1 in, 1 out]
        n281 = property on="IsActive?" class="Bool (strict)"(error in=w567) -> (error out=w575:errorcluster, "Value"=w573:bool)  [unwired: 1 in, 1 out]
        n282 = property on="IsActive?" class="Bool (strict)"(error in=w575) -> (error out=w574:errorcluster, "Value"=w572:bool)  [unwired: 1 in, 1 out]
        n283 = property on="IsActive?" class="Bool (strict)"(error in=w574) -> (error out=w569:errorcluster, "Value"=w571:bool)  [unwired: 1 in, 1 out]
        n284 = Compound Arithmetic op=AND(w573, w572, w571) -> (w570:bool)
        n285 = case shown="True" w570 {
          tunnel: w569 -> [w576 w594]
          tunnel: [w576 w581] -> w568
          tunnel: w566 -> [_ w580]
          frame False {
          }
          frame True {
            # "Read the Current Motor Positions and save them to the Top Dispenser"
            # "X Motor Pos"
            # "Y Motor Pos"
            # "Z Motor Pos"
            n286 = Unbundle(w580) -> ("XMotorRef"=w577:refnum<k7>, "YMotorRef"=w578:refnum<k7>, "ZMotorRef"=w579:refnum<k7>)
            n287 = invoke class="MG17Motor" method="GetPosition_Position"(reference=w579, error in=w594, "lChanID"=0) -> (error out=w591:errorcluster, "GetPosition_Position"=w584:sgl)  [unwired: 1 in, 2 out]
            n288 = invoke class="MG17Motor" method="GetPosition_Position"(reference=w578, error in=w591, "lChanID"=0) -> (error out=w589:errorcluster, "GetPosition_Position"=w583:sgl)  [unwired: 1 in, 2 out]
            n289 = invoke class="MG17Motor" method="GetPosition_Position"(reference=w577, error in=w589, "lChanID"=0) -> (error out=w588:errorcluster, "GetPosition_Position"=w582:sgl)  [unwired: 1 in, 2 out]
            n290 = property on="Top Dispenser" class="Clust (strict)"(error in=w588) -> (error out=w587:errorcluster, "Value"=w586:T5)  [unwired: 1 in, 1 out]
            n291 = Bundle By Name(cluster=w586, "X Pos (mm)"=w582, "Y Pos (mm)"=w583, "Z Pos (mm)"=w584) -> (w585:T5)
            n292 = property on="Top Dispenser" class="Clust (strict)"(error in=w587, "Value"=w585) -> (error out=w581:errorcluster)  [unwired: 1 in, 1 out]
          }
        }
      }
      event "SaveBottDisp": Value Change {
        n293 = event-data() -> ()  [unwired: 1 in, 1 out]
        n294 = property on="IsActive?" class="Bool (strict)"(error in=w596) -> (error out=w604:errorcluster, "Value"=w602:bool)  [unwired: 1 in, 1 out]
        n295 = property on="IsActive?" class="Bool (strict)"(error in=w604) -> (error out=w603:errorcluster, "Value"=w601:bool)  [unwired: 1 in, 1 out]
        n296 = property on="IsActive?" class="Bool (strict)"(error in=w603) -> (error out=w598:errorcluster, "Value"=w600:bool)  [unwired: 1 in, 1 out]
        n297 = Compound Arithmetic op=AND(w602, w601, w600) -> (w599:bool)
        n298 = case shown="True" w599 {
          tunnel: w598 -> [w605 w623]
          tunnel: [w605 w610] -> w597
          tunnel: w595 -> [_ w609]
          frame False {
          }
          frame True {
            # "Read the Current Motor Positions and save them to the Bottom Dispenser"
            # "X Motor Pos"
            # "Y Motor Pos"
            # "Z Motor Pos"
            n299 = Unbundle(w609) -> ("XMotorRef"=w606:refnum<k7>, "YMotorRef"=w607:refnum<k7>, "ZMotorRef"=w608:refnum<k7>)
            n300 = invoke class="MG17Motor" method="GetPosition_Position"(reference=w608, error in=w623, "lChanID"=0) -> (error out=w620:errorcluster, "GetPosition_Position"=w613:sgl)  [unwired: 1 in, 2 out]
            n301 = invoke class="MG17Motor" method="GetPosition_Position"(reference=w607, error in=w620, "lChanID"=0) -> (error out=w618:errorcluster, "GetPosition_Position"=w612:sgl)  [unwired: 1 in, 2 out]
            n302 = invoke class="MG17Motor" method="GetPosition_Position"(reference=w606, error in=w618, "lChanID"=0) -> (error out=w617:errorcluster, "GetPosition_Position"=w611:sgl)  [unwired: 1 in, 2 out]
            n303 = property on="Bottom Dispenser" class="Clust (strict)"(error in=w617) -> (error out=w616:errorcluster, "Value"=w615:T5)  [unwired: 1 in, 1 out]
            n304 = Bundle By Name(cluster=w615, "X Pos (mm)"=w611, "Y Pos (mm)"=w612, "Z Pos (mm)"=w613) -> (w614:T5)
            n305 = property on="Bottom Dispenser" class="Clust (strict)"(error in=w616, "Value"=w614) -> (error out=w610:errorcluster)  [unwired: 1 in, 1 out]
          }
        }
      }
      event "SaveExpLoc": Value Change {
        n306 = event-data() -> ()  [unwired: 1 in, 1 out]
        n307 = property on="IsActive?" class="Bool (strict)"(error in=w625) -> (error out=w633:errorcluster, "Value"=w631:bool)  [unwired: 1 in, 1 out]
        n308 = property on="IsActive?" class="Bool (strict)"(error in=w633) -> (error out=w632:errorcluster, "Value"=w630:bool)  [unwired: 1 in, 1 out]
        n309 = property on="IsActive?" class="Bool (strict)"(error in=w632) -> (error out=w627:errorcluster, "Value"=w629:bool)  [unwired: 1 in, 1 out]
        n310 = Compound Arithmetic op=AND(w631, w630, w629) -> (w628:bool)
        n311 = case shown="True" w628 {
          tunnel: w627 -> [w634 w652]
          tunnel: [w634 w639] -> w626
          tunnel: w624 -> [_ w638]
          frame False {
          }
          frame True {
            # "Read the Current Motor Positions and save them to the Exp Location"
            # "X Motor Pos"
            # "Y Motor Pos"
            # "Z Motor Pos"
            n312 = Unbundle(w638) -> ("XMotorRef"=w635:refnum<k7>, "YMotorRef"=w636:refnum<k7>, "ZMotorRef"=w637:refnum<k7>)
            n313 = invoke class="MG17Motor" method="GetPosition_Position"(reference=w637, error in=w652, "lChanID"=0) -> (error out=w649:errorcluster, "GetPosition_Position"=w642:sgl)  [unwired: 1 in, 2 out]
            n314 = invoke class="MG17Motor" method="GetPosition_Position"(reference=w636, error in=w649, "lChanID"=0) -> (error out=w647:errorcluster, "GetPosition_Position"=w641:sgl)  [unwired: 1 in, 2 out]
            n315 = invoke class="MG17Motor" method="GetPosition_Position"(reference=w635, error in=w647, "lChanID"=0) -> (error out=w646:errorcluster, "GetPosition_Position"=w640:sgl)  [unwired: 1 in, 2 out]
            n316 = property on="Experiment Region" class="Clust (strict)"(error in=w646) -> (error out=w645:errorcluster, "Value"=w644:T5)  [unwired: 1 in, 1 out]
            n317 = Bundle By Name(cluster=w644, "X Pos (mm)"=w640, "Y Pos (mm)"=w641, "Z Pos (mm)"=w642) -> (w643:T5)
            n318 = property on="Experiment Region" class="Clust (strict)"(error in=w645, "Value"=w643) -> (error out=w639:errorcluster)  [unwired: 1 in, 1 out]
          }
        }
      }
      event "GoToTopDisp": Value Change {
        n319 = event-data() -> ()  [unwired: 1 in, 1 out]
        n320 = property on="IsActive?" class="Bool (strict)"(error in=w664) -> (error out=w672:errorcluster, "Value"=w670:bool)  [unwired: 1 in, 1 out]
        n321 = property on="Motor Cruise Param" class="Clust (strict)"() -> ("Value"=w653:T11)  [unwired: 2 in, 2 out]
        n322 = Unbundle By Name(w653) -> ("X Acc (mm/s^2)"=w657:sgl, "X Vmax (mm/s)"=w656:sgl, "Y Acc (mm/s^2)"=w655:sgl, "Y Vmax (mm/s)"=w654:sgl, "Z Acc (mm/s^2)"=w659:sgl, "Z Vmax (mm/s)"=w658:sgl)
        n323 = property on="IsActive?" class="Bool (strict)"(error in=w672) -> (error out=w671:errorcluster, "Value"=w669:bool)  [unwired: 1 in, 1 out]
        n324 = property on="IsActive?" class="Bool (strict)"(error in=w671) -> (error out=w666:errorcluster, "Value"=w668:bool)  [unwired: 1 in, 1 out]
        n325 = Unbundle(w663) -> ("XMotorRef"=w662:refnum<k7>, "YMotorRef"=w661:refnum<k7>, "ZMotorRef"=w660:refnum<k7>)
        n326 = Compound Arithmetic op=AND(w670, w669, w668) -> (w667:bool)
        n327 = case shown="True" w667 {
          tunnel: w666 -> [w673 w693]
          tunnel: [w673 w689] -> w665
          tunnel: w662 -> [_ w716]
          tunnel: w661 -> [_ w701]
          tunnel: w660 -> [_ w688]
          tunnel: w659 -> [_ w679]
          tunnel: w658 -> [_ w678]
          tunnel: w657 -> [_ w677]
          tunnel: w656 -> [_ w676]
          tunnel: w655 -> [_ w675]
          tunnel: w654 -> [_ w674]
          frame False {
          }
          frame True {
            (unwired) 0 ("lChanID")
            n328 = invoke class="MG17Motor" method="StopImmediate"(reference=w716, error in=w693, "lChanID"=0) -> (reference out=w714:refnum<k7>, error out=w715:errorcluster, "lChanID"=w684:i32)  [unwired: 1 in, 1 out]
            n329 = invoke class="MG17Motor" method="StopImmediate"(reference=w701, error in=w693, "lChanID"=0) -> (reference out=w708:refnum<k7>, error out=w709:errorcluster, "lChanID"=w685:i32)  [unwired: 1 in, 1 out]
            n330 = invoke class="MG17Motor" method="StopImmediate"(reference=w688, error in=w693, "lChanID"=0) -> (reference out=w698:refnum<k7>, error out=w699:errorcluster, "lChanID"=w686:i32)  [unwired: 1 in, 1 out]
            n331 = property on="Top Dispenser" class="Clust (strict)"(error in=w693) -> ("Value"=w718:T5)  [unwired: 1 in, 2 out]
            n332 = invoke class="MG17Motor" method="SetVelParams"(reference=w698, error in=w699, "lChanID"=w686, "fMinVel"=sgl 0.0, "fAccn"=w679, "fMaxVel"=w678) -> (reference out=w697:refnum<k7>, error out=w696:errorcluster, "lChanID"=w695:i32)  [unwired: 1 in, 4 out]
            n333 = invoke class="MG17Motor" method="SetVelParams"(reference=w714, error in=w715, "lChanID"=w684, "fMinVel"=sgl 0.0, "fAccn"=w677, "fMaxVel"=w676) -> (reference out=w713:refnum<k7>, error out=w712:errorcluster, "lChanID"=w711:i32)  [unwired: 1 in, 4 out]
            n334 = invoke class="MG17Motor" method="SetVelParams"(reference=w708, error in=w709, "lChanID"=w685, "fMinVel"=sgl 0.0, "fAccn"=w675, "fMaxVel"=w674) -> (reference out=w706:refnum<k7>, error out=w705:errorcluster, "lChanID"=w704:i32)  [unwired: 1 in, 4 out]
            n335 = Unbundle By Name(w718) -> ("X Pos (mm)"=w682:sgl, "Y Pos (mm)"=w681:sgl, "Z Pos (mm)"=w680:sgl)
            n336 = invoke class="MG17Motor" method="MoveAbsoluteEx"(reference=w713, error in=w712, "lChanID"=w711, "fAbsPosCh1"=w682, "fAbsPosCh2"=w682, "bWait"=FALSE) -> (error out=w692:errorcluster)  [unwired: 1 in, 6 out]
            n337 = invoke class="MG17Motor" method="MoveAbsoluteEx"(reference=w706, error in=w705, "lChanID"=w704, "fAbsPosCh1"=w681, "fAbsPosCh2"=w681, "bWait"=FALSE) -> (error out=w691:errorcluster)  [unwired: 1 in, 6 out]
            n338 = invoke class="MG17Motor" method="MoveAbsoluteEx"(reference=w697, error in=w696, "lChanID"=w695, "fAbsPosCh1"=w680, "fAbsPosCh2"=w680, "bWait"=FALSE) -> (error out=w690:errorcluster)  [unwired: 1 in, 6 out]
            n339 = Merge Errors(w692, w691, w690) -> (w689:errorcluster)
          }
        }
      }
      event "GoToBottDisp": Value Change {
        n340 = event-data() -> ()  [unwired: 1 in, 1 out]
        n341 = property on="IsActive?" class="Bool (strict)"(error in=w730) -> (error out=w738:errorcluster, "Value"=w736:bool)  [unwired: 1 in, 1 out]
        n342 = property on="Motor Cruise Param" class="Clust (strict)"() -> ("Value"=w725:T11)  [unwired: 2 in, 2 out]
        n343 = Unbundle By Name(w725) -> ("X Acc (mm/s^2)"=w724:sgl, "X Vmax (mm/s)"=w723:sgl, "Y Acc (mm/s^2)"=w722:sgl, "Y Vmax (mm/s)"=w721:sgl, "Z Acc (mm/s^2)"=w720:sgl, "Z Vmax (mm/s)"=w719:sgl)
        n344 = property on="IsActive?" class="Bool (strict)"(error in=w738) -> (error out=w737:errorcluster, "Value"=w735:bool)  [unwired: 1 in, 1 out]
        n345 = property on="IsActive?" class="Bool (strict)"(error in=w737) -> (error out=w732:errorcluster, "Value"=w734:bool)  [unwired: 1 in, 1 out]
        n346 = Unbundle(w729) -> ("XMotorRef"=w728:refnum<k7>, "YMotorRef"=w727:refnum<k7>, "ZMotorRef"=w726:refnum<k7>)
        n347 = Compound Arithmetic op=AND(w736, w735, w734) -> (w733:bool)
        n348 = case shown="True" w733 {
          tunnel: w732 -> [w739 w759]
          tunnel: [w739 w755] -> w731
          tunnel: w728 -> [_ w782]
          tunnel: w727 -> [_ w767]
          tunnel: w726 -> [_ w754]
          tunnel: w724 -> [_ w745]
          tunnel: w723 -> [_ w744]
          tunnel: w722 -> [_ w743]
          tunnel: w721 -> [_ w742]
          tunnel: w720 -> [_ w741]
          tunnel: w719 -> [_ w740]
          frame False {
          }
          frame True {
            (unwired) 0 ("lChanID")
            n349 = invoke class="MG17Motor" method="StopImmediate"(reference=w782, error in=w759, "lChanID"=0) -> (reference out=w780:refnum<k7>, error out=w781:errorcluster, "lChanID"=w750:i32)  [unwired: 1 in, 1 out]
            n350 = invoke class="MG17Motor" method="StopImmediate"(reference=w767, error in=w759, "lChanID"=0) -> (reference out=w774:refnum<k7>, error out=w775:errorcluster, "lChanID"=w751:i32)  [unwired: 1 in, 1 out]
            n351 = invoke class="MG17Motor" method="StopImmediate"(reference=w754, error in=w759, "lChanID"=0) -> (reference out=w764:refnum<k7>, error out=w765:errorcluster, "lChanID"=w752:i32)  [unwired: 1 in, 1 out]
            n352 = property on="Bottom Dispenser" class="Clust (strict)"(error in=w759) -> ("Value"=w784:T5)  [unwired: 1 in, 2 out]
            n353 = invoke class="MG17Motor" method="SetVelParams"(reference=w780, error in=w781, "lChanID"=w750, "fMinVel"=sgl 0.0, "fAccn"=w745, "fMaxVel"=w744) -> (reference out=w779:refnum<k7>, error out=w778:errorcluster, "lChanID"=w777:i32)  [unwired: 1 in, 4 out]
            n354 = invoke class="MG17Motor" method="SetVelParams"(reference=w764, error in=w765, "lChanID"=w752, "fMinVel"=sgl 0.0, "fAccn"=w741, "fMaxVel"=w740) -> (reference out=w763:refnum<k7>, error out=w762:errorcluster, "lChanID"=w761:i32)  [unwired: 1 in, 4 out]
            n355 = invoke class="MG17Motor" method="SetVelParams"(reference=w774, error in=w775, "lChanID"=w751, "fMinVel"=sgl 0.0, "fAccn"=w743, "fMaxVel"=w742) -> (reference out=w772:refnum<k7>, error out=w771:errorcluster, "lChanID"=w770:i32)  [unwired: 1 in, 4 out]
            n356 = Unbundle By Name(w784) -> ("X Pos (mm)"=w748:sgl, "Y Pos (mm)"=w747:sgl, "Z Pos (mm)"=w746:sgl)
            n357 = invoke class="MG17Motor" method="MoveAbsoluteEx"(reference=w779, error in=w778, "lChanID"=w777, "fAbsPosCh1"=w748, "fAbsPosCh2"=w748, "bWait"=FALSE) -> (error out=w758:errorcluster)  [unwired: 1 in, 6 out]
            n358 = invoke class="MG17Motor" method="MoveAbsoluteEx"(reference=w772, error in=w771, "lChanID"=w770, "fAbsPosCh1"=w747, "fAbsPosCh2"=w747, "bWait"=FALSE) -> (error out=w757:errorcluster)  [unwired: 1 in, 6 out]
            n359 = invoke class="MG17Motor" method="MoveAbsoluteEx"(reference=w763, error in=w762, "lChanID"=w761, "fAbsPosCh1"=w746, "fAbsPosCh2"=w746, "bWait"=FALSE) -> (error out=w756:errorcluster)  [unwired: 1 in, 6 out]
            n360 = Merge Errors(w758, w757, w756) -> (w755:errorcluster)
          }
        }
      }
      event "GoToExpLoc": Value Change {
        n361 = event-data() -> ()  [unwired: 1 in, 1 out]
        n362 = property on="Motor Cruise Param" class="Clust (strict)"() -> ("Value"=w791:T11)  [unwired: 2 in, 2 out]
        n363 = property on="IsActive?" class="Bool (strict)"(error in=w796) -> (error out=w804:errorcluster, "Value"=w802:bool)  [unwired: 1 in, 1 out]
        n364 = Unbundle By Name(w791) -> ("X Acc (mm/s^2)"=w790:sgl, "X Vmax (mm/s)"=w789:sgl, "Y Acc (mm/s^2)"=w788:sgl, "Y Vmax (mm/s)"=w787:sgl, "Z Acc (mm/s^2)"=w786:sgl, "Z Vmax (mm/s)"=w785:sgl)
        n365 = property on="IsActive?" class="Bool (strict)"(error in=w804) -> (error out=w803:errorcluster, "Value"=w801:bool)  [unwired: 1 in, 1 out]
        n366 = property on="IsActive?" class="Bool (strict)"(error in=w803) -> (error out=w798:errorcluster, "Value"=w800:bool)  [unwired: 1 in, 1 out]
        n367 = Unbundle(w795) -> ("XMotorRef"=w794:refnum<k7>, "YMotorRef"=w793:refnum<k7>, "ZMotorRef"=w792:refnum<k7>)
        n368 = Compound Arithmetic op=AND(w802, w801, w800) -> (w799:bool)
        n369 = case shown="True" w799 {
          tunnel: w798 -> [w805 w825]
          tunnel: [w805 w821] -> w797
          tunnel: w794 -> [_ w848]
          tunnel: w793 -> [_ w833]
          tunnel: w792 -> [_ w820]
          tunnel: w790 -> [_ w811]
          tunnel: w789 -> [_ w810]
          tunnel: w788 -> [_ w809]
          tunnel: w787 -> [_ w808]
          tunnel: w786 -> [_ w807]
          tunnel: w785 -> [_ w806]
          frame False {
          }
          frame True {
            (unwired) 0 ("lChanID")
            n370 = invoke class="MG17Motor" method="StopImmediate"(reference=w848, error in=w825, "lChanID"=0) -> (reference out=w846:refnum<k7>, error out=w847:errorcluster, "lChanID"=w816:i32)  [unwired: 1 in, 1 out]
            n371 = invoke class="MG17Motor" method="StopImmediate"(reference=w833, error in=w825, "lChanID"=0) -> (reference out=w840:refnum<k7>, error out=w841:errorcluster, "lChanID"=w817:i32)  [unwired: 1 in, 1 out]
            n372 = invoke class="MG17Motor" method="StopImmediate"(reference=w820, error in=w825, "lChanID"=0) -> (reference out=w830:refnum<k7>, error out=w831:errorcluster, "lChanID"=w818:i32)  [unwired: 1 in, 1 out]
            n373 = property on="Experiment Region" class="Clust (strict)"(error in=w825) -> ("Value"=w850:T5)  [unwired: 1 in, 2 out]
            n374 = invoke class="MG17Motor" method="SetVelParams"(reference=w846, error in=w847, "lChanID"=w816, "fMinVel"=sgl 0.0, "fAccn"=w811, "fMaxVel"=w810) -> (reference out=w845:refnum<k7>, error out=w844:errorcluster, "lChanID"=w843:i32)  [unwired: 1 in, 4 out]
            n375 = invoke class="MG17Motor" method="SetVelParams"(reference=w830, error in=w831, "lChanID"=w818, "fMinVel"=sgl 0.0, "fAccn"=w807, "fMaxVel"=w806) -> (reference out=w829:refnum<k7>, error out=w828:errorcluster, "lChanID"=w827:i32)  [unwired: 1 in, 4 out]
            n376 = invoke class="MG17Motor" method="SetVelParams"(reference=w840, error in=w841, "lChanID"=w817, "fMinVel"=sgl 0.0, "fAccn"=w809, "fMaxVel"=w808) -> (reference out=w838:refnum<k7>, error out=w837:errorcluster, "lChanID"=w836:i32)  [unwired: 1 in, 4 out]
            n377 = Unbundle By Name(w850) -> ("X Pos (mm)"=w814:sgl, "Y Pos (mm)"=w813:sgl, "Z Pos (mm)"=w812:sgl)
            n378 = invoke class="MG17Motor" method="MoveAbsoluteEx"(reference=w845, error in=w844, "lChanID"=w843, "fAbsPosCh1"=w814, "fAbsPosCh2"=w814, "bWait"=FALSE) -> (error out=w824:errorcluster)  [unwired: 1 in, 6 out]
            n379 = invoke class="MG17Motor" method="MoveAbsoluteEx"(reference=w838, error in=w837, "lChanID"=w836, "fAbsPosCh1"=w813, "fAbsPosCh2"=w813, "bWait"=FALSE) -> (error out=w823:errorcluster)  [unwired: 1 in, 6 out]
            n380 = invoke class="MG17Motor" method="MoveAbsoluteEx"(reference=w829, error in=w828, "lChanID"=w827, "fAbsPosCh1"=w812, "fAbsPosCh2"=w812, "bWait"=FALSE) -> (error out=w822:errorcluster)  [unwired: 1 in, 6 out]
            n381 = Merge Errors(w824, w823, w822) -> (w821:errorcluster)
          }
        }
      }
      event "Steerable \nTrap\n(F12)": Value Change {
        # "Update the TTL signal to the shutter"
        n382 = event-data() -> ("NewVal"=w856:bool)  [unwired: 1 in]
        n383 = call-poly <vilib>:"DAQmx Create Virtual Channel.vi"("lines"=tag "PCI-6036E/port0/line0", "name to assign"="TrapA_TTL_Signal", "error in"=w854) -> ("task out"=w858:refnum<k21>, "error out"=w855:errorcluster)  [unwired: 11 in]
        n384 = call-poly <vilib>:"DAQmx Write.vi"("task/channels in"=w858, "data"=w856, "timeout"=10.0, "error in"=w855) -> ("task out"=w853:refnum<k21>, "error out"=w852:errorcluster)  [unwired: 9 in, 1 out]
        n385 = call <vilib>:"DAQmx Clear Task.vi"("task in"=w853, "error in"=w852) -> ("error out"=w851:errorcluster)  [unwired: 13 in]
      }
      event "Fixed\nTrap\n(F11)": Value Change {
        # "Update the TTL signal to the shutter"
        n386 = event-data() -> ("NewVal"=w866:bool)  [unwired: 1 in]
        n387 = call-poly <vilib>:"DAQmx Create Virtual Channel.vi"("lines"=tag "PCI-6036E/port0/line1", "name to assign"="TrapB_TTL_Signal", "error in"=w864) -> ("task out"=w868:refnum<k21>, "error out"=w865:errorcluster)  [unwired: 11 in]
        n388 = call-poly <vilib>:"DAQmx Write.vi"("task/channels in"=w868, "data"=w866, "timeout"=10.0, "error in"=w865) -> ("task out"=w863:refnum<k21>, "error out"=w862:errorcluster)  [unwired: 9 in, 1 out]
        n389 = call <vilib>:"DAQmx Clear Task.vi"("task in"=w863, "error in"=w862) -> ("error out"=w861:errorcluster)  [unwired: 13 in]
      }
      event "InterfaceSelector": Value Change {
        n390 = event-data() -> ("NewVal"=w873:T4)  [unwired: 1 in]
        n391 = case shown="\"Force-Extension (F4)\"" w873 {
          tunnel: [T1."BasicMode" T1."PassiveMode" T1."AcquireOffsetMode" T1."AcquireSpectrumMode" T1."Force-ExtensionMode"] -> w872
          frame "Basic Operation" {
          }
          frame "Passive Mode (F1)" {
            n392 = property on="IsPassiveModeActive?" class="Bool (strict)"("Value"=TRUE ("StopOffset")) -> ()  [unwired: 2 in, 2 out]
          }
          frame "Acquire Offset (F2)" {
            n393 = property on="IsOffsetModeActive?" class="Bool (strict)"("Value"=TRUE ("StopOffset")) -> ()  [unwired: 2 in, 2 out]
          }
          frame "Acquire Spectrum (F3)" {
          }
          frame "Force-Extension (F4)" {
            n394 = property on="IsForceExtActive?" class="Bool (strict)"("Value"=TRUE ("StopOffset")) -> ()  [unwired: 2 in, 2 out]
          }
        }
        "InstrumentMode" <- w872
      }
      event "BMSliderVert(V)": Value Change {
        # "Enforce Upper/Lower Limit for the axis voltage"
        # "X axis on the MadCityLabs controller, vertical bead motion"
        n395 = event-data() -> ()  [unwired: 1 in, 6 out]
        n396 = call-poly <vilib>:"DAQmx Create Virtual Channel.vi"("maximum value"=10.0 ("Maximum Value"), "minimum value"=0.0 ("Minimum Value"), "physical channels"=tag "PCI-6036E/ao1") -> ("task out"=w883:refnum<k21>, "error out"=w882:errorcluster)  [unwired: 11 in]
        n397 = In Range and Coerce(upper limit=10.0, x="BMSliderVert(V)", lower limit=0.0 ("upper limit")) -> (coerced(x)=w888:dbl)  [unwired: 1 out]
        n398 = call-poly <vilib>:"DAQmx Write.vi"("task/channels in"=w883, "data"=w888, "timeout"=10.0, "error in"=w882) -> ("task out"=w885:refnum<k21>, "error out"=w884:errorcluster)  [unwired: 9 in, 1 out]
        n399 = call <vilib>:"DAQmx Clear Task.vi"("task in"=w885, "error in"=w884) -> ()  [unwired: 13 in, 1 out]
      }
      event "BMHorizSlider(V)": Value Change {
        # "Enforce Upper/Lower Bounds"
        # "Y axis on the MadCityLabs controller corresponds to horizontall bead motion"
        n400 = event-data() -> ()  [unwired: 1 in, 6 out]
        n401 = call-poly <vilib>:"DAQmx Create Virtual Channel.vi"("maximum value"=10.0 ("Maximum Value"), "minimum value"=0.0 ("Minimum Value"), "physical channels"=tag "PCI-6036E/ao0") -> ("task out"=w896:refnum<k21>, "error out"=w895:errorcluster)  [unwired: 11 in]
        n402 = In Range and Coerce(upper limit=10.0, x="BMHorizSlider(V)", lower limit=0.0 ("upper limit")) -> (coerced(x)=w900:dbl)  [unwired: 1 out]
        n403 = call-poly <vilib>:"DAQmx Write.vi"("task/channels in"=w896, "data"=w900, "timeout"=10.0, "error in"=w895) -> ("task out"=w898:refnum<k21>, "error out"=w897:errorcluster)  [unwired: 9 in, 1 out]
        n404 = call <vilib>:"DAQmx Clear Task.vi"("task in"=w898, "error in"=w897) -> ()  [unwired: 13 in, 1 out]
      }
      event "StopOffset": Value Change {
        n405 = event-data() -> ("NewVal"=w906:bool)  [unwired: 1 in, 5 out]
        n406 = case shown="True" w906 {
          frame False {
          }
          frame True {
            n407 = flat-sequence {
              frame #0 {
                n408 = Not(x="StopOffset") -> (.not. x?=→"IsOffsetModeActive?":bool)
              }
              frame #1 {
                n409 = property on="InterfaceSelector" class="TabCtl (strict)"("Value"=T4."Basic Operation" ("InterfaceSelector")) -> ()  [unwired: 2 in, 2 out]
                n410 = property on="InstrumentMode" class="Enum (strict)"("Value"=T1."BasicMode" ("InstrumentMode")) -> ()  [unwired: 2 in, 2 out]
              }
            }
          }
        }
      }
      event "StopPassiveMode": Value Change {
        n411 = event-data() -> ("NewVal"=w911:bool)  [unwired: 1 in, 5 out]
        n412 = case shown="True" w911 {
          frame False {
          }
          frame True {
            n413 = flat-sequence {
              frame #0 {
                n414 = Not(x="StopPassiveMode") -> (.not. x?=→"IsPassiveModeActive?":bool)
              }
              frame #1 {
                n415 = property on="InterfaceSelector" class="TabCtl (strict)"("Value"=T4."Basic Operation" ("InterfaceSelector")) -> ()  [unwired: 2 in, 2 out]
                n416 = property on="InstrumentMode" class="Enum (strict)"("Value"=T1."BasicMode" ("InstrumentMode")) -> ()  [unwired: 2 in, 2 out]
              }
            }
          }
        }
      }
      event "StopForceExtension": Value Change {
        n417 = event-data() -> ("NewVal"=w916:bool)  [unwired: 1 in, 5 out]
        n418 = case shown="True" w916 {
          frame False {
          }
          frame True {
            n419 = flat-sequence {
              frame #0 {
                n420 = Not(x="StopForceExtension") -> (.not. x?=→"IsForceExtActive?":bool)
              }
              frame #1 {
                n421 = property on="InterfaceSelector" class="TabCtl (strict)"("Value"=T4."Basic Operation" ("InterfaceSelector")) -> ()  [unwired: 2 in, 2 out]
                n422 = property on="InstrumentMode" class="Enum (strict)"("Value"=T1."BasicMode" ("InstrumentMode")) -> ()  [unwired: 2 in, 2 out]
              }
            }
          }
        }
      }
      event "Stop": Value Change {
        n423 = event-data() -> ()  [unwired: 1 in, 1 out]
        n424 = property on="InstrumentMode" class="Enum (strict)"("Value"=T1."Shutdown") -> ()  [unwired: 2 in, 2 out]
      }
    }
  }
  n425 = while {
    shift-right: [w925] -> _
    shift-left: T1."InitializeJoystick" -> [w924]
    shift-right: [w942] -> _
    shift-left: _ -> [w935]
    shift-right: [w939] -> w5
    shift-left: _ -> [w941]
    shift-right: [w940] -> _
    shift-left: _ -> [w938]
    shift-right: [w937] -> _
    shift-left: _ -> [w936]
    shift-right: [w934] -> _
    shift-left: _ -> [w931]
    shift-right: [w932] -> _
    shift-left: _ -> [w933]
    stop <- w926 stop-if-true
    # "Motor Control Loop"
    # ">Joystick Offset>"
    # ">RelJoyPos>"
    # ">XYZ Motor Ref>"
    # ">Error>"
    # ">Joystick Task ID>"
    # ">Joystick Buttons>"
    n426 = control-ref of="Steerable \nTrap\n(F12)"() -> (w928:refnum<vi>)
    n427 = control-ref of="Fixed\nTrap\n(F11)"() -> (w929:refnum<vi>)
    n428 = Bundle("Steerable \nTrap\n(F12)"=w928, "Fixed\nTrap\n(F11)"=w929) -> (w927:T24)  [unwired: 1 in]
    n429 = Wait (ms)(milliseconds to wait="MotorLoopDelay") -> ()  [unwired: 1 out]
    n430 = case shown="\"InitializeJoystick\"" w924 {
      tunnel: [w971 _ w1059 w1149 w1156 w1163 w1170 _] -> w942
      tunnel: [T1."InitializeMotors" w975 w1043 w1153 w1160 w1167 w1174 w1193] -> w925
      tunnel: w941 -> [_ w1024 w1061 w1152 w1159 w1166 w1173 w1178]
      tunnel: [w970 _ w1060 w1147 w1154 w1161 w1168 _] -> w940
      tunnel: [w946 w1023 w1052 w1152 w1159 w1166 w1173 w1175] -> w939
      tunnel: w938 -> [_ _ w1062 w1147 w1154 w1161 w1168 w1177]
      tunnel: [_ _ w1046 w1148 w1155 w1162 w1169 _] -> w937
      tunnel: w936 -> [_ _ w1045 w1148 w1155 w1162 w1169 _]
      tunnel: w935 -> [_ _ w1057 w1149 w1156 w1163 w1170 _]
      tunnel: [_ _ _ _ _ _ _ TRUE ("status")] -> w926
      tunnel: [_ w1022 w1051 w1151 w1158 w1165 w1172 _] -> w934
      tunnel: w931 -> [_ _ w1051 w1151 w1158 w1165 w1172 w1179]
      tunnel: [_ _ w1049 w1150 w1157 w1164 w1171 _] -> w932
      tunnel: w933 -> [_ _ w1058 w1150 w1157 w1164 w1171 _]
      tunnel: w927 -> [w961 _ w1044 _ _ _ _ _]
      frame "InitializeJoystick" {
        # "Initialize Joystick and Shutter Controls"
        n431 = property on="JoystOffset" class="Clust (strict)"() -> ("Value"=w969:T2)  [unwired: 2 in, 2 out]
        n432 = Bundle By Name(cluster=w969, "XOffset"=-99999, "YOffset"=-99999, "ZOffset"=-99999) -> (w971:T2)
        n433 = Unbundle(w961) -> ("Steerable \nTrap\n(F12)"=w950:refnum<vi>, "Fixed\nTrap\n(F11)"=w949:refnum<vi>)
        n434 = call <vilib>:"Initialize Joystick.vi"() -> ("error out"=w951:errorcluster, "device ID"=w970:refnum<k1>)  [unwired: 10 in]
        n435 = call-poly <vilib>:"DAQmx Create Virtual Channel.vi"("lines"=tag "PCI-6036E/port0/line1", "name to assign"="TrapB_TTL_Signal", "error in"=w951) -> ("task out"=w957:refnum<k21>, "error out"=w959:errorcluster)  [unwired: 11 in]
        n436 = call-poly <vilib>:"DAQmx Create Virtual Channel.vi"("lines"=tag "PCI-6036E/port0/line0", "name to assign"="TrapA_TTL_Signal", "error in"=w951) -> ("task out"=w966:refnum<k21>, "error out"=w968:errorcluster)  [unwired: 11 in]
        n437 = call-poly <vilib>:"DAQmx Read.vi"("task/channels in"=w957, "timeout"=10.0, "error in"=w959) -> ("task out"=w953:refnum<k21>, "data"=w944:bool, "error out"=w954:errorcluster)  [unwired: 10 in]
        n438 = call-poly <vilib>:"DAQmx Read.vi"("task/channels in"=w966, "timeout"=10.0, "error in"=w968) -> ("task out"=w962:refnum<k21>, "data"=w945:bool, "error out"=w963:errorcluster)  [unwired: 10 in]
        n439 = property class="Bool (strict)"(reference=w950, error in=w963, "Value"=w945) -> (error out=w960:errorcluster)  [unwired: 1 out]
        n440 = property class="Bool (strict)"(reference=w949, error in=w954, "Value"=w944) -> (error out=w952:errorcluster)  [unwired: 1 out]
        n441 = call <vilib>:"DAQmx Clear Task.vi"("task in"=w953, "error in"=w952) -> ("error out"=w947:errorcluster)  [unwired: 13 in]
        n442 = call <vilib>:"DAQmx Clear Task.vi"("task in"=w962, "error in"=w960) -> ("error out"=w948:errorcluster)  [unwired: 13 in]
        n443 = Merge Errors(w948, w947) -> (w946:errorcluster)
      }
      frame "InitializeMotors" {
        w975 = T1."BasicMode"
        w1028 = 83829794  # Z Axis Controller ID
        w1034 = 83829822  # Y Axis Controller ID
        w1040 = 83829798  # X Axis Controller ID
        n444 = property on="IsActive?" class="Bool (strict)"(error in=w1024, "Value"=FALSE ("IsYMotorActive?")) -> (error out=w1035:errorcluster)  [unwired: 1 in, 1 out]
        n445 = property on="IsActive?" class="Bool (strict)"(error in=w1024, "Value"=FALSE ("IsYMotorActive?")) -> (error out=w1041:errorcluster)  [unwired: 1 in, 1 out]
        n446 = property on="IsActive?" class="Bool (strict)"(error in=w1024, "Value"=FALSE ("IsYMotorActive?")) -> (error out=w1029:errorcluster)  [unwired: 1 in, 1 out]
        n447 = call "s_InitializeMotor.vi"("Error In"=w1035, "Servo Controller  ID"=w1034, "Motor Reference In"="YMotorRef") -> ("Error Out"=w1036:errorcluster, "Motor Reference"=w1017:refnum<k7>)
        n448 = call "s_InitializeMotor.vi"("Error In"=w1041, "Servo Controller  ID"=w1040, "Motor Reference In"="XMotorRef") -> ("Error Out"=w1042:errorcluster, "Motor Reference"=w1021:refnum<k7>)
        n449 = call "s_InitializeMotor.vi"("Error In"=w1029, "Servo Controller  ID"=w1028, "Motor Reference In"="ZMotorRef") -> ("Error Out"=w1030:errorcluster, "Motor Reference"=w1014:refnum<k7>)
        n450 = property on="IsActive?" class="Bool (strict)"(error in=w1036, "Value"=TRUE ("IsYMotorActive?")) -> (error out=w1016:errorcluster)  [unwired: 1 in, 1 out]
        n451 = Unbundle By Name("Motor Limits") -> ("XMin"=w981:sgl, "XMax"=w980:sgl, "YMin"=w979:sgl, "YMax"=w978:sgl, "ZMin"=w977:sgl, "ZMax"=w976:sgl)
        n452 = property on="IsActive?" class="Bool (strict)"(error in=w1042, "Value"=TRUE ("IsYMotorActive?")) -> (error out=w1019:errorcluster)  [unwired: 1 in, 1 out]
        n453 = property on="IsActive?" class="Bool (strict)"(error in=w1030, "Value"=TRUE ("IsYMotorActive?")) -> (error out=w1013:errorcluster)  [unwired: 1 in, 1 out]
        n454 = invoke class="MG17Motor" method="SetStageAxisInfo"(reference=w1021, error in=w1019, "lChanID"=0, "fMinPos"=w981, "fMaxPos"=w980, "lUnits"=1, "fPitch"=sgl 1.0, "lDirSense"=0) -> (reference out=w1012:refnum<k7>, error out=w1011:errorcluster, "lChanID"=w1010:i32)  [unwired: 1 in, 6 out]
        n455 = invoke class="MG17Motor" method="SetStageAxisInfo"(reference=w1017, error in=w1016, "lChanID"=0, "fMinPos"=w979, "fMaxPos"=w978, "lUnits"=1, "fPitch"=sgl 1.0, "lDirSense"=0) -> (reference out=w1004:refnum<k7>, error out=w1003:errorcluster, "lChanID"=w1002:i32)  [unwired: 1 in, 6 out]
        n456 = invoke class="MG17Motor" method="SetStageAxisInfo"(reference=w1014, error in=w1013, "lChanID"=0, "fMinPos"=w977, "fMaxPos"=w976, "lUnits"=1, "fPitch"=sgl 1.0, "lDirSense"=0) -> (reference out=w999:refnum<k7>, error out=w998:errorcluster, "lChanID"=w997:i32)  [unwired: 1 in, 6 out]
        n457 = invoke class="MG17Motor" method="GetPosition_Position"(reference=w1004, error in=w1003, "lChanID"=w1002) -> (reference out=w996:refnum<k7>, error out=w1006:errorcluster, "GetPosition_Position"=w1005:sgl)  [unwired: 1 in, 1 out]
        n458 = invoke class="MG17Motor" method="GetPosition_Position"(reference=w999, error in=w998, "lChanID"=w997) -> (reference out=w995:refnum<k7>, error out=w1001:errorcluster, "GetPosition_Position"=w1000:sgl)  [unwired: 1 in, 1 out]
        n459 = invoke class="MG17Motor" method="GetPosition_Position"(reference=w1012, error in=w1011, "lChanID"=w1010) -> (reference out=w1009:refnum<k7>, error out=w1008:errorcluster, "GetPosition_Position"=w1007:sgl)  [unwired: 1 in, 1 out]
        n460 = property on="Pos (mm)" class="DigNum (strict)"(error in=w1006, "Value"=w1005) -> (error out=w994:errorcluster)  [unwired: 1 in, 1 out]
        n461 = property on="Pos (mm)" class="DigNum (strict)"(error in=w1001, "Value"=w1000) -> (error out=w992:errorcluster)  [unwired: 1 in, 1 out]
        n462 = property on="Pos (mm)" class="DigNum (strict)"(error in=w1008, "Value"=w1007) -> (error out=w993:errorcluster)  [unwired: 1 in, 1 out]
        n463 = Bundle("Motor Reference"=w1009, "Motor Reference"=w996, "Motor Reference"=w995) -> (w1022:T25)  [unwired: 1 in]
        n464 = Merge Errors(w993, w994, w992) -> (w1023:errorcluster)
        n465 = property on="InstrumentMode" class="Enum (strict)"("Value"=w975) -> ()  [unwired: 2 in, 2 out]
      }
      frame "BasicMode" {
        n466 = call-poly <vilib>:"Acquire Input Data.vi"("device ID"=w1062, "error in (no error)"=w1061) -> ("device ID"=w1060:refnum<k1>, "axis info"=w1056:T26, "button info"=w1046:T27, "error out"=w1048:errorcluster)  [unwired: 13 in, 1 out]
        n467 = call "j_GetJoystickSignal.vi"("RelJoyPos In"=w1058, "NewJoystButtInfo"=w1046, "NewJoystAxisInfo"=w1056, "OldJoystButtInfo"=w1045, "OldJoystickOffset"=w1057) -> ("MoveZ"=→"Move Z":bool, "MoveXY"=→"Move XY":bool, "Joystick Offset"=w1059:T2, "RelJoyPos"=w1053:T3, "TalkToMotors?"=w1050:bool)
        n468 = call "s_TurnTrapsOnOffWithJoystick.vi"("Error In"=w1048, "Shutter Control Reference Cluster"=w1044, "NewJoystButtInfo"=w1046, "OldJoystButtInfo"=w1045) -> ("Error Out"=w1047:errorcluster)  [unwired: 7 in]
        n469 = case shown="True" w1050 {
          tunnel: w1053 -> [w1100 w1104]
          tunnel: [w1089 w1121] -> w1052
          tunnel: w1051 -> [w1099 w1107]
          tunnel: w1047 -> [w1073 w1106]
          tunnel: [w1100 w1104] -> w1049
          frame False {
            # "Just Update Motor Position and Vel"
            n470 = Unbundle(w1099) -> ("Motor Reference"=w1098:refnum<k7>, "Motor Reference"=w1091:refnum<k7>, "Motor Reference"=w1090:refnum<k7>)
            n471 = property on="Pos (mm)" class="DigNum (strict)"(error in=w1073) -> (error out=w1081:errorcluster, "Value"=w1078:sgl)  [unwired: 1 in, 1 out]
            n472 = property on="Pos (mm)" class="DigNum (strict)"(error in=w1073) -> (error out=w1074:errorcluster, "Value"=w1071:sgl)  [unwired: 1 in, 1 out]
            n473 = property on="Pos (mm)" class="DigNum (strict)"(error in=w1073) -> (error out=w1082:errorcluster, "Value"=w1087:sgl)  [unwired: 1 in, 1 out]
            n474 = invoke class="MG17Motor" method="GetPosition_Position"(reference=w1091, error in=w1081, "lChanID"=0) -> (error out=w1094:errorcluster, "GetPosition_Position"=w1079:sgl)  [unwired: 1 in, 2 out]
            n475 = invoke class="MG17Motor" method="GetPosition_Position"(reference=w1090, error in=w1074, "lChanID"=0) -> (error out=w1092:errorcluster, "GetPosition_Position"=w1070:sgl)  [unwired: 1 in, 2 out]
            n476 = property on="MotorLoopDelay" class="DigNum (strict)"() -> ("Value"=w1066:u32)  [unwired: 2 in, 2 out]
            n477 = invoke class="MG17Motor" method="GetPosition_Position"(reference=w1098, error in=w1082, "lChanID"=0) -> (error out=w1096:errorcluster, "GetPosition_Position"=w1088:sgl)  [unwired: 1 in, 2 out]
            n478 = To Single Precision Float(number=w1066) -> (single precision float=w1065:sgl)
            n479 = Subtract(x=w1088, y=w1087) -> (x-y=w1086:sgl)
            n480 = property on="Pos (mm)" class="DigNum (strict)"(error in=w1094, "Value"=w1079) -> (error out=w1077:errorcluster)  [unwired: 1 in, 1 out]
            n481 = Subtract(x=w1079, y=w1078) -> (x-y=w1080:sgl)
            n482 = Subtract(x=w1070, y=w1071) -> (x-y=w1072:sgl)
            n483 = property on="Pos (mm)" class="DigNum (strict)"(error in=w1092, "Value"=w1070) -> (error out=w1069:errorcluster)  [unwired: 1 in, 1 out]
            n484 = property on="Pos (mm)" class="DigNum (strict)"(error in=w1096, "Value"=w1088) -> (error out=w1084:errorcluster)  [unwired: 1 in, 1 out]
            n485 = Divide(x=w1065, y=sgl 1000.0) -> (x/y=w1063:sgl)
            n486 = Divide(x=w1086, y=w1063) -> (x/y=w1085:sgl)
            n487 = Divide(x=w1080, y=w1063) -> (x/y=w1076:sgl)
            n488 = Divide(x=w1072, y=w1063) -> (x/y=w1068:sgl)
            n489 = property on="Vel (mm/s)" class="DigNum (strict)"(error in=w1084, "Value"=w1085) -> (error out=w1083:errorcluster)  [unwired: 1 in, 1 out]
            n490 = property on="Vel (mm/s)" class="DigNum (strict)"(error in=w1077, "Value"=w1076) -> (error out=w1075:errorcluster)  [unwired: 1 in, 1 out]
            n491 = property on="Vel (mm/s)" class="DigNum (strict)"(error in=w1069, "Value"=w1068) -> (error out=w1067:errorcluster)  [unwired: 1 in, 1 out]
            n492 = Merge Errors(w1083, w1075, w1067) -> (w1089:errorcluster)
          }
          frame True {
            # ">ZMotRef>"
            # ">YMotRef>"
            # ">XMotRef>"
            n493 = Unbundle By Name(w1104) -> ("XRelPos"=w1137:i32, "YRelPos"=w1123:i32, "ZRelPos"=w1108:i32)
            n494 = Unbundle(w1107) -> ("Motor Reference"=w1103:refnum<k7>, "Motor Reference"=w1102:refnum<k7>, "Motor Reference"=w1101:refnum<k7>)
            n495 = property on="Direction" class="DigNum (strict)"(error in=w1106) -> (error out=w1136:errorcluster, "Value"=w1135:i32)  [unwired: 1 in, 1 out]
            n496 = property on="Direction" class="DigNum (strict)"(error in=w1106) -> (error out=w1126:errorcluster, "Value"=w1125:i32)  [unwired: 1 in, 1 out]
            n497 = property on="Direction" class="DigNum (strict)"(error in=w1106) -> (error out=w1111:errorcluster, "Value"=w1110:i32)  [unwired: 1 in, 1 out]
            n498 = property on="Move Z" class="Bool (strict)"(error in=w1111) -> (error out=w1119:errorcluster, "Value"=w1118:bool)  [unwired: 1 in, 1 out]
            n499 = property on="Move XY" class="Bool (strict)"(error in=w1136) -> (error out=w1145:errorcluster, "Value"=w1144:bool)  [unwired: 1 in, 1 out]
            n500 = property on="Move XY" class="Bool (strict)"(error in=w1126) -> (error out=w1134:errorcluster, "Value"=w1133:bool)  [unwired: 1 in, 1 out]
            n501 = call "j_MotorExecute.vi"("MoveChamber?"=w1144, "Axis Motor Settings"="X Motor Settings", "Error In"=w1145, "JoystRelPos"=w1137, "Motor's Old Direction"=w1135, "Motor Reference In"=w1103) -> ("Error Out"=w1140:errorcluster, "Motor Position (mm)"=w1139:sgl, "Motor's New Direction"=w1138:i32, "Motor Velocity (mm/s)"=w1141:sgl)  [unwired: 1 out]
            n502 = call "j_MotorExecute.vi"("MoveChamber?"=w1133, "Axis Motor Settings"="Y Motor Settings", "Error In"=w1134, "JoystRelPos"=w1123, "Motor's Old Direction"=w1125, "Motor Reference In"=w1102) -> ("Error Out"=w1129:errorcluster, "Motor Position (mm)"=w1128:sgl, "Motor's New Direction"=w1127:i32, "Motor Velocity (mm/s)"=w1130:sgl)  [unwired: 1 out]
            n503 = call "j_MotorExecute.vi"("MoveChamber?"=w1118, "Axis Motor Settings"="Z Motor Settings", "Error In"=w1119, "JoystRelPos"=w1108, "Motor's Old Direction"=w1110, "Motor Reference In"=w1101) -> ("Error Out"=w1114:errorcluster, "Motor Position (mm)"=w1113:sgl, "Motor's New Direction"=w1112:i32, "Motor Velocity (mm/s)"=w1115:sgl)  [unwired: 1 out]
            n504 = property on="Pos (mm)" class="DigNum (strict)"(error in=w1140, "Value"=w1139) -> (error out=w1142:errorcluster)  [unwired: 1 in, 1 out]
            n505 = property on="Pos (mm)" class="DigNum (strict)"(error in=w1129, "Value"=w1128) -> (error out=w1131:errorcluster)  [unwired: 1 in, 1 out]
            n506 = property on="Pos (mm)" class="DigNum (strict)"(error in=w1114, "Value"=w1113) -> (error out=w1116:errorcluster)  [unwired: 1 in, 1 out]
            n507 = property on="Vel (mm/s)" class="DigNum (strict)"(error in=w1142, "Value"=w1141) -> (error out=w1143:errorcluster)  [unwired: 1 in, 1 out]
            n508 = property on="Vel (mm/s)" class="DigNum (strict)"(error in=w1131, "Value"=w1130) -> (error out=w1132:errorcluster)  [unwired: 1 in, 1 out]
            n509 = property on="Vel (mm/s)" class="DigNum (strict)"(error in=w1116, "Value"=w1115) -> (error out=w1117:errorcluster)  [unwired: 1 in, 1 out]
            n510 = property on="Direction" class="DigNum (strict)"(error in=w1132, "Value"=w1127) -> (error out=w1120:errorcluster)  [unwired: 1 in, 1 out]
            n511 = property on="Direction" class="DigNum (strict)"(error in=w1143, "Value"=w1138) -> (error out=w1122:errorcluster)  [unwired: 1 in, 1 out]
            n512 = property on="Direction" class="DigNum (strict)"(error in=w1117, "Value"=w1112) -> (error out=w1105:errorcluster)  [unwired: 1 in, 1 out]
            n513 = Merge Errors(w1122, w1120, w1105) -> (w1121:errorcluster)
          }
        }
        n514 = property on="InstrumentMode" class="Enum (strict)"() -> ("Value"=w1043:T1)  [unwired: 2 in, 2 out]
      }
      frame "PassiveMode" {
        n515 = property on="InstrumentMode" class="Enum (strict)"() -> ("Value"=w1153:T1)  [unwired: 2 in, 2 out]
      }
      frame "AcquireOffsetMode" {
        n516 = property on="InstrumentMode" class="Enum (strict)"() -> ("Value"=w1160:T1)  [unwired: 2 in, 2 out]
      }
      frame "AcquireSpectrumMode" {
        n517 = property on="InstrumentMode" class="Enum (strict)"() -> ("Value"=w1167:T1)  [unwired: 2 in, 2 out]
      }
      frame "Force-ExtensionMode" {
        n518 = property on="InstrumentMode" class="Enum (strict)"() -> ("Value"=w1174:T1)  [unwired: 2 in, 2 out]
      }
      frame "Shutdown" {
        n519 = call-poly <vilib>:"Close Input Device.vi"("error in (no error)"=w1178, "device ID"=w1177) -> ("error out"=w1186:errorcluster)  [unwired: 8 in]
        n520 = Unbundle(w1179) -> ("Motor Reference"=w1182:refnum<k7>, "Motor Reference"=w1181:refnum<k7>, "Motor Reference"=w1180:refnum<k7>)
        n521 = call "s_CloseMotor.vi"("Error In"=w1186, "Motor Reference In"=w1182) -> ("Error Out"=w1191:errorcluster)
        n522 = call "s_CloseMotor.vi"("Error In"=w1186, "Motor Reference In"=w1181) -> ("Error Out"=w1189:errorcluster)
        n523 = call "s_CloseMotor.vi"("Error In"=w1186, "Motor Reference In"=w1180) -> ("Error Out"=w1187:errorcluster)
        n524 = property on="IsActive?" class="Bool (strict)"(error in=w1191, "Value"=FALSE ("IsYMotorActive?")) -> (error out=w1185:errorcluster)  [unwired: 1 in, 1 out]
        n525 = property on="IsActive?" class="Bool (strict)"(error in=w1189, "Value"=FALSE ("IsYMotorActive?")) -> (error out=w1184:errorcluster)  [unwired: 1 in, 1 out]
        n526 = property on="IsActive?" class="Bool (strict)"(error in=w1187, "Value"=FALSE ("IsYMotorActive?")) -> (error out=w1183:errorcluster)  [unwired: 1 in, 1 out]
        n527 = Merge Errors(w1185, w1184, w1183) -> (w1176:errorcluster)
        n528 = property on="InstrumentMode" class="Enum (strict)"(error in=w1176) -> (error out=w1175:errorcluster, "Value"=w1193:T1)  [unwired: 1 in, 1 out]
      }
    }
  }
  n529 = Merge Errors(w1, w5, w7) -> (w3:errorcluster)
  n530 = call <vilib>:"General Error Handler.vi"("type of dialog (OK msg:1)"=w2, "error in (no error)"=w3) -> ()  [unwired: 9 in, 5 out]
